vi "Main control_v2.13.vi"() -> ()   [LabVIEW 2015]
panel:
  out "millisecond timer value":u32
  in  "Snap Number Counting":dbl=49.0
  out "Movie Point cluster":cluster{"Movie Y":dbl[], "Movie X":dbl[]}={"Movie Y"=[-12.0, -12.0, -12.0, 0.323, 0.323, 0.323, 0.323, 0.323, 0.3734, 0.3734, 0.3734, 0.3734, 0.3734, 0.3734, 0.3734, 0.3734, 0.3734, 0.3734, 0.8702, 0.8702, 0.8702, 0.8702, 0.8702, 0.8702, 1.1907, 1.1907, 1.1907, 1.1907, 1.1907, 1.1782, 1.1782, 1.1782, 1.1782, 1.1782, 1.1782, 1.1782, 1.1782, 0.273, 0.273, 0.273, 2.5485, 2.5485, 2.5485, 2.5485], "Movie X"=[-1.0, -1.0, -1.0, 4.5272, 4.5272, 4.5272, 4.5272, 4.5272, 5.9944, 5.9944, 5.9944, 5.9944, 5.9944, 5.9944, 5.9944, 5.9944, 5.9944, 5.9944, 5.5544, 5.5544, 5.5544, 5.5544, 5.5544, 5.5544, 5.661, 5.661, 5.661, 5.661, 5.661, 6.0676, 6.0676, 6.0676, 6.0676, 6.0676, 6.0676, 6.0676, 6.0676, 5.2601, 5.2601, 5.2601, 2.0517, 2.0517, 2.0517, 2.0517]}
  out "Movie Point  Y Array":dbl[](array[numeric])=[-12.0, -12.0, -12.0, 0.323, 0.323, 0.323, 0.323, 0.323, 0.3734, 0.3734, 0.3734, 0.3734, 0.3734, 0.3734, 0.3734, 0.3734, 0.3734, 0.3734, 0.8702, 0.8702, 0.8702, 0.8702, 0.8702, 0.8702, 1.1907, 1.1907, 1.1907, 1.1907, 1.1907, 1.1782, 1.1782, 1.1782, 1.1782, 1.1782, 1.1782, 1.1782, 1.1782, 0.273, 0.273, 0.273, 2.5485, 2.5485, 2.5485, 2.5485]
  out "Movie Point  X Array":dbl[](array[numeric])=[-1.0, -1.0, -1.0, 4.5272, 4.5272, 4.5272, 4.5272, 4.5272, 5.9944, 5.9944, 5.9944, 5.9944, 5.9944, 5.9944, 5.9944, 5.9944, 5.9944, 5.9944, 5.5544, 5.5544, 5.5544, 5.5544, 5.5544, 5.5544, 5.661, 5.661, 5.661, 5.661, 5.661, 6.0676, 6.0676, 6.0676, 6.0676, 6.0676, 6.0676, 6.0676, 6.0676, 5.2601, 5.2601, 5.2601, 2.0517, 2.0517, 2.0517, 2.0517]
  out "Snap Point cluster":cluster{"Snap Y":dbl[], "Snap X":dbl[]}={"Snap Y"=[-12.0, 0.323, 0.8702, 1.1907, 2.5485], "Snap X"=[-1.0, 4.5272, 5.5544, 5.661, 2.0517]}
  out "Snap Point  Y Array":dbl[](array[numeric])=[-12.0, 0.323, 0.8702, 1.1907, 2.5485]
  out "Snap Point  X Array":dbl[](array[numeric])=[-1.0, 4.5272, 5.5544, 5.661, 2.0517]
  out "Stage XY Cluster":cluster{"Stage Y ":dbl[], "Stage X":dbl[]}
  in  "Previous Light control":T1={"Filter Set"=0, "Lasers DO"=[FALSE, FALSE, FALSE, FALSE, FALSE, FALSE], "Lasers AO (V)"=[0.3, 0.3, 0.3, 0.3, 0.3, 0.3], "LED"=FALSE, "Global"=FALSE} {"Lasers AO (V)" min=0.0 max=5.0 step=0.01 scale=0.0..5.0 scale format="%#1.2f"; "Filter Set" items=["R-QuasAr", "R-Cy5", "R-mCherry", "R-mOrange", "R-GFP", "R-CFP/DAPI", "R-BFP", "R-LED", "SDC-Cy5", "SDC-mCherry", "SDC-mO2", "SDC-GFP", "SDC-CFP/DAPI", "SDC-BFP", "SDC-LED"]}
  out "Image Info":T2={"Status"="Camera live", "scale bar (μm)"=65.0, "Image"=array512x512[262144 elements], "Histogram"={"max value"=6837, "mean"=2967, "min value"=1682, "Histogram"={"X Values"=[1707.775, 1759.325, 1810.875, 1862.425, 1913.975, 1965.5249999999999, 2017.0749999999998, 2068.625, 2120.175, 2171.7250000000004, 2223.2750000000005, 2274.8250000000007, 2326.375000000001, 2377.925000000001, 2429.4750000000013, 2481.0250000000015, 2532.5750000000016, 2584.125000000002, 2635.675000000002, 2687.225000000002, 2738.7750000000024, 2790.3250000000025, 2841.8750000000027, 2893.425000000003, 2944.975000000003, 2996.5250000000033, 3048.0750000000035, 3099.6250000000036, 3151.175000000004, 3202.725000000004, 3254.275000000004, 3305.8250000000044, 3357.3750000000045, 3408.9250000000047, 3460.475000000005, 3512.025000000005, 3563.5750000000053, 3615.1250000000055, 3666.6750000000056, 3718.225000000006, 3769.775000000006, 3821.325000000006, 3872.8750000000064, 3924.4250000000065, 3975.9750000000067, 4027.525000000007, 4079.075000000007, 4130.625000000007, 4182.1750000000075, 4233.725000000008, 4285.275000000008, 4336.825000000008, 4388.375000000008, 4439.925000000008, 4491.475000000009, 4543.025000000009, 4594.575000000009, 4646.125000000009, 4697.675000000009, 4749.2250000000095, 4800.77500000001, 4852.32500000001, 4903.87500000001, 4955.42500000001, 5006.97500000001, 5058.525000000011, 5110.075000000011, 5161.625000000011, 5213.175000000011, 5264.725000000011, 5316.2750000000115, 5367.825000000012, 5419.375000000012, 5470.925000000012, 5522.475000000012, 5574.025000000012, 5625.575000000013, 5677.125000000013, 5728.675000000013, 5780.225000000013, 5831.775000000013, 5883.3250000000135, 5934.875000000014, 5986.425000000014, 6037.975000000014, 6089.525000000014, 6141.075000000014, 6192.625000000015, 6244.175000000015, 6295.725000000015, 6347.275000000015, 6398.825000000015, 6450.3750000000155, 6501.925000000016, 6553.475000000016, 6605.025000000016, 6656.575000000016, 6708.125000000016, 6759.675000000017, 6811.225000000017], "Histogram: h(x)"=[41, 1173, 7166, 18548, 38399, 52796, 41857, 18688, 5319, 2347, 1597, 1341, 1106, 993, 836, 742, 658, 618, 542, 497, 461, 457, 375, 411, 351, 350, 349, 333, 306, 267, 290, 314, 267, 266, 245, 236, 239, 226, 215, 236, 207, 198, 220, 203, 183, 203, 193, 233, 207, 201, 200, 213, 225, 205, 234, 233, 217, 223, 226, 234, 205, 188, 191, 179, 188, 151, 157, 160, 126, 106, 88, 73, 65, 45, 58, 56, 47, 62, 59, 57, 75, 127, 241, 563, 1192, 2513, 4244, 6503, 8198, 8910, 8047, 6139, 3870, 2034, 948, 358, 135, 51, 13, 6]}}, "Scale Info"={"Pixel size (nm)"=650.0, "Total x width (μm)"=332.8, "Total y width (μm)"=332.8}, "Camera View indicator"=array512x512[262144 elements], "max frame rate (Hz)"=100.0}
  out "log path":path=path "C:/Register info of scope/201810 regiser info.txt"
  out "ROI cursor":T3={"Bin"=4, "ROI"={"x offset"=0, "y offset"=0, "x width"=512, "y width"=512}} caption="ROI" {"ROI"."x offset" min=1 max=512 step=1; "ROI"."y offset" min=1 max=512 step=1; "ROI"."x width" min=1 max=512 step=1; "ROI"."y width" min=1 max=512 step=1; "Bin" items=["1x1"=1, "2x2"=2, "4x4"=4]}
  out "Previous ROI":T3={"Bin"=4, "ROI"={"x offset"=0, "y offset"=0, "x width"=512, "y width"=512}} caption="ROI" {"ROI"."x offset" min=1 max=512 step=1; "ROI"."y offset" min=1 max=512 step=1; "ROI"."x width" min=1 max=512 step=1; "ROI"."y width" min=1 max=512 step=1; "Bin" items=["1x1"=1, "2x2"=2, "4x4"=4]}
  in  "Tab":T4(tab)
  in  "Load Excel to table":bool
  in  "Write table to excel":bool
  in  "Goto destination":bool
  in  "Clear Table":bool
  in  "Track on?":bool
  in  "Stage on?":bool
  out "SDC initialized":bool
  in  "Confocal on?":bool
  in  "Camera on?":bool
  out "Stage initialized":bool
  out "Camera initialized":bool[](array[boolean])
  in  "Light control":T1={"Filter Set"=7, "Lasers DO"=[FALSE, FALSE, FALSE, FALSE, FALSE, FALSE], "Lasers AO (V)"=[0.3, 0.3, 0.3, 0.3, 0.3, 0.3], "LED"=TRUE, "Global"=FALSE} {"Lasers AO (V)" min=0.2 max=5.0 step=0.01 scale=0.0..5.0 scale format="%#1.2f"; "Filter Set" items=["R-QuasAr", "R-Cy5", "R-mCherry", "R-mOrange", "R-GFP", "R-CFP/DAPI", "R-BFP", "R-LED", "SDC-Cy5", "SDC-mCherry", "SDC-mO2", "SDC-GFP", "SDC-CFP/DAPI", "SDC-BFP", "SDC-LED", "SDC-Cy3", "R-pHlamingo", "R-dualview", "R-mO2_no laser"]}
  in  "Confocal scanner":T5={"SDC shutter"=FALSE, "Filter wheel"=6, "FW speed"=3, "Disk spinning"=FALSE, "Disk speed (rpm)"=3000.0} {"Disk speed (rpm)" min=1500.0 max=10000.0; "FW speed" min=1 max=5 step=1; "Filter wheel" items=["CFP"=1, "GFP"=2, "mCherry"=3, "Alexa-647"=4, "OFP"=5, "empty"=6]}
  in  "Stage-Ctrl":T6={"Console"={"L"=FALSE, "R"=FALSE, "FWD"=FALSE, "BACK"=FALSE}, "Step Width [mm]"=0.2, "Destination [mm]"=[0.0, 0.0], "Move "=FALSE} {"Destination [mm]" format="%_6g"; "Step Width [mm]" min=0.0 format="%_6f"}
  out "Stage Status":T7={" Current Position"=[-1.0, -12.0, 0.0], "Number of Axis"=3, "ILSID"=1}
  in  "Camera Ctrl":T8={"Chosen Camera"=1, "ROI selection"=0, "Live"=FALSE, "ROI define"=FALSE, "Snap"=FALSE, "ROI update"=FALSE, "ROI previous "=FALSE, "ROI"={"Bin"=4, "ROI"={"x offset"=0, "y offset"=0, "x width"=512, "y width"=512}}, "Exposure (ms)"=100.0, "Symmetrical"=TRUE, "Autoscale"=TRUE, "Scale"={"Scale.Min"=374, "Scale.Max"=483}} {"Scale"."Scale.Max" min=1 max=5000 step=1; "Scale"."Scale.Min" min=1 max=5000 step=1; "Exposure (ms)" min=1.0 max=5000.0 step=1.0; "ROI"."ROI"."x offset" min=1 max=512 step=1; "ROI"."ROI"."y offset" min=1 max=512 step=1; "ROI"."ROI"."x width" min=1 max=512 step=1; "ROI"."ROI"."y width" min=1 max=512 step=1; "ROI"."Bin" items=["1x1"=1, "2x2"=2, "4x4"=4]; "ROI selection" items=["Full ROI", "Central quad", "Confocal", "Patch 500", "Patch 1000", "Patch 484", "Patch 484 full X", "Line scan 2.5KHz", "Confocal_2", "patch 1000 wide", "patch 671", "DV2"]; "Chosen Camera" items=["Left", "Right"]}
  in  "TI-Ctrl":T9={"Obj"=2, "Cube Bottom"=4, "Cube Top"=6, "PFS-Ctrl"={"PFS IO"=FALSE, "PSF Err"=FALSE, "PSF Pos"=0}, "Z-Ctrl"={"Z-pos"=500.85, "Home"=FALSE, "Sensitivity"=1}, "Condenser"=2, "Lightpath"=enum."R100"} {"Condenser" items=["A"=1, "DICN2"=2, "- empty 3 -"=3, "- empty 4 -"=4, "- empty 5 -"=5, "- empty 6 -"=6]; "Z-Ctrl"."Sensitivity" min=1 max=3 step=1 scale=1.0..3.0; "PFS-Ctrl"."PSF Pos" scale=0.0..16400.0; "Cube Top" items=["Quad-O"=1, "Quad-R"=2, "empty"=3, "empty"=4, "empty"=5, "DIC"=6]; "Cube Bottom" items=["GFP"=1, "RFP"=2, "mO2"=3, "empty"=4, "CFP"=5, "Cy5"=6]; "Obj" items=["20x/.75 Dry PFS"=1, "40x/1.3 Oil PFS"=2, "60x/1.4 Oil PFS"=3, "- empty 4 -"=4, "- empty 5 -"=5, "40x/0.6 Dry PFS"=6]}
  in  "Scope on?":bool
  out "Ti-E initialized":bool
  in  "stop program":bool
  in  "Record Table":string[][](table)=[["", "", "", "", ""], ["", "", "", "", ""], ["", "", "", "", ""], ["", "", "", "", ""], ["", "", "", "", ""], ["", "", "", "", ""], ["", "", "", "", ""], ["", "", "", "", ""], ["", "", "", "", ""], ["", "", "", "", ""], ["", "", "", "", ""], ["", "", "", "", ""], ["", "", "", "", ""], ["", "", "", "", ""], ["", "", "", "", ""], ["", "", "", "", ""], ["", "", "", "", ""], ["", "", "", "", ""], ["", "", "", "", ""], ["", "", "", "", ""], ["", "", "", "", ""], ["", "", "", "", ""], ["", "", "", "", ""], ["", "", "", "", ""], ["", "", "", "", ""], ["", "", "", "", ""], ["", "", "", "", ""], ["", "", "", "", ""], ["", "", "", "", ""], ["", "", "", "", ""], ["", "", "", "", ""], ["", "", "", "", ""], ["", "", "", "", ""], ["", "", "", "", ""], ["", "", "", "", ""], ["", "", "", "", ""], ["", "", "", "", ""], ["", "", "", "", ""], ["", "", "", "", ""], ["", "", "", "", ""], ["", "", "", "", ""], ["", "", "", "", ""], ["", "", "", "", ""], ["", "", "", "", ""], ["", "", "", "", ""], ["46", "01/25 18:48:27", "-1.0000", "-12.0000", "Movie"], ["47", "01/25 18:49:17", "-1.0000", "-12.0000", "Movie"], ["48", "01/25 20:04:01", "-1.0000", "-12.0000", "Movie"], ["49", "05/17 17:14:13", "-1.0000", "-12.0000", "Image"]]
  out "Stage Trajec":cluster{"Value":dbl[], "Value":dbl[]}[](graph)=[{"Value"=[], "Value"=[]}, {"Value"=[-12.0, 0.323, 0.8702, 1.1907, 2.5485], "Value"=[-1.0, 4.5272, 5.5544, 5.661, 2.0517]}, {"Value"=[-12.0, -12.0, -12.0, 0.323, 0.323, 0.323, 0.323, 0.323, 0.3734, 0.3734, 0.3734, 0.3734, 0.3734, 0.3734, 0.3734, 0.3734, 0.3734, 0.3734, 0.8702, 0.8702, 0.8702, 0.8702, 0.8702, 0.8702, 1.1907, 1.1907, 1.1907, 1.1907, 1.1907, 1.1782, 1.1782, 1.1782, 1.1782, 1.1782, 1.1782, 1.1782, 1.1782, 0.273, 0.273, 0.273, 2.5485, 2.5485, 2.5485, 2.5485], "Value"=[-1.0, -1.0, -1.0, 4.5272, 4.5272, 4.5272, 4.5272, 4.5272, 5.9944, 5.9944, 5.9944, 5.9944, 5.9944, 5.9944, 5.9944, 5.9944, 5.9944, 5.9944, 5.5544, 5.5544, 5.5544, 5.5544, 5.5544, 5.5544, 5.661, 5.661, 5.661, 5.661, 5.661, 6.0676, 6.0676, 6.0676, 6.0676, 6.0676, 6.0676, 6.0676, 6.0676, 5.2601, 5.2601, 5.2601, 2.0517, 2.0517, 2.0517, 2.0517]}]
  in  "Number":dbl
  out "Color Acquiring":bool
  out "T Acquired Progress":i32(slide)=100 scale=0.0..100.0
  in  "Load from Exel (For XY Scan)":bool
  in  "Load from table (For XY Scan)":bool
  in  "Generate Tiling":bool
  in  "XY Scan List":string[][](table)
  in  "Cal step num":bool
  in  "Cal step size":bool
  in  "Define 1":bool
  in  "Define 2":bool
  in  "Z-Stack":T10={"Z end"=1000.0, "Step Num"=10, "Step Size"=-200.0, "Z0"=3000.0, "z-stack?"=FALSE}
  in  "MD acquisition":bool
  in  "Channel settings":T11={"Take?"=[FALSE, TRUE, FALSE, FALSE], "Channel"=[1, 2, 3, 4], "Exposure time (msec)"=[100.0, 100.0, 100.0, 100.0], "Cumulation"=[1, 1, 1, 1], "Name"=["Cy5", "mCh", "GFO", "CFP"]} {"Exposure time (msec)" format="%0.0f"; "Channel" items=["R-QuasAr", "R-Cy5", "R-mCherry", "R-mOrange", "R-GFP", "R-CFP/DAPI", "R-BFP", "R-LED", "SDC-Cy5", "SDC-mCherry", "SDC-mO2", "SDC-GFP", "SDC-CFP/DAPI", "SDC-BFP", "SDC-LED", "SDC-Cy3", "R-pHlamingo"]}
  in  "Period (s)":u32=3
  in  "Timelapse Cycles":i32=100 caption="# Cycles"
  in  "Timelapse?":bool
  out "Timelapse Acquired":i32=100 caption="Acquired"
  out "Timelapse Time (s)":dbl=297.037 caption="Time (s)"
  in  "Movie frame rate (Hz)":dbl=10.0 format="%0.0f"
  out "Frames Recorded":i32=1000
  in  "Stream movie":bool
  in  "# frames":i32=1000
  in  "Total time (sec)":dbl=100.0 min=1.0 max=5000.0 step=1.0
  out "Elapsed time (sec)":dbl=100.541 min=1.0 max=5000.0 step=1.0
  in  "Base folder":path=path "C:/Users/ZouOptics/Desktop/test"
  in  "Sub-folder":string="patch"
  out "Full path":path=path "C:/Users/ZouOptics/Desktop/test/200401_patch"
  in  "XY tiling":T12={"Tiling?"=FALSE, "YY/XX"=[1, 1], "X0Y0"=[-1.0, -12.0, 0.0]}
  in  "Excel Loading Path":path=path "X:/Data and analysis/Sicong Wang/Fluorescence Images/test.xlsx"
  out "Z Stack Aquired":i32(slide)=10 scale=0.0..1.0
  out "Stage Trajec for tiling":cluster{"Value":dbl[], "Value":dbl[]}[](graph)
  in  "Ranking":u16(ring) items=["Identical", "Minimum Distance", "Snake"]
  in  "Waveform channels":T13={"Lasers"=[FALSE, TRUE, FALSE, TRUE, FALSE, FALSE], "Patch"=FALSE, "Camera Output"=TRUE}
  out "Lasers DO waveform":digitalwaveform[](graph)=[{"t0"=timestamp(0 s since 1904-01-01), "dt"=0.001, "Y"={"transitions"=[0, 10000, 13000, 19999], "data"=[[0], [1], [0], [0]]}}, {"t0"=timestamp(0 s since 1904-01-01), "dt"=0.001, "Y"={"transitions"=[0, 10000, 19999], "data"=[[1], [0], [0]]}}]
  out "Lasers AO waveform":waveform(dbl)[](graph)=[{"t0"=timestamp(0 s since 1904-01-01), "dt"=0.001, "Y"=array[20000 elements]}, {"t0"=timestamp(0 s since 1904-01-01), "dt"=0.001, "Y"=array[20000 elements]}]
  in  "Load waveform":bool
  in  "Waveform info":T14={"Waveform folder"=path "C:/Users/ZouOptics/Desktop/MATLAB codes new/MATLAB codes/ephys waveforms_new/Mito and ER/dual-color/waveform003_561_3s 3min test", "Exposure time (ms)"=200.0} {"Exposure time (ms)" format="%0.5f"}
  out "AI Waveform":cluster{"xo":i32, dbl, "data":dbl[][]}(graph)={"xo"=0, 0.001, "data"=[]}
  in  "Run waveform":bool
  out "Patch Ex. Command AO waveform":waveform(dbl)(graph)
  out "Seal test DAQ params":T15={"samples"=40000, "Duration (sec)"=2.2222222222222223, "Downsampling factor"=2000.0}
  out "Patch seal test waveform":waveform(dbl)(graph)={"t0"=timestamp(0 s since 1904-01-01), "dt"=5.555555555555556e-05, "Y"=array[40000 elements]}
  in  "Save patch param":bool
  in  "Pipet tuning parameters":T16={"Amplitude (mV)"=5.0, "Number of repeats"=20, "DAQ rate (Hz)"=18000.0, "Frequency (Hz)"=9.0}
  in  "Test patch":bool
  out "Patch output":cluster{"xo":i32, dbl, "data":dbl[][]}(graph)={"xo"=0, 5.555555555555556e-05, "data"=array2x40000[80000 elements]}
  out "Average I-t curve":cluster{"xo":i32, dbl, dbl[]}(graph)={"xo"=0, 5.555555555555556e-05, [29.880051543579523, 31.53110578210508, 83.18090907512509, 162.0368645993861, 229.6898135163709, 288.6606341781445, 343.08904187423104, 388.8031046956136, 432.56006420735736, 429.5156789314345, 389.7776239991212, 355.78201712503267, 329.13964160904936, 306.7416838810265, 288.4109564887366, 272.60916075180677, 258.4745269911103, 245.11307022374868, 234.37719239460748, 224.51919115018714, 215.35382740090955, 206.6636454502011, 199.34263011111548, 192.6498209835887, 186.06976642635385, 179.43333449516217, 174.21439286866243, 168.7377258559817, 163.79261775420784, 158.65421491547735, 154.4661750789392, 150.4794835552285, 146.3397675650155, 141.9987034936742, 139.3731246948087, 136.7636538843144, 133.12328092961516, 130.39300120942653, 127.58218215818046, 125.35124577902424, 122.21826996530297, 119.06918641850369, 117.3456469811447, 115.89594095422709, 114.10797017306047, 111.50655329307857, 109.57361178840823, 107.18965080041876, 105.35335650344665, 102.92912592909049, 102.10762590319547, 101.1008856426019, 100.06192974722902, 98.96659640362893, 97.00143950529804, 95.9946992448826, 94.87520399068636, 93.32885099805317, 91.07375276207976, 89.26967425849605, 88.464282088203, 87.36894864979442, 86.14475245555671, 84.88028669189909, 83.79300728992337, 82.64129641270459, 82.10168356131484, 81.30434527026028, 80.03987957079214, 80.11236480548284, 79.13784014631288, 78.29217829154415, 77.06798205802154, 75.22363383162443, 74.1766240107049, 74.00749150960763, 73.31485423356304, 73.04907478387904, 71.53493743348268, 71.22888838598573, 71.19667263278379, 70.03690780108447, 69.72280488470987, 69.42480969761857, 68.67579487408646, 68.2892065594221, 68.2650448000469, 67.53213783229249, 66.21129465198342, 65.04347590641633, 64.47970136823793, 63.738740585923004, 63.31188273674811, 63.06221124272047, 63.247451399716546, 62.50649048668514, 61.548073809976344, 61.5722356830505, 61.773583749751516, 61.29034841296893, 60.30776992217408, 59.252706103313066, 58.970818812926204, 59.7117796957233, 59.5345934070801, 58.45536777888253, 57.56138251425965, 56.96539234266666, 56.38550986897839, 55.6042793899474, 55.20158318736758, 55.282122384674594, 55.443200858403316, 54.97607337010223, 54.621700717145416, 54.90358802777563, 54.35592129460591, 53.42972030928748, 54.372029148842316, 53.49415159115674, 53.20421033522031, 52.2457936059895, 52.1733082482847, 52.03639155042868, 51.22294539942853, 51.79477386875771, 50.97327375999859, 51.118244339124836, 50.498092398621225, 50.820249284974935, 50.5142002256432, 49.22557270943183, 49.096709956802705, 49.41081292650386, 48.790660927446204, 48.72622958625065, 49.563837544108324, 49.71686213809168, 49.233626722017284, 48.492665888390036, 48.782607126502214, 47.62284235318299, 48.218832605660864, 48.44434242434597, 47.075175695308104, 46.94631299135462, 47.759759177278106, 46.56777864142779, 46.61610214009233, 46.18119035155284, 45.99595015189401, 45.5207686921585, 45.14223428471252, 45.383851918860685, 45.810709817016004, 45.214719602674585, 44.32073419846522, 43.990523364405924, 44.844239111123336, 45.64157743347831, 44.455050003834835, 42.9998909052363, 43.475072280525744, 43.7730674181327, 44.04690079066772, 42.99989087004219, 43.08848400218545, 42.66968004658263, 42.85492020248559, 42.981182076403115, 42.49249376565697, 42.532763411615534, 42.33946927737113, 42.017312373726895, 41.727371189308236, 42.548871213651026, 42.78243503281226, 41.815964370657404, 41.67099377457743, 40.74479272430971, 41.33272903397758, 41.73542518986539, 40.68841531947955, 40.68036138479713, 40.66425355122241, 41.67099382135634, 40.7689545273035, 40.62398400796506, 40.124640818844185, 39.83469956321526, 40.29377314835857, 39.923292709326375, 39.69778287373534, 40.09242502006745, 40.1165867506579, 39.66556710850734, 39.02385421340008, 38.449424886197086, 39.10179251143014, 39.907184658568255, 40.317934715770775, 39.82664548999167, 39.593081728282165, 39.58502783256104, 39.45616501104882, 39.480326789591686, 39.97966992283737, 39.81053760662116, 38.83601302550602, 38.505802172044845, 38.22391489382652, 39.144662908881884, 39.11790028828071, 38.417209103882385, 39.09373859598984, 38.71520425745377, 38.44942479293209, 38.64271891646013, 38.256130738306, 37.780949304210154, 37.99035129543478, 37.23328257384945, 37.692356207891606, 37.78094938449001, 37.72457190122881, 37.57154738570286, 38.00645923224989, 37.5312778137379, 37.87759644612147, 37.90981213503523, 37.84538073068071, 38.15948368901419, 38.39304737004068, 38.18364539082346, 37.716517944756625, 37.305767891483846, 36.62923834581099, 36.830586380562174, 36.28291974002178, 36.62923835578246, 36.99971871503225, 37.24133642280873, 37.67624822587764, 35.888277488077094, 36.52453727615889, 37.82121877366858, 37.080257998223054, 36.677561870857566, 35.63055195367037, 36.47621377440903, 36.556752962450304, 36.817079377736675, 35.87216966309211, 35.45336570834543, 35.75136084508183, 35.77552256150283, 36.06546377068963, 36.21848834436996, 35.831900084497946, 36.64534623485339, 36.49232172114825, 36.049356061223044, 35.86411580752019, 36.31773634513554, 36.38762076053971, 36.162110948839185, 35.1714785375557, 35.80228530827381, 36.221089318174705, 36.05740998819331, 36.234596259515136, 35.131208907727846, 35.93660112849782, 36.98361098547167, 36.41983640610623, 35.63055202080656, 35.70303727905714, 36.05740981623031, 35.92854705422721, 35.35671863758792, 35.686929417746775, 36.02519411870366, 36.04130196862305, 35.80513734973099, 35.853460911422225, 35.11510086032629, 34.656027278390894, 34.478840946772294, 34.57548806003412, 35.1527696265201, 36.00103227632688, 35.30034103329851, 34.53521850111496, 34.865429279655665, 35.6627675893214, 36.685615730073295, 35.703037251838076, 34.054584022453355, 35.68953027356607, 35.83995400784085, 35.2439637863511, 35.04261567853634, 34.56198119625272, 34.79814587027351, 34.970130472238445, 35.01040010245213, 34.67473618343048, 34.73916762344858, 35.24656475502339, 35.13380981144574, 34.124468602443265, 34.41701062047655, 34.61835868531181, 35.22240285144073, 35.0023460751858, 35.211748027071806, 34.23722340304511, 33.826473384960565, 34.58354206554848, 33.227882236903135, 33.10707340456224, 33.823872504398196, 33.81036547173107, 33.38090675630988, 33.268151809626936, 33.260097906803445, 33.42117637060354, 34.17019112956772, 34.79839701045026, 34.98363723051565, 33.89090473781439, 32.51368406091628, 33.48820861717215, 34.0680910149931, 32.4305439113784, 32.88961752023779, 33.47755388152356, 33.32713026373934, 33.35129198579972, 32.85740184312288, 34.50845598814005, 33.576801900497294, 34.28814790525812, 33.29491457286375, 33.77814996396535, 34.084199078645284, 34.272040140362186, 33.23308420063638, 33.60356458985568, 33.98469978568426, 33.79685868804102, 33.98209888749632, 33.353892963877016, 33.28686075071024, 33.10707355187398, 32.89767152720865, 33.539133089710276, 33.49886349447493, 33.55264005260219, 33.78905597985785, 33.93117437541065, 34.18084601030195, 32.916380133871534, 32.2559585132527, 32.58616932156536, 33.21177438100168, 33.576801728530626, 33.52847818346761, 33.77814984665877, 33.63863227243345, 33.778149832967486, 34.97818427338362, 34.680189157321486, 33.75944114678964, 33.93117436078832, 33.82387255658079, 33.34063724504784, 33.061350832666015, 32.33649783263258, 32.86000283828841, 32.46536067034913, 32.70957917530949, 32.87611066749775, 32.60227733217256, 33.431831332440225, 33.20632151462504, 32.67736351117674, 32.63709392257487, 33.015628287713305, 33.86934405322023, 32.99952040978686, 33.50691746633257, 33.03458822506665, 33.2923137505889, 33.25464502047356, 32.857401940524845, 33.13383614177684, 32.7230860846945, 33.51782354473178, 33.16865260615072, 33.25464488004037, 33.81036555020686, 34.156684233437915, 32.97821065828864, 32.86000265489926, 32.70697814823967, 32.972757554955756, 32.51108314372694, 32.7929704134161, 33.12032905957902, 32.27466722926702, 32.19412805134144, 31.896132920558067, 33.70826546725869, 33.89090476099264, 33.69761065497293, 33.190213613064564, 33.20632142585998, 32.98601334906449, 32.741794880060795, 32.28817436835036, 31.7646694066269, 32.50823109621544, 32.46796151596167, 31.340412406565125, 31.03436337556969, 31.56852313913503, 32.1403515811195, 32.63969476829801, 32.5485007324532, 32.30688307985144, 32.03304972077633, 32.53499374600606, 32.36065966647435, 32.59942512105814, 32.196980288638684, 31.635806586574443, 31.235711320411408, 32.306882974958725, 32.15125757030716, 31.944456465814945, 31.82104673328156, 31.77272321662366, 32.26946549432704, 32.23724981873913, 31.737906623218368, 31.853262418874255, 32.24790456433751, 32.34195074938029, 32.280120284066754, 31.517598539524357, 30.65582887774616, 30.81975955493944, 31.619698723654817, 31.104247722579014, 30.9351153357554, 32.213088086020925, 31.456019436396677, 31.73790676935194, 32.75270098238981, 32.607730407576675, 31.41574989477592, 31.531105711919206, 31.18478704877367, 30.919007585808018, 31.587483151770833, 31.12840961645485, 31.179334033517204, 30.35523306530969, 31.16607837413623, 31.689583307138683, 32.108387280662065, 31.44796563489925, 31.665421495347566, 32.74464701592463, 32.30168130493072, 32.143203734291866, 32.07071842025991, 31.50434292991561, 32.01434091344282, 32.304282138445515, 31.555267359288916, 31.61164479053598, 31.772723234375118, 31.73245361272506, 32.03850264630772, 31.866769372738997, 31.133862486566013, 31.378080986518274, 31.43445846323188, 31.297541794396263, 31.007600642087446, 31.426404609191703, 31.305595773656705, 32.47341445327548, 31.68958317094127, 31.708291949137532, 31.571375276751702, 31.41029680286774, 31.735054573538918, 31.40224294857394, 32.25855958429945, 32.12709595526592, 32.014341055350485, 32.548500821840065, 31.563321429034854, 32.06266464659797, 31.557868392452068, 31.735054666392447, 32.06786634854822, 32.21829000105026, 31.43445864129108, 30.90550055484247, 31.565922199383742, 32.74439577108956, 32.80622627683914, 31.603590937293813, 31.227657404087406, 31.33235844208331, 31.72439980138405, 32.20763509026013, 30.97538496036247, 31.265326158285603, 30.910953532773906, 31.44796545801619, 31.70569100495986, 31.25727220550966, 30.68544366007619, 31.69763699291113, 32.5568058683679, 30.967331024342286, 31.257272228962393, 31.461221169015328, 31.51759864918303, 31.99823311270946, 31.684130142679276, 30.516311463134777, 29.914868169545862, 30.9779858757755, 31.99823312580485, 30.508257520275055, 31.348466316509402, 31.54721343780208, 31.89353212832518, 31.635806689247424, 31.888079136450628, 31.710892859029546, 32.46796154145252, 32.20218214144233, 31.531105730372392, 31.799485974142833, 31.896133044845413, 31.549814385193596, 31.633205796520286, 31.638658809288323, 33.034588244313646, 32.811679271974256, 32.63994604569917, 32.62383813951148, 31.947308642051155, 31.882877272238257, 31.705691012757082, 31.59553694057632, 31.0639780411176, 32.245303741456134, 31.327156646376245, 31.98497738706063, 31.754014493314706, 32.75815391380303, 31.756615378639385, 31.512396844714164, 31.3674262422325, 32.77140960429028, 31.533957751273974, 30.77688911611326, 31.456019463499782, 31.657367500176907, 31.778176318456836, 31.893532131794363, 31.327156735270798, 30.540473205208805, 30.06529184371326, 30.951223310518714, 30.894845837431127, 31.096193885174088, 30.637120368779996, 31.7243998764309, 31.257272371463607, 31.788831245688037, 31.28948811045239, 32.135149885863015, 32.172818584434474, 31.286887102411967, 31.810392069406326, 31.713745016952483, 31.57137528962488, 30.908352738668093, 31.327156703970836, 31.402242833385337, 31.563321255214674, 31.724399686599444, 32.24790466817393, 32.164764616467565, 30.983438868015334, 30.725713302903657, 31.845208507857382, 32.90572538454016, 32.680215511032365, 31.69763699732868, 31.635806530539316, 32.39287522201038, 32.24245161694785, 32.1834733143828, 32.46536063396243, 33.11772828602879, 32.45730665126147, 32.078772309469485, 31.40224285401661, 31.57942916481285, 31.20349572746602, 31.450566465836673, 31.32975760514152, 31.200894856826146, 32.296228336044614, 31.281434118783995, 30.878737999785105, 30.580742902576137, 31.68673114847933, 33.01562831400659, 31.131010466554596, 30.631667235535073, 31.496289125427666, 31.614245797440212, 31.211549671241873, 31.370027177893874, 30.991492850089656, 30.833015316745822, 31.24376532947516, 31.692184034043294, 30.572688825384922, 31.5552673754126, 31.217002640458894, 30.96733103585858, 31.434458503688436, 31.659968271830152, 32.11904192419194, 31.120355544607026, 30.830414336323074, 30.564634884949417, 30.95122310879727, 31.966017358462167, 31.47732895837401, 30.148431847342014, 30.446426980577804, 30.94577015502743, 31.023708412930922, 31.80493890640768, 30.972532773535328, 31.713493666093385, 32.25855949492659, 31.95251043134216, 31.85326252525323, 31.756615505137205, 31.549814382487217, 31.020856402695518, 31.979273100828895, 32.39002319769506, 31.90418701928753, 32.36586145638116, 31.84235650087687, 32.06526542756272, 30.628815052346862, 29.839782002889855, 31.077233852323314, 32.13229763381895, 32.02499571929181, 29.941630711558663, 29.925522915681533, 29.91486810586367, 30.28820071066647, 30.798198666447885, 29.815620191529806, 30.258585876990605, 31.12035556143148, 30.545926225824854, 30.352632087120078, 31.21440175147005, 31.36482536311301, 30.801050802731506, 31.429256736566643, 31.520450751781844, 30.862630039038468, 31.324304499306724, 31.278833159463602, 30.956676254443614, 30.3604347147787, 30.476041848199696, 30.894845809018012, 30.701551671752554, 30.999546815003757, 31.24116453355479, 32.465360708866044, 32.20763519921539, 31.76727034656866, 31.4451134538732, 31.72700076064497, 30.824961454822606, 30.76053008060773, 31.3001428842445, 31.286635957481643, 31.018255638184936, 31.710892845150802, 31.54721353543418, 31.82910086033523, 31.4692751855601, 31.72960156848901, 31.61424578852162, 31.55786830228545, 31.434458571204658, 30.516311420978596, 30.476041797680725, 30.629066321367187, 30.733767290196383, 30.451880022493715, 29.65194086011632, 30.368739961190006, 30.39550254159804, 29.23313682270737, 30.368739862372074, 31.026560691792298, 31.023708509804553, 31.888079024195022, 31.415498550014895, 31.51499780331629, 30.784691725345446, 29.957989912879217, 30.473440956633922, 31.045269456235964, 30.333672123238326, 29.85588982023964, 30.073345767800177, 30.207410243685274, 30.921608483815014, 29.98995440320599, 30.51891240020253, 31.455768218895308, 31.81559387622767, 31.815593882283984, 30.932263310215863, 31.17128009201948, 32.234397788879974, 31.010201633812333, 31.356520264265857, 31.649313626879547, 32.03044881971146, 31.375480236579005, 31.061377280971858, 31.286635736595215, 30.725713337528504, 31.11775467351705, 31.273380076138007, 31.426404587227502, 31.16867905851295, 30.862630000857155, 30.81430646152824, 31.434458454174607, 30.919007421203926, 30.83041426930373, 30.760529811808027, 30.639721029031293, 30.497351315332885, 31.042417142920748, 31.576576862282476, 31.802086771755153, 31.163226034858297, 31.434458539901552, 31.831701628300063, 30.704152537353597, 30.26663987115451, 30.59685068241315, 30.935115403309197, 30.994093738597435, 31.13101047335675, 29.885253409888595, 30.69064560512269, 31.6571162794837, 31.718946822468943, 30.84367014287102, 31.334959407307114, 32.309484016428925, 31.997981895589806, 31.24921839735877, 31.316250660405387, 31.504091714639518, 31.31885149341779, 30.27729465851637, 31.316250610730435, 31.297541854155217, 31.74570932861524, 30.86523088628539, 31.007600607971025, 31.179333876255754, 30.800799517191457, 30.741821192127794, 30.54592616862937, 31.104247680473215, 31.788831082376014, 31.783378025132098, 30.851975215476774, 30.365887672508354, 30.476041756270966, 30.82756216299985, 31.56046904668177, 32.05981230246551, 31.15517211759733, 31.249218328323703, 30.693497699573225, 30.097507435948625, 31.394188871726715, 30.526966219048095, 29.71897311446653, 31.06397815885712, 30.902899699950478, 30.025022174032827, 29.912267285168575, 30.34717913403877, 29.592711336450922, 29.506719012104046, 30.52696631479477, 30.328219104807474, 30.594249854926087, 30.50565668876932, 30.910953669575182, 31.292340216785878, 31.90158606541657, 30.83846834299569, 31.47472819085728, 31.06943114529891, 31.555267375178683, 31.15257125475, 31.152571236122316, 30.73922032685906, 30.4438260962654, 30.097507394514306, 30.465386966695327, 30.65868110266879, 30.45733306260895, 30.715058585676303, 30.908352699865382, 31.0317623644851, 30.900298765572398, 30.540473145533497, 31.64386047438833, 30.226370196123653, 30.328470367039458, 30.178046702743913, 31.684130129933784, 31.38613500513597, 30.119068410694847, 30.583343710082143, 30.49735145483496, 31.198042662156247, 31.22505669951251, 31.30274374127294, 31.326905528954132, 32.62358699616382, 32.11618989103248, 31.50409184549359, 31.560469251446197, 31.83975567319857, 31.082686970538155, 30.51891238925412, 30.78729266941014, 31.098794773824803, 31.823647750627856, 30.357833871748657, 29.88525333248012, 31.122956480936736, 31.332358484811667, 30.18064757398678, 29.643886974725834, 29.87199765914472, 30.580742811847994, 30.242478044568006, 30.91095356758006, 30.38484772028895, 30.664134121345576, 29.99020551564751, 29.97149677764961, 30.760781181089612, 29.81016705878638, 29.92552289823385, 30.94031707674453, 30.784691652032432, 30.897446617439208, 30.577890634454963, 29.952536889890304, 29.68675743323106, 30.39290172749185, 30.400955672851023, 29.78340454552243, 31.023708580818, 30.398103518369282, 29.383309306915507, 29.694811402401267, 29.19806912103426, 29.689358424338295, 30.263787758332427, 30.71220652952314, 30.505656731183127, 29.99825962923186, 30.725713420318137, 30.23702502470289, 30.011515276599383, 29.313676253034696, 30.145831032122537, 30.548527090833915, 30.650627267976194, 29.437085864190102, 29.297568285526683, 30.121669222761223, 30.467987853632795, 31.748561437058765, 30.355232915444972, 29.756641812719355, 30.38484771031607, 30.935115297572047, 30.57268877968259, 29.598164183607203, 29.54984064495232, 30.234424079699664, 30.411610382671917, 30.132323956261548, 29.055950579773217, 29.968644702536775, 30.61035761548154, 30.457333052694707, 30.578141935818294, 29.933576855493047, 29.598164341679603, 30.24247813231346, 30.237025048291827, 29.603366100870506, 29.587258253062178, 30.752476186866865, 30.376542653985073, 30.328219138044766, 30.70675352766904, 30.875885853142567, 31.251819323134317, 31.05307209489085, 30.100108369400296, 30.242478130987276, 31.579429207528584, 30.465387066590555, 30.36588778766559, 30.688044641234868, 30.218316291768947, 30.99149281941957, 29.332384797535045, 29.300169096758832, 30.250531908373873, 29.936428947409006, 29.82367404783354, 31.00499978308015, 31.206347778490027, 30.64517405374463, 30.988891874451113, 30.46798779128403, 30.046582983070873, 30.462534742357736, 30.7122063872844, 29.45579451175222, 29.00737572075709, 30.9940936394729, 31.195441722935506, 30.49214966993508, 29.69481138318175, 30.188701502252982, 30.269240719057212, 29.662595666793226, 30.02502222200787, 29.823674167948187, 30.132324080321702, 30.245079031228556, 30.196755523816226, 29.51477300648566, 29.939029987192416, 30.81690750522429, 30.58334373538448, 30.20480941376228, 30.494750608848882, 29.952536916967993, 29.501517270797315, 29.273155228096407, 29.020882729501672, 29.904213316044252, 29.743134889524367, 30.116216128197355, 29.68415651199726]}
  out "Patch quality":T17={"Ra (MΩ)"=24.853031315565314, "Rm (MΩ)"=165.59219608794982, "Cm (pF)"=76.83727869217161, "RC constant (msec)"=1.9096392935393605, "Steady state current (pA)"=30.194659640508572}
  in  "Path of saving register":path=path "C:/Register info of scope"
  in  "Calibrate stage":bool
  in  "Hardware Settings":T18={"DAQ ports"={"Lasers DO lines"=["Dev2/port0/line0", "Dev2/port0/line1", "Dev2/port0/line2", "Dev2/port0/line3", "Dev2/port0/line4", "Dev2/port0/line5"], "Lasers AO lines"=["Dev2/ao0", "Dev2/ao1", "Dev2/ao2", "Dev2/ao3", "Dev2/ao4", "Dev2/ao5"], "Patch AO line"="Dev1/ao1", "Patch AI lines 1"={"Patch scaled output"="Dev1/ai13", "Patch 10 V_m "="Dev1/ai8"}, "Camera timing DI"="Dev1/port0/line23", "Dev1 timing DO "="Dev1/port0/line18", "Dev1 trigger source"="/Dev1/PFI0", "Dev2 trigger source"="/Dev2/PFI0", "LED line"="Dev1/port0/line8", "Global Shutter line"="Dev1/port0/line10", "Patch AI lines 2"={"Cell capacitance"="Dev1/ai9", "Mode"="Dev1/ai10", "Frequency"="Dev1/ai11", "Gain"="Dev1/ai12"}}, "Camera Setting"={"Camera Output triger mode setiting"={"Mode"=3, "Polarity"=2, "Period"=0.0005, "Delay"=0.0}, "Camera timing port for trigering"=enum."3"}, "Stage setting"={"Baudrate"=57600, "COM Port"="COM10", "Xmax"=118.5, "Xmin"=15.0, "Ymax"=76.5, "Ymin"=12.2}, "Confocal VISA Setting"="COM1"} {"Camera Setting"."Camera Output triger mode setiting"."Polarity" items=["Negative"=1, "Positive"=2]; "Camera Setting"."Camera Output triger mode setiting"."Mode" items=["Low"=1, "Global Exposure"=2, "Programmable"=3, "Trigger Ready"=4, "High"=5]}
  out "Camera":errorcluster
  out "Stage":errorcluster
  out "Confocal":errorcluster
  out "Camera Info":T19={"Camera Details Array"=[{"Model"="C11440-22C", "Camera ID"="S/N: 003223", "Firmware"="3.20.A"}], "Handle"=0, "Camera in use "={"Model"="C11440-22C", "Camera ID"="S/N: 003223", "Bits"=16}}
  out "Confocal Info":T20
  in  "Ti Control Lib":refnum<k7>
  out "TiE Ref":T21 caption="Ref (can be hidden)"
  out "Previous Bin":u16(ring)=1 caption="Cursor Bin" items=["1x1"=1, "2x2"=2, "4x4"=4]
  # "Nikon Scope v2.13"
  # "Red"
  # "637"
  # "561"
  # "488"
  # "405"
  # "532"
  # "Camera"
  # "Left Camera"
  # "Right Camera"
  # "Stage"
  # "DON'T Close the window \nuntil this button turns RED!"
  # "Stage Status"
  # "Confocal Scanner"
  # "Nikon control"
  # "Red"
  # "637"
  # "561"
  # "488"
  # "405"
  # "532"
  # "X"
  # "Y"
  # "X"
  # "Y"
  # "File I/O"
  # "Multidimensional acquisition"
  # "Stream"
  # "1. Timelapse"
  # "2. Channel"
  # "grey out at start up"
  # "3. XY Scan"
  # "4. Z-stack"
  # "Need to add tiling function"
  # "X"
  # "Y"
  # "Load waveform"
  # "637"
  # "561"
  # "532"
  # "488"
  # "405"
  # "Red"
  # "Pipet tuning"
  # "Need to restart the program if these settings are changed."
  # "Trigger source: /Dev1/PFI0= right camera (default);\n                           /Dev1/PFI8= left camera"
  # "637"
  # "561"
  # "532"
  # "488"
  # "405"
  # "Red"
  # "Camera information"
  # "Confocal Status"
  # "Power calibration (2017-02-09) Confocal mode\nLaser\t     Voltage\t   mW\n405nm     1             1.22\n488nm\t    1\t            2.90    \n532nm\t    1\t            4.76    \n561nm\t    1\t            4.47       \n637nm\t   \t1             9.95"
  # "Low gain = 100mV/nA\nWith external set to div10,\nthis means DAQ 1mV = 1 pA"
  # "When updating filter set information, please edit:\nsubDAQ_SetFilterSet.vi"
  # "Global shutter mode : 4"
  # "Minimum AO for all lasers: 0.2 V"
  # "Frame        DAQ rate       Exposure\nrate (Hz)       (Hz)            time (ms)\n986.1          9681.46         1.03290\n1058          21159.48        0.9452"
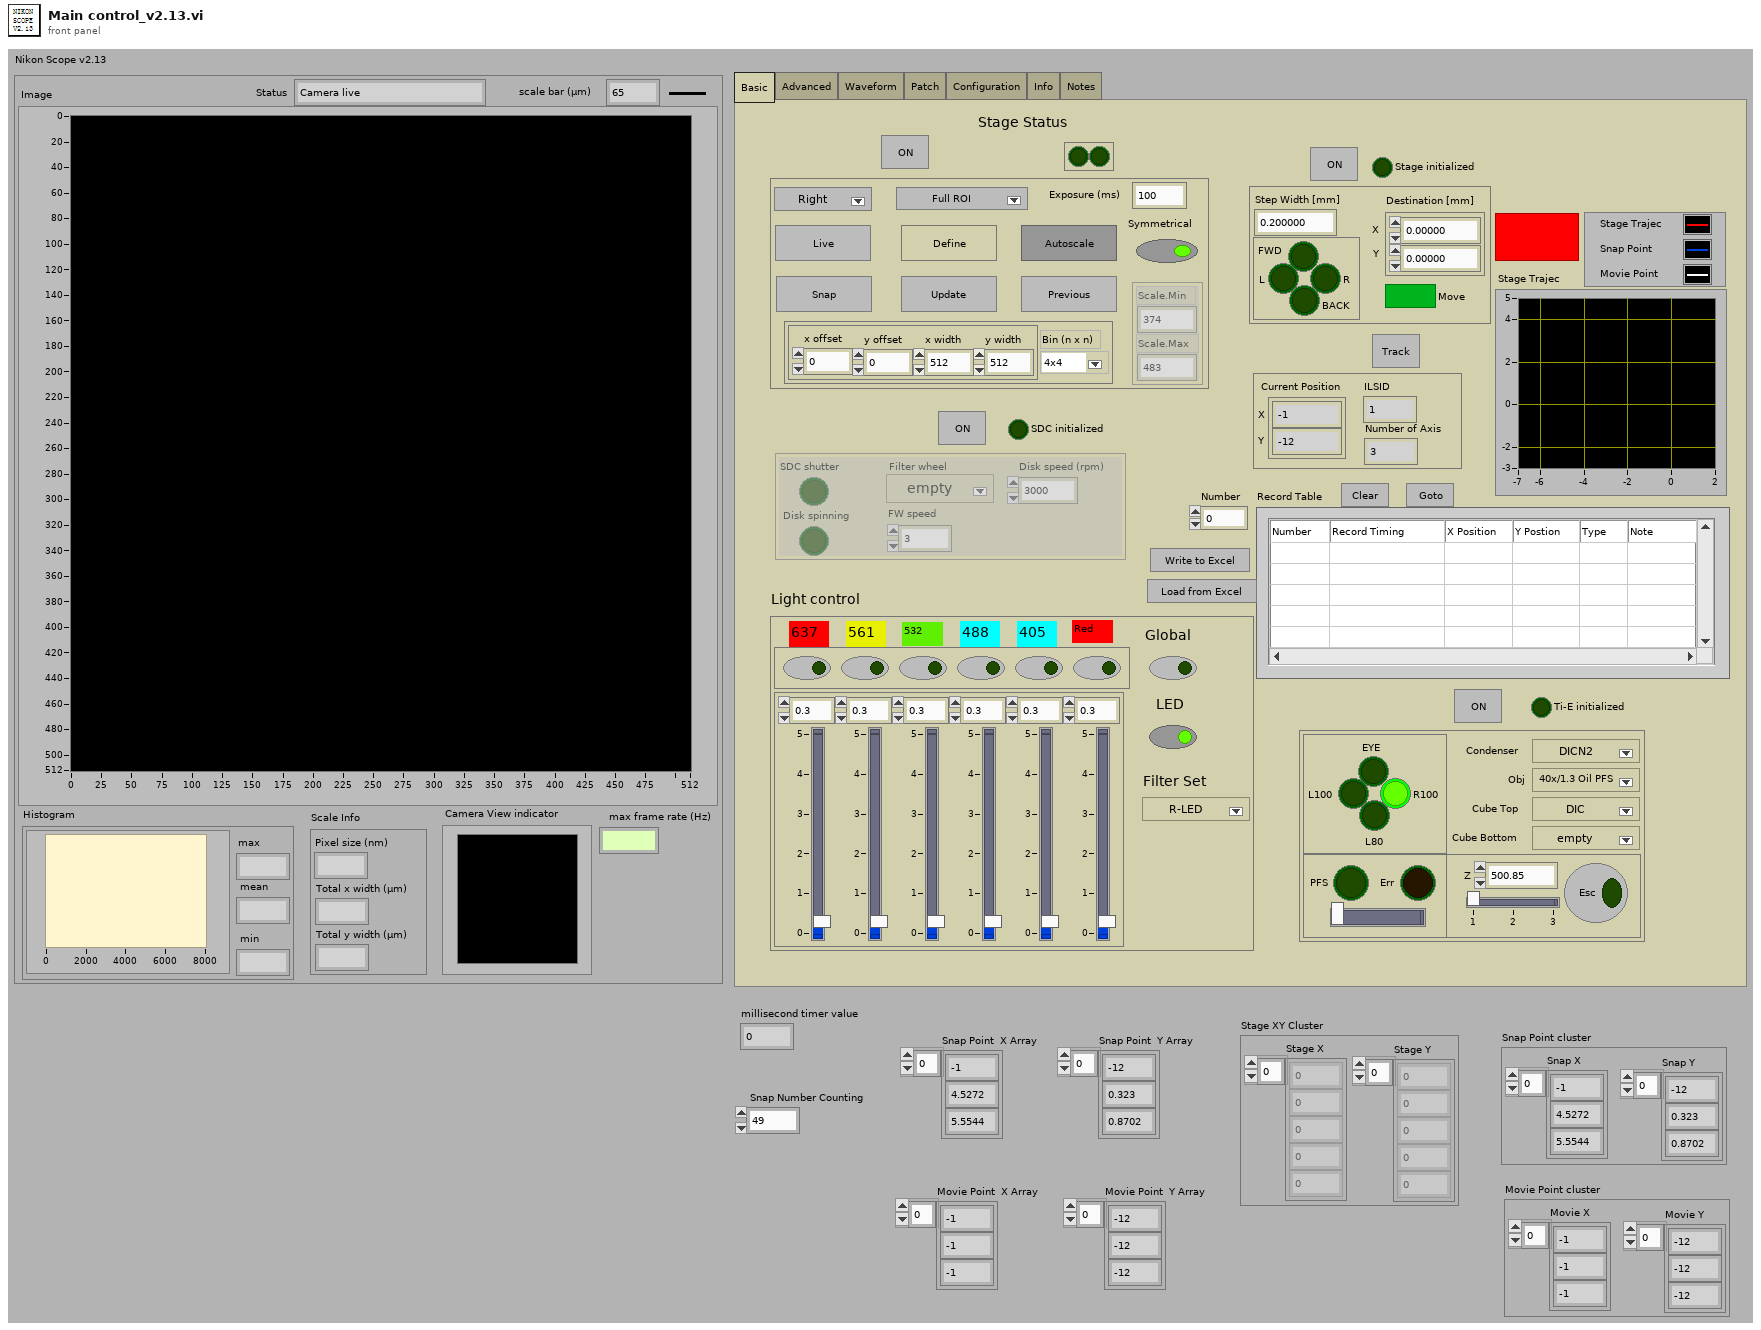
[diagram p1: front panel]
types:
  T1 = cluster{"Filter Set":i32, "Lasers DO":bool[], "Lasers AO (V)":dbl[], "LED":bool, "Global":bool}
  T2 = cluster{"Status":string, "scale bar (μm)":dbl, "Image":u16[][], "Histogram":cluster{"max value":u16, "mean":i16, "min value":u16, "Histogram":cluster{"X Values":dbl[], "Histogram: h(x)":i32[]}}, "Scale Info":cluster{"Pixel size (nm)":dbl, "Total x width (μm)":dbl, "Total y width (μm)":dbl}, "Camera View indicator":u16[][], "max frame rate (Hz)":dbl}
  T3 = cluster{"Bin":u16, "ROI":cluster{"x offset":i32, "y offset":i32, "x width":i32, "y width":i32}}
  T4 = enum32{"Basic", "Advanced", "Waveform", "Patch", "Configuration", "Info", "Notes"}
  T5 = cluster{"SDC shutter":bool, "Filter wheel":u16, "FW speed":i32, "Disk spinning":bool, "Disk speed (rpm)":dbl}
  T6 = cluster{"Console":cluster{"L":bool, "R":bool, "FWD":bool, "BACK":bool}, "Step Width [mm]":dbl, "Destination [mm]":dbl[], "Move ":bool}
  T7 = cluster{" Current Position":dbl[], "Number of Axis":i32, "ILSID":i32}
  T8 = cluster{"Chosen Camera":u32, "ROI selection":u16, "Live":bool, "ROI define":bool, "Snap":bool, "ROI update":bool, "ROI previous ":bool, "ROI":cluster{"Bin":u16, "ROI":cluster{"x offset":i32, "y offset":i32, "x width":i32, "y width":i32}}, "Exposure (ms)":dbl, "Symmetrical":bool, "Autoscale":bool, "Scale":cluster{"Scale.Min":i32, "Scale.Max":i32}}
  T9 = cluster{"Obj":u16, "Cube Bottom":u16, "Cube Top":u16, "PFS-Ctrl":cluster{"PFS IO":bool, "PSF Err":bool, "PSF Pos":u32}, "Z-Ctrl":cluster{"Z-pos":dbl, "Home":bool, "Sensitivity":u8}, "Condenser":u16, "Lightpath":enum32{"EYE", "L100", "R100", "L80"}}
  T10 = cluster{"Z end":dbl, "Step Num":i32, "Step Size":dbl, "Z0":dbl, "z-stack?":bool}
  T11 = cluster{"Take?":bool[], "Channel":i32[], "Exposure time (msec)":dbl[], "Cumulation":i32[], "Name":string[]}
  T12 = cluster{"Tiling?":bool, "YY/XX":i32[], "X0Y0":dbl[]}
  T13 = cluster{"Lasers":bool[], "Patch":bool, "Camera Output":bool}
  T14 = cluster{"Waveform folder":path, "Exposure time (ms)":dbl}
  T15 = cluster{"samples":i32, "Duration (sec)":dbl, "Downsampling factor":dbl}
  T16 = cluster{"Amplitude (mV)":dbl, "Number of repeats":i32, "DAQ rate (Hz)":dbl, "Frequency (Hz)":dbl}
  T17 = cluster{"Ra (MΩ)":dbl, "Rm (MΩ)":dbl, "Cm (pF)":dbl, "RC constant (msec)":dbl, "Steady state current (pA)":dbl}
  T18 = cluster{"DAQ ports":cluster{"Lasers DO lines":tag[], "Lasers AO lines":tag[], "Patch AO line":tag, "Patch AI lines 1":cluster{"Patch scaled output":tag, "Patch 10 V_m ":tag}, "Camera timing DI":tag, "Dev1 timing DO ":tag, "Dev1 trigger source":tag, "Dev2 trigger source":tag, "LED line":tag, "Global Shutter line":tag, "Patch AI lines 2":cluster{"Cell capacitance":tag, "Mode":tag, "Frequency":tag, "Gain":tag}}, "Camera Setting":cluster{"Camera Output triger mode setiting":cluster{"Mode":u32, "Polarity":u32, "Period":dbl, "Delay":dbl}, "Camera timing port for trigering":enum16{"1", "2", "3"}}, "Stage setting":cluster{"Baudrate":i32, "COM Port":string, "Xmax":dbl, "Xmin":dbl, "Ymax":dbl, "Ymin":dbl}, "Confocal VISA Setting":refnum<visa-resource-name>}
  T19 = cluster{"Camera Details Array":cluster{"Model":string, "Camera ID":string, "Firmware":string}[], "Handle":u32, "Camera in use ":cluster{"Model":string, "Camera ID":string, "Bits":i32}}
  T20 = cluster{"Actual Disk speed (rpm)":string, "Actual FW speed (rpm)":i32}
  T21 = cluster{"TI":refnum<k7>, "Nosepiece":refnum<k7>, "LightPathDrive":refnum<k7>, "ZDrive":refnum<k7>, "PFS":refnum<k7>, "CondenserCassette":refnum<k7>, "FilterBlockCassette1":refnum<k7>, "FilterBlockCassette2":refnum<k7>}
  T22 = cluster{"width":u32, "height":u32, "datatype":u32}
  T23 = enum8{"Enabled", "Disabled", "Disabled and Grayed Out"}
  T24 = cluster{"SDC shutter":bool, "FWPosition":i32, "FW speed":i32, "Disk spinning?":bool, "Disk speed (rpm)":dbl}
  T25 = cluster{"Lasers DO lines":tag[], "Lasers AO lines":tag[], "Patch AO line":tag, "Patch AI lines 1":cluster{"Patch scaled output":tag, "Patch 10 V_m ":tag}, "Camera timing DI":tag, "Dev1 timing DO ":tag, "Dev1 trigger source":tag, "Dev2 trigger source":tag, "LED line":tag, "Global Shutter line":tag, "Patch AI lines 2":cluster{"Cell capacitance":tag, "Mode":tag, "Frequency":tag, "Gain":tag}}
  T26 = cluster{"Baudrate":i32, "COM Port":string, "Xmax":dbl, "Xmin":dbl, "Ymax":dbl, "Ymin":dbl}
  T27 = cluster{"LEFT":bool, "RIGHT":bool, "FWD":bool, "BACK":bool}
  T28 = cluster{"Total x width (μm)":refnum<vi>, "Total y width (μm)":refnum<vi>, "Pixel size (nm)":refnum<vi>, "scale bar (μm)":refnum<vi>}
  T29 = cluster{"Ra (Mohm)":dbl, "Rm (Mohm)":dbl, "Cm (pF)":dbl, "RC constant (msec)":dbl, "Steady state current (pA)":dbl}
  T30 = cluster{"max value":u16, "mean":i16, "min value":u16, "Histogram":cluster{"X Values":dbl[], "Histogram: h(x)":i32[]}}
  T31 = cluster{"Camera Output triger mode setiting":cluster{"Mode":u32, "Polarity":u32, "Period":dbl, "Delay":dbl}, "Camera timing port for trigering":enum16{"1", "2", "3"}}
  T32 = cluster{"Model":string, "Camera ID":string, "Bits":i32}
  T33 = cluster{"Lasers DO lines":tag[], "Lasers AO lines":tag[], "Patch AO line":tag, "Patch AI lines":tag[], "Dev1 timing DO":tag, "Camera timing DI":tag, "Dev1 trigger source":tag, "Dev2 trigger source":tag}
  T34 = cluster{"Sampling rate (Hz)":dbl, "dt (sec)":dbl, "total time (sec)":dbl, "# samples":i32, "Exposure time (ms)":dbl, "# frames":i32}
  T35 = cluster{"TI-Ctrl":refnum<vi>, "TiE Ref":cluster{"TI":refnum<k7>, "Nosepiece":refnum<k7>, "LightPathDrive":refnum<k7>, "ZDrive":refnum<k7>, "PFS":refnum<k7>, "CondenserCassette":refnum<k7>, "FilterBlockCassette1":refnum<k7>, "FilterBlockCassette2":refnum<k7>}}
  T36 = cluster{"Filter Set":i32, "Light control":refnum<vi>, "Confocal scanner":refnum<vi>, "Value":cluster{"Lasers DO lines":tag[], "Lasers AO lines":tag[], "Patch AO line":tag, "Patch AI lines 1":cluster{"Patch scaled output":tag, "Patch 10 V_m ":tag}, "Camera timing DI":tag, "Dev1 timing DO ":tag, "Dev1 trigger source":tag, "Dev2 trigger source":tag, "LED line":tag, "Global Shutter line":tag, "Patch AI lines 2":cluster{"Cell capacitance":tag, "Mode":tag, "Frequency":tag, "Gain":tag}}, "Value":refnum<visa-resource-name>}
  T37 = cluster{"XY tiling":cluster{"Tiling?":bool, "YY/XX":i32[], "X0Y0":dbl[]}, "Stage Status":refnum<vi>}
  T38 = cluster{i32, "appended path":path, "Z-Stack":cluster{"Z end":dbl, "Step Num":i32, "Step Size":dbl, "Z0":dbl, "z-stack?":bool}, "Arch_Dragon cumulation":i32, "Image Info":refnum<vi>, "Camera Ctrl":cluster{"Chosen Camera":u32, "ROI selection":u16, "Live":bool, "ROI define":bool, "Snap":bool, "ROI update":bool, "ROI previous ":bool, "ROI":cluster{"Bin":u16, "ROI":cluster{"x offset":i32, "y offset":i32, "x width":i32, "y width":i32}}, "Exposure (ms)":dbl, "Symmetrical":bool, "Autoscale":bool, "Scale":cluster{"Scale.Min":i32, "Scale.Max":i32}}}
  T39 = cluster{"NewVal":i32, "Light control":refnum<vi>, "Confocal scanner":refnum<vi>, "Value":cluster{"Lasers DO lines":tag[], "Lasers AO lines":tag[], "Patch AO line":tag, "Patch AI lines 1":cluster{"Patch scaled output":tag, "Patch 10 V_m ":tag}, "Camera timing DI":tag, "Dev1 timing DO ":tag, "Dev1 trigger source":tag, "Dev2 trigger source":tag, "LED line":tag, "Global Shutter line":tag, "Patch AI lines 2":cluster{"Cell capacitance":tag, "Mode":tag, "Frequency":tag, "Gain":tag}}, "Value":refnum<visa-resource-name>}
  T40 = cluster{"Obj":u16, "Cube 1":u16, "Cube 2":u16, "PFS-Ctrl":cluster{"PFS IO":bool, "PSF Err":bool, "PSF Pos":u32}, "Z-Ctrl":cluster{"Z-pos":dbl, "Home":bool, "Sensitivity":u8}, "Condenser":u16, "Lightpath":enum32{"EYE", "L100", "R100", "L80"}}
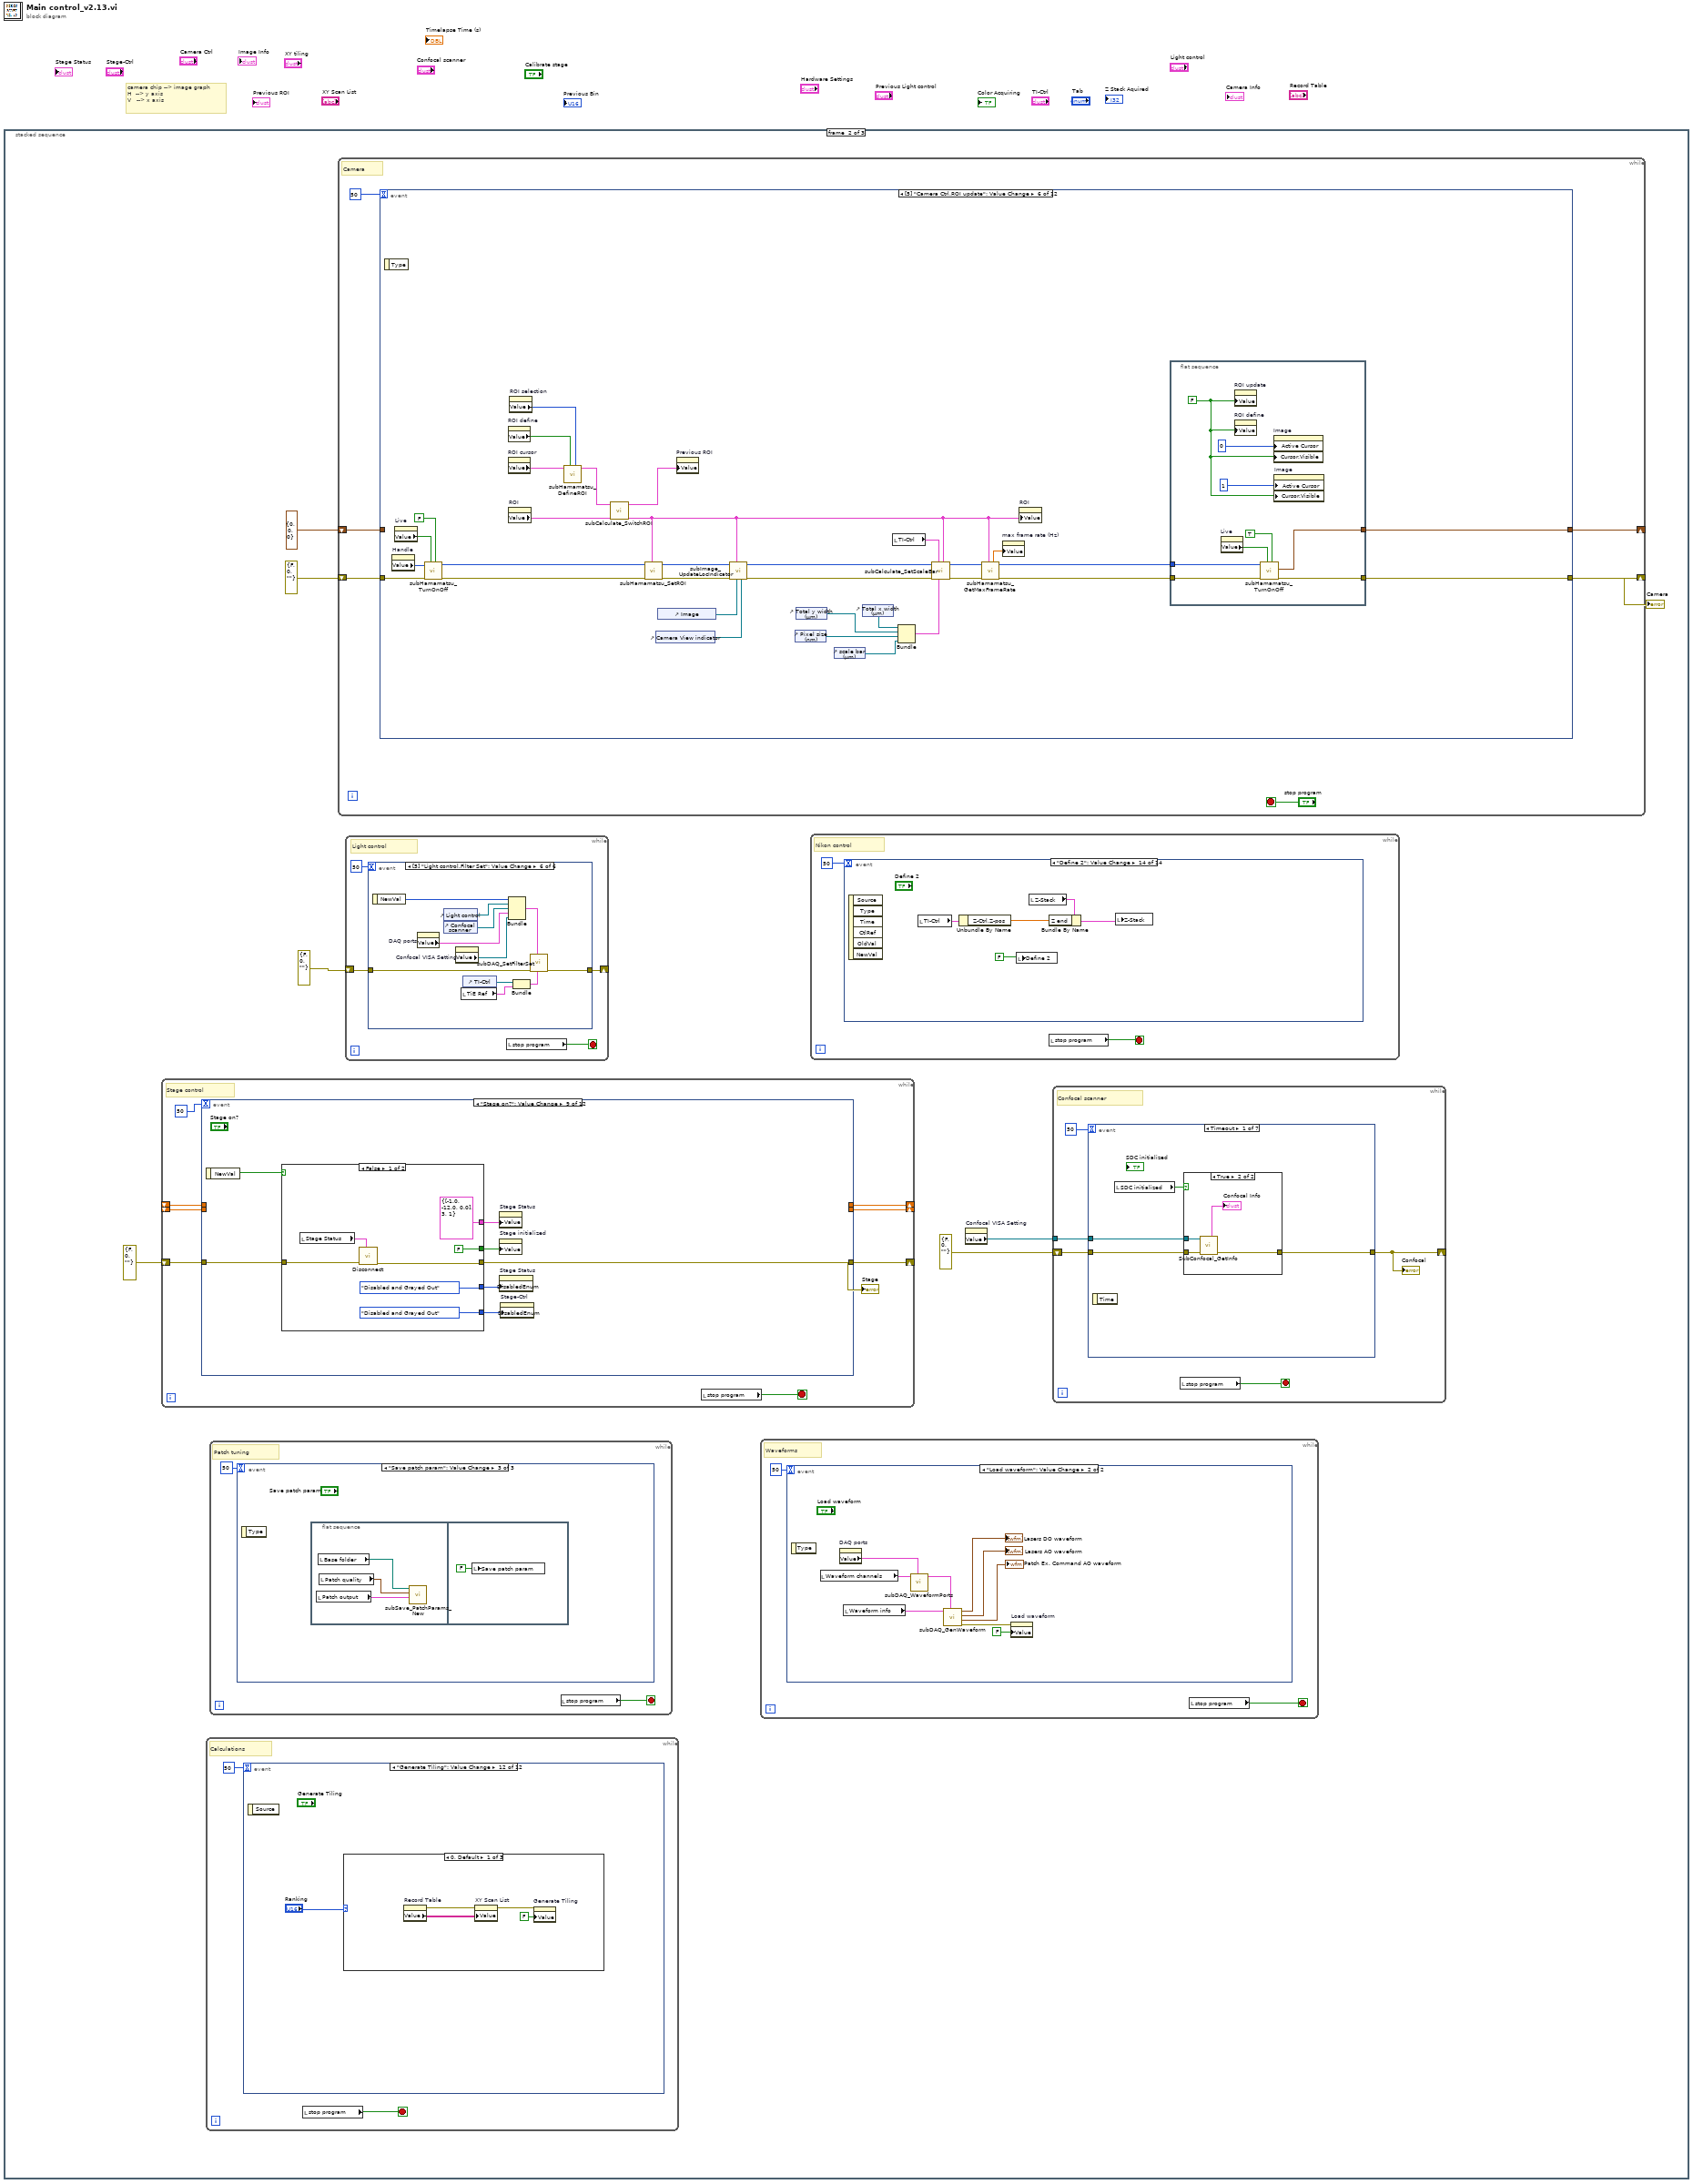
[diagram p0: block diagram]
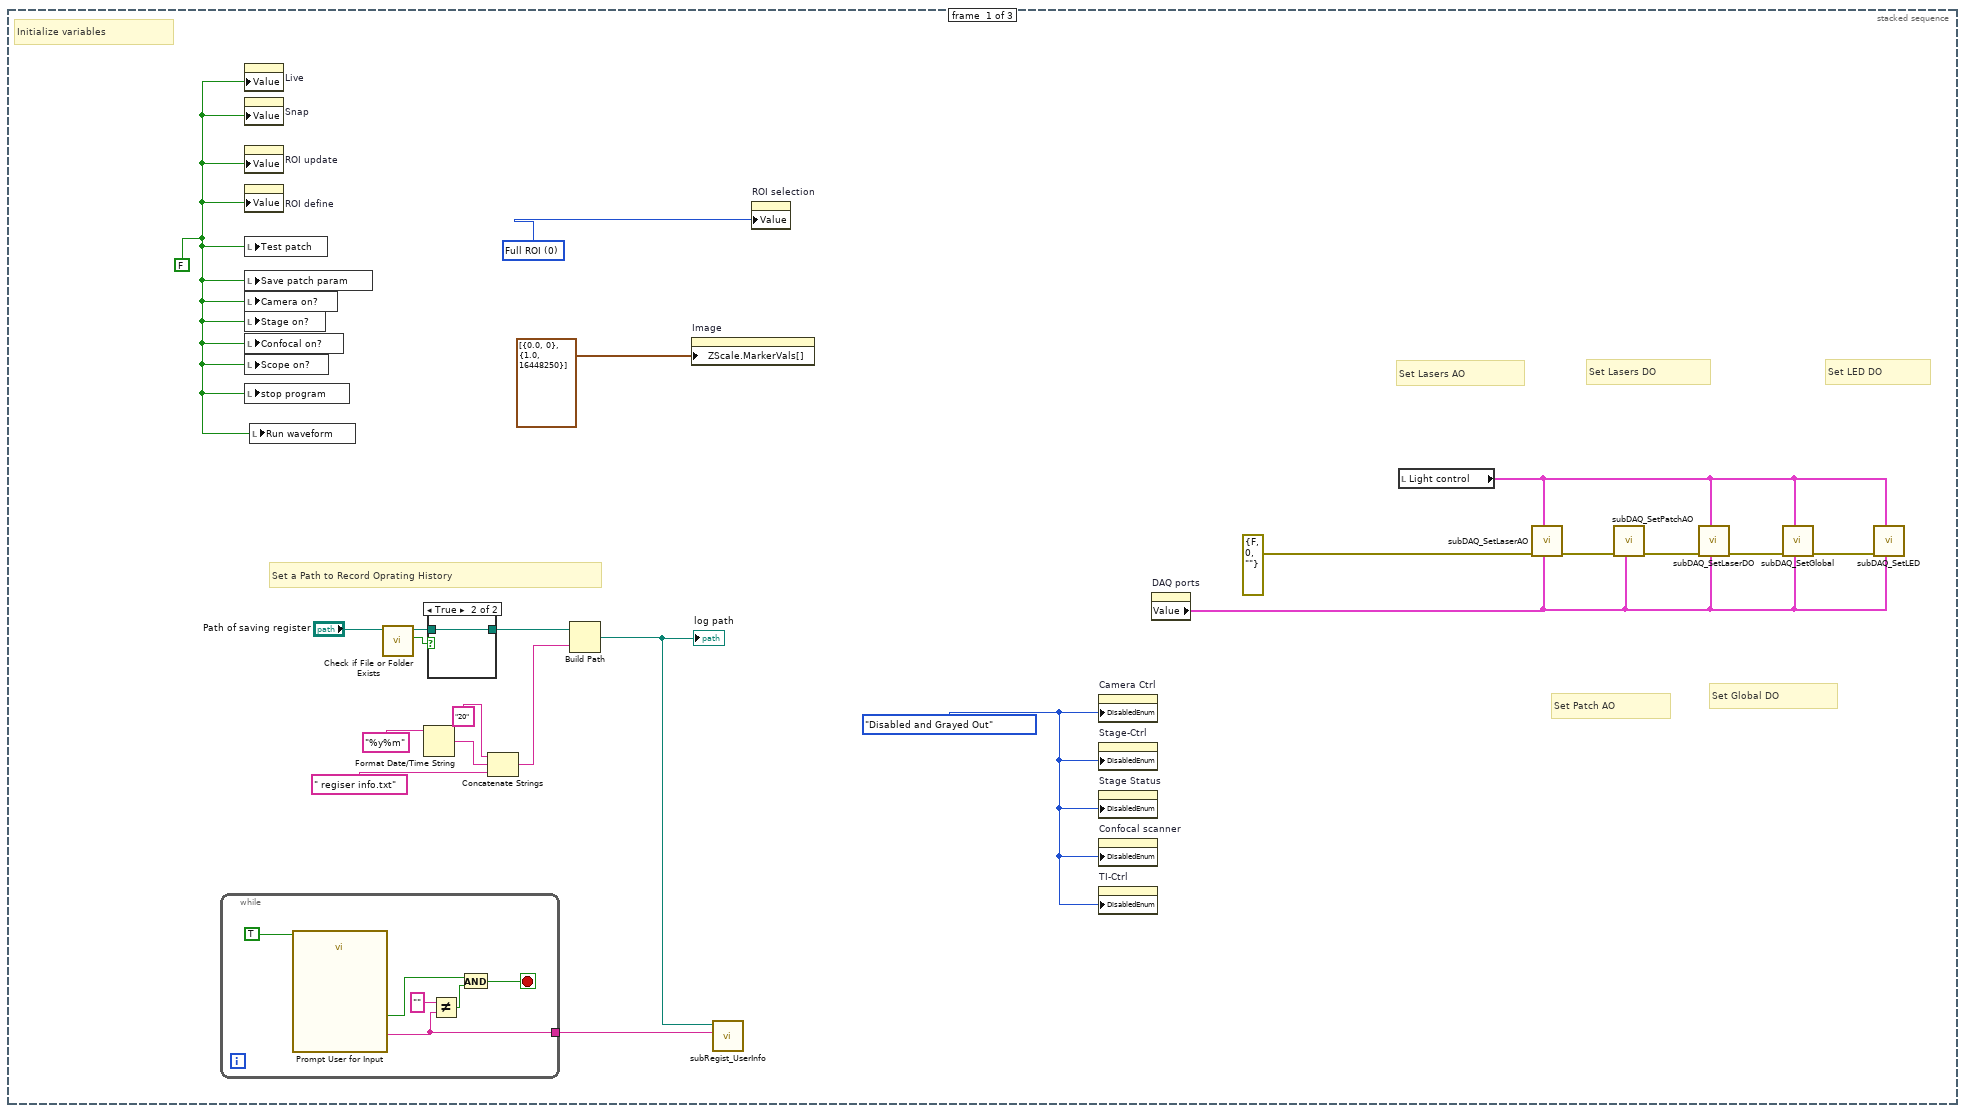
[diagram p2: hidden frame]
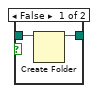
[diagram p3: hidden frame]
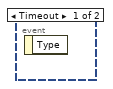
[diagram p4: hidden frame]
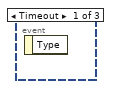
[diagram p5: hidden frame]
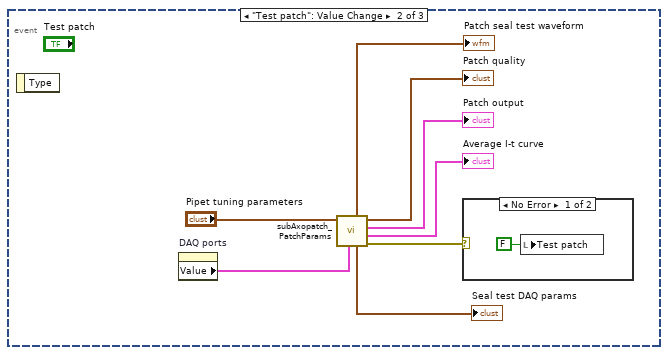
[diagram p6: hidden frame]
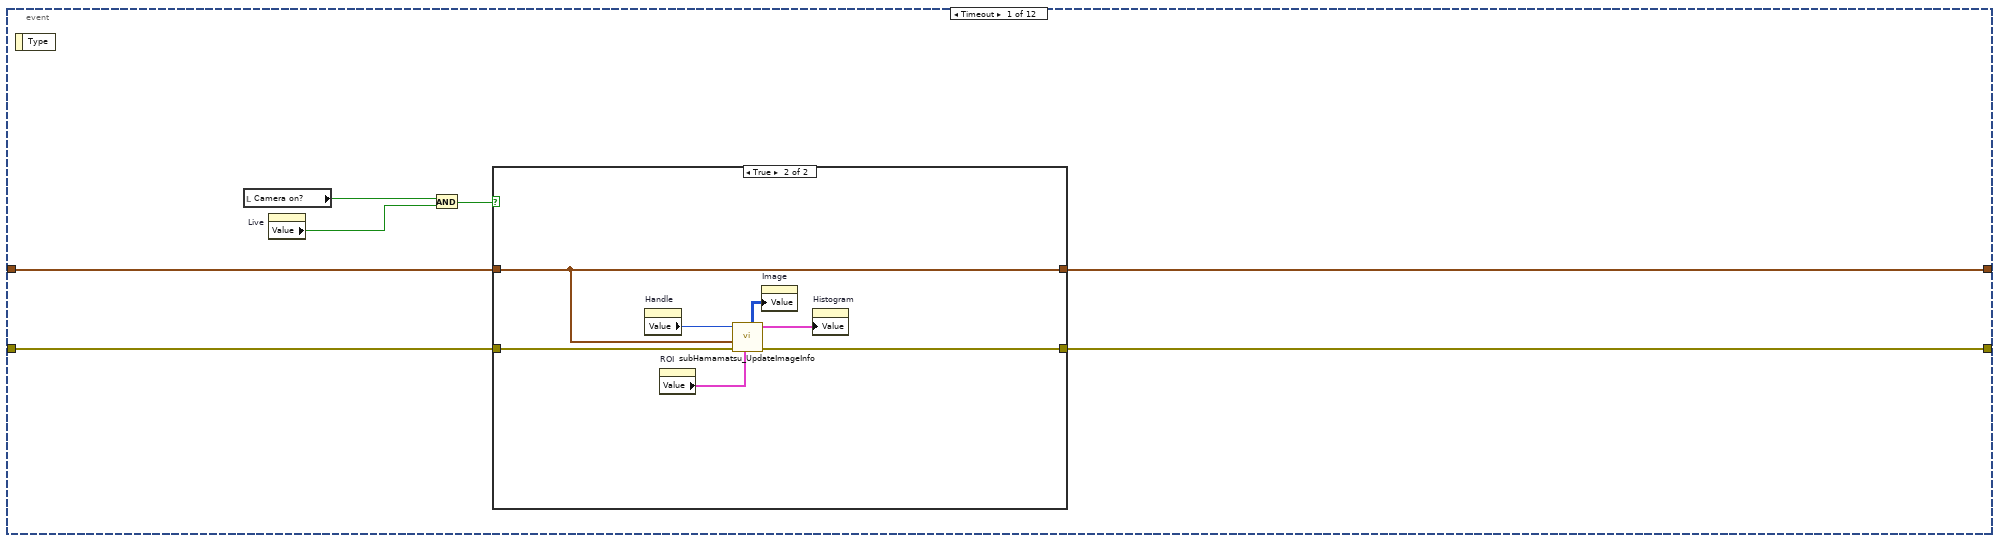
[diagram p8: hidden frame]
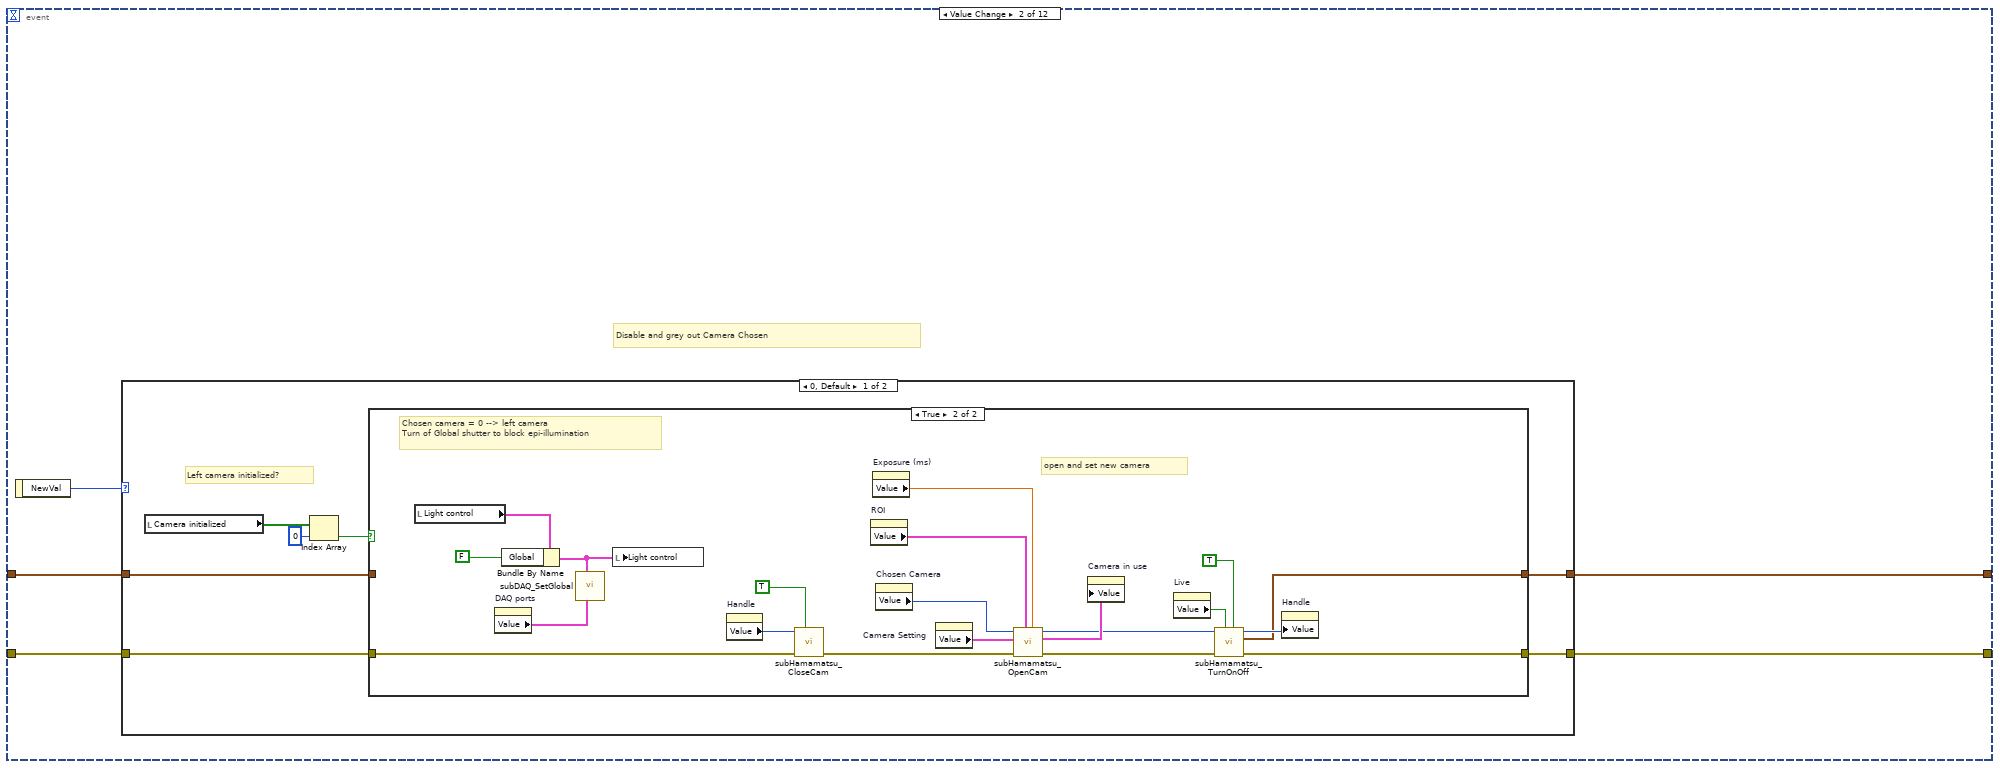
[diagram p10: hidden frame]
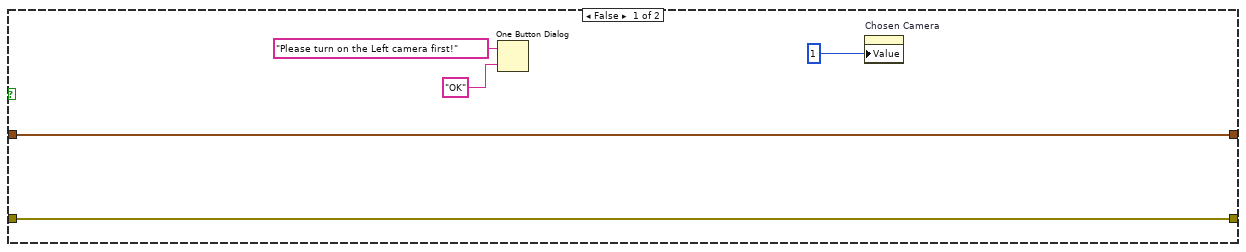
[diagram p11: hidden frame]
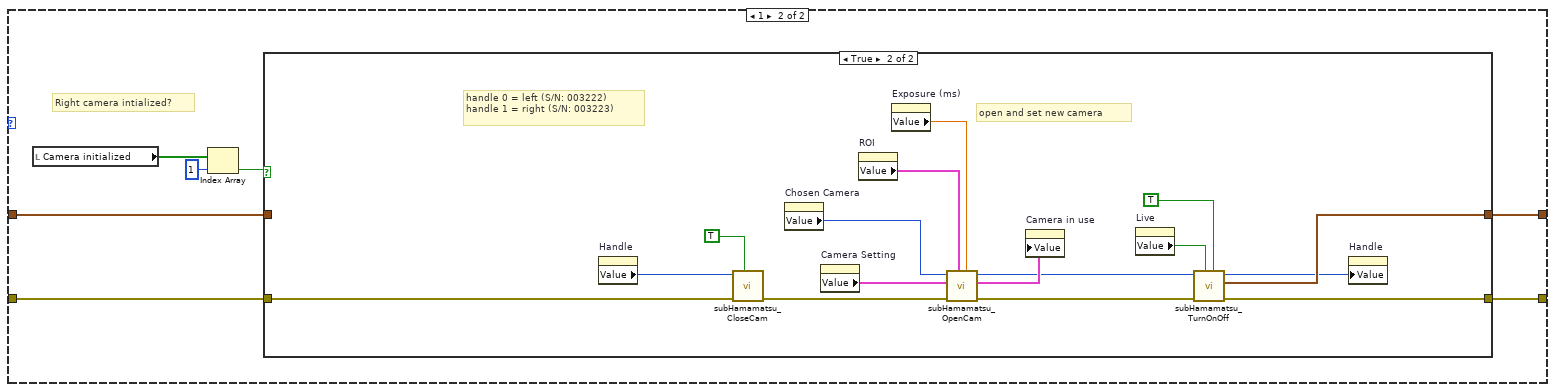
[diagram p12: hidden frame]
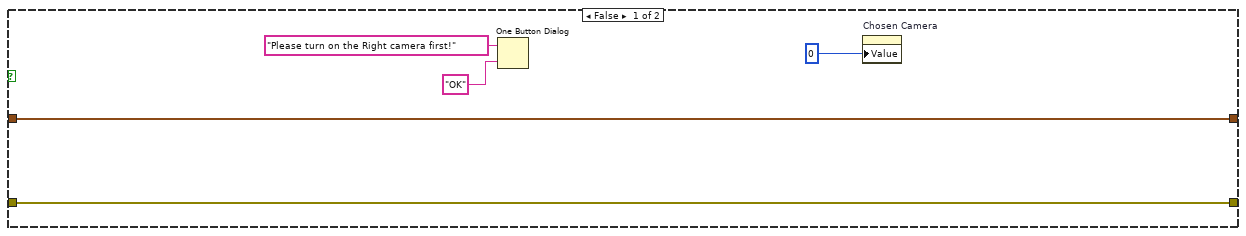
[diagram p13: hidden frame]
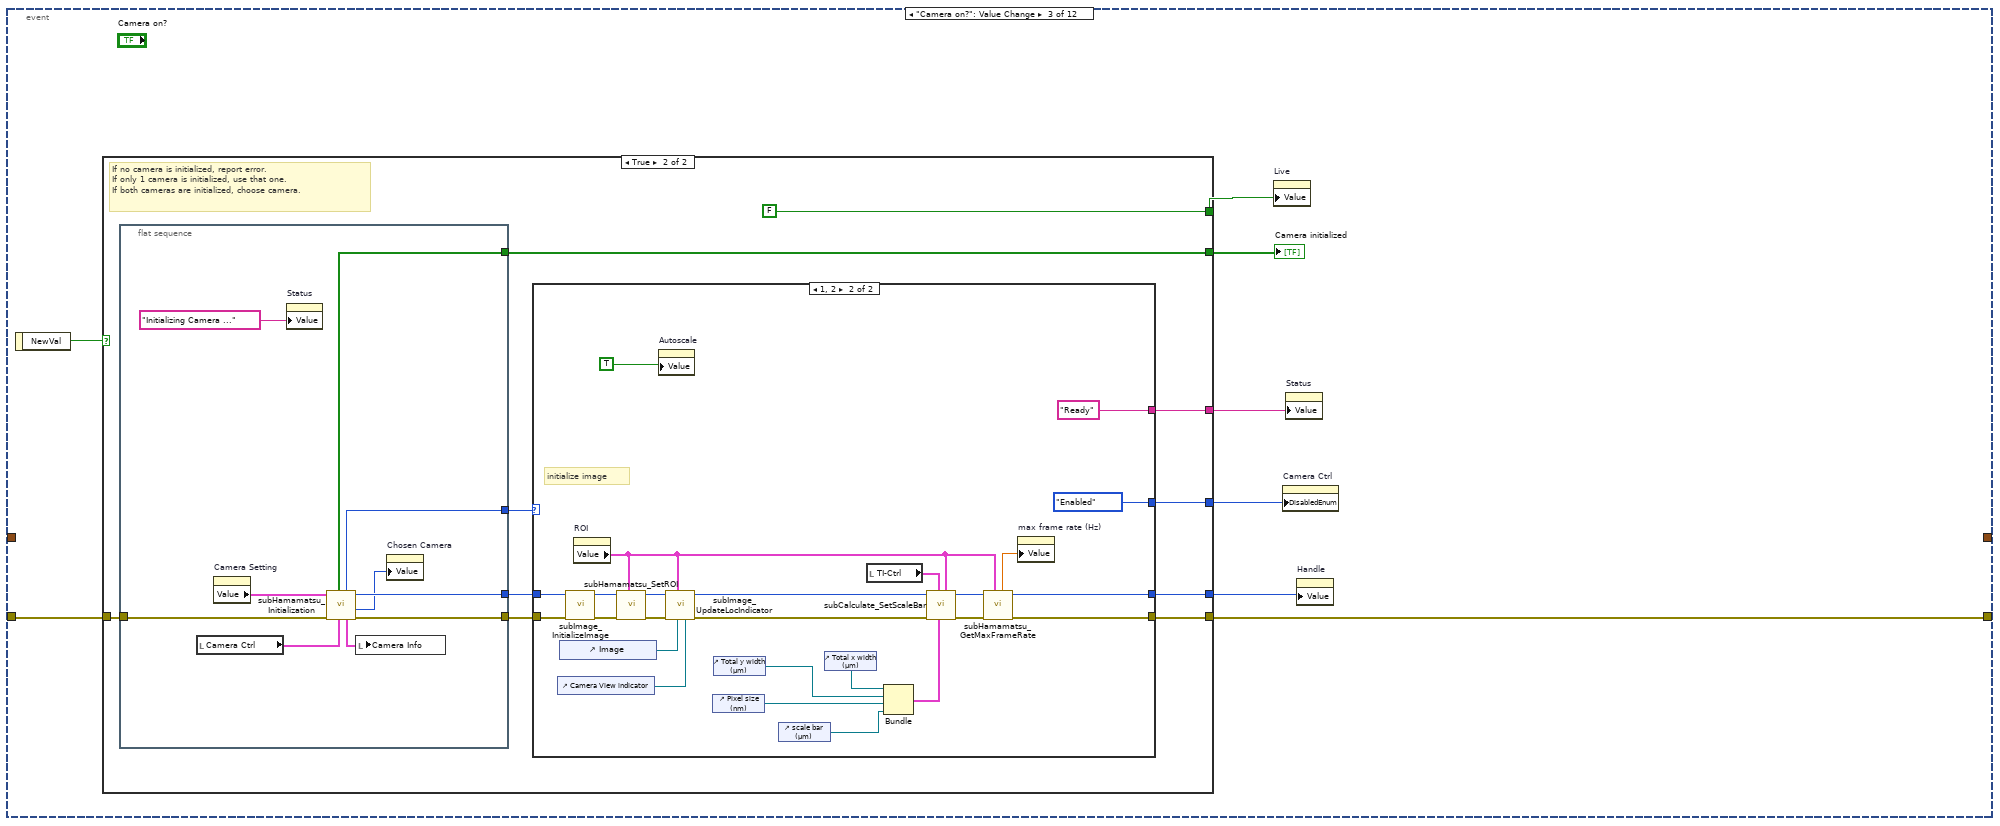
[diagram p14: hidden frame]
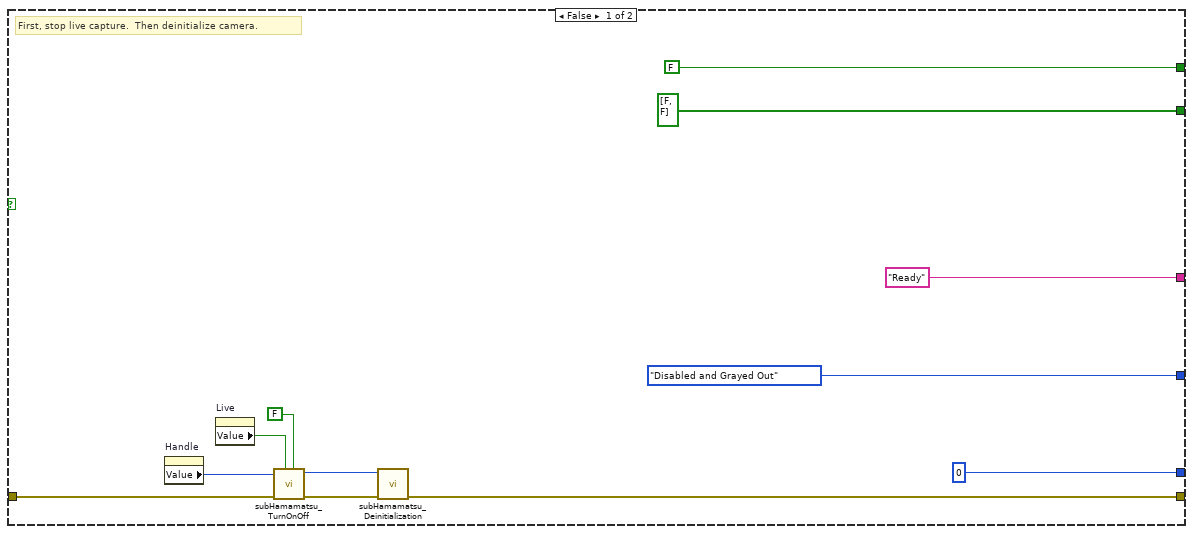
[diagram p15: hidden frame]
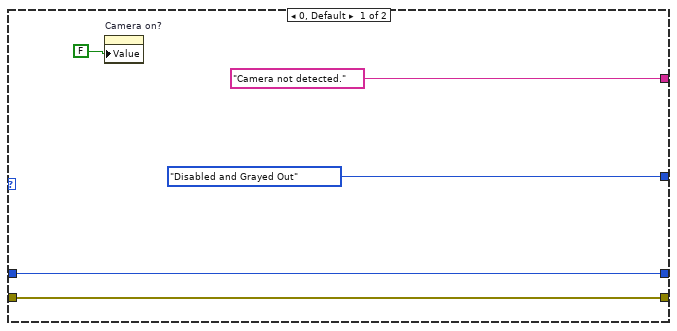
[diagram p16: hidden frame]
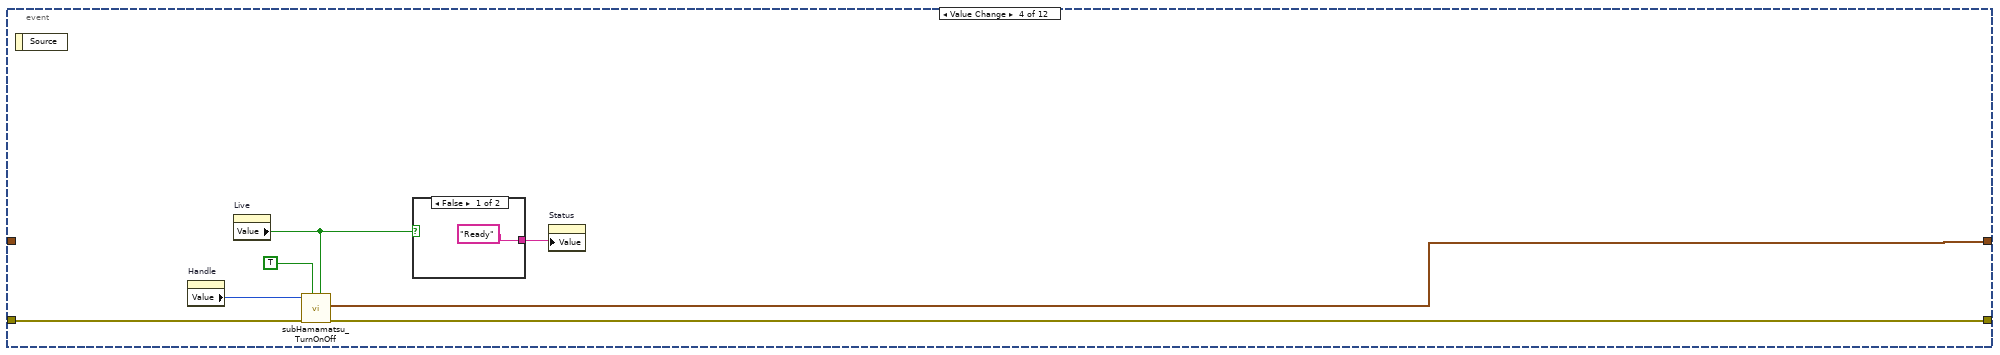
[diagram p17: hidden frame]
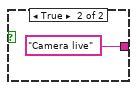
[diagram p18: hidden frame]
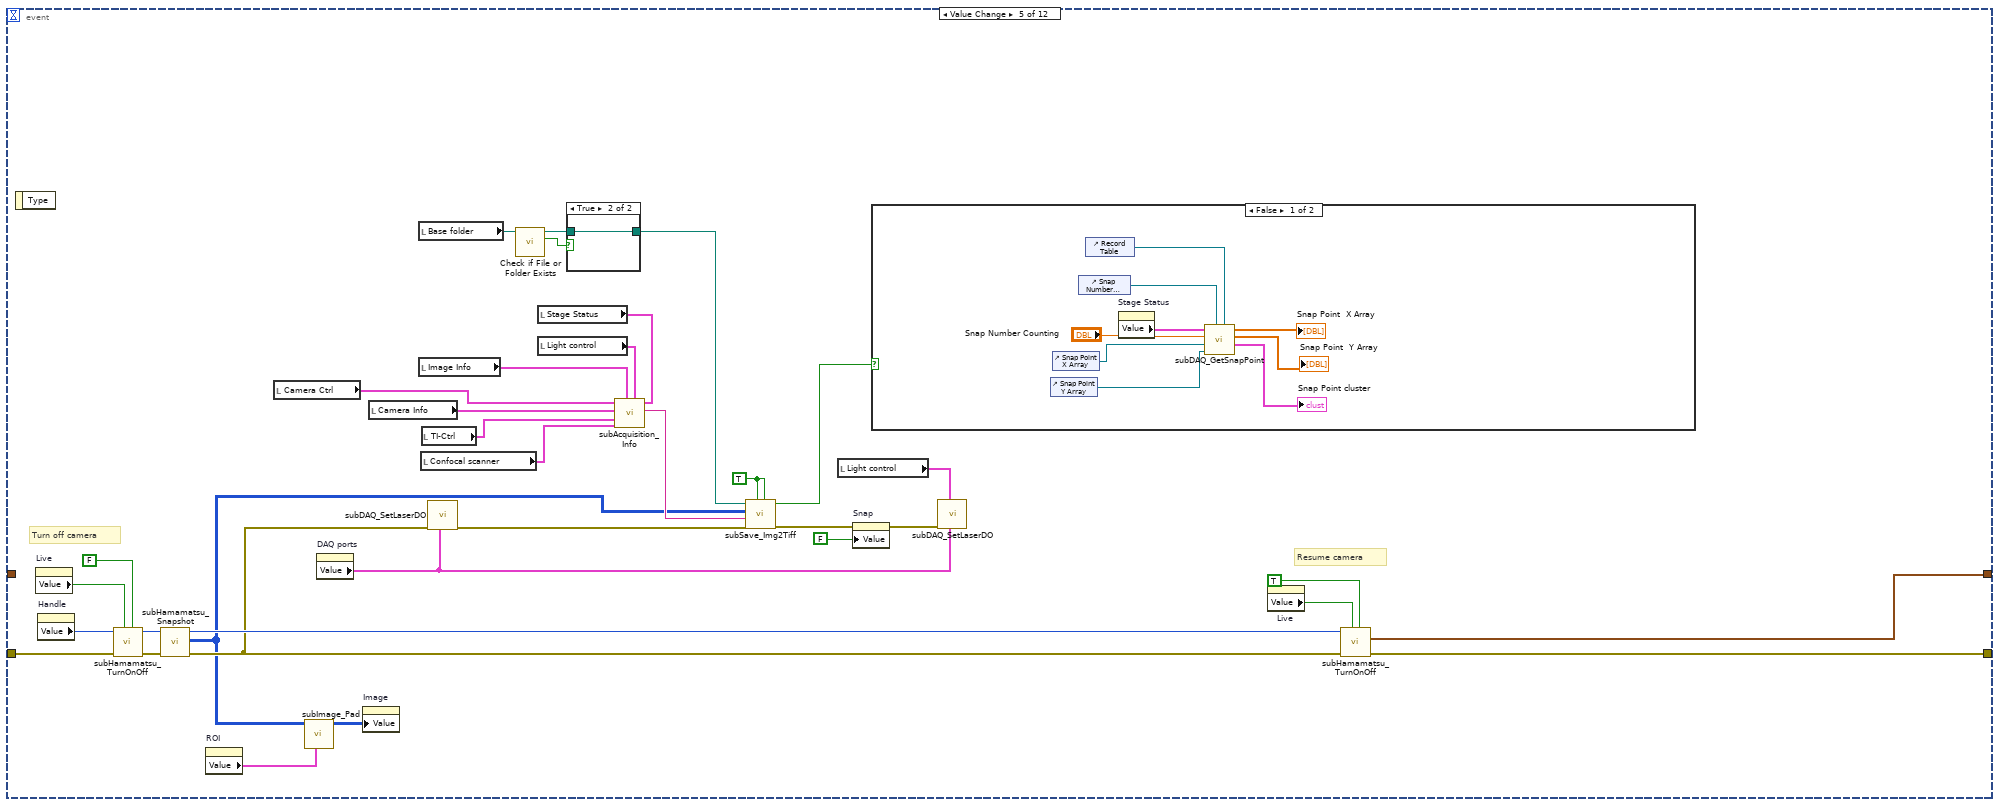
[diagram p19: hidden frame]
diagram:
  # "camera chip --> image graph\nH  --> y axis\nV   --> x axis"
  n1 = stacked-sequence {
    frame #0 {
      w5 = T23."Disabled and Grayed Out" ("Disabled")
      w3 = u16 0 items=["Full ROI", "Central quad", "Custom ROI"] ("ROI selection")
      w4 = FALSE ("stop program")
      # "Set LED DO"
      # "Set Global DO"
      # "Set Patch AO"
      # "Set Lasers DO"
      # "Set Lasers AO"
      # "Set a Path to Record Oprating History"
      # "Initialize variables"
      n2 = while {
        tunnel: [w23] -> w20
        stop <- w24 stop-if-true
        n3 = call "Prompt User for Input"("Enable"=TRUE) -> ("使用前请登记，使用后请按流程关闭程序，不要点保存，谢谢！"=w23:string, "OK"=w28:bool)  [unwired: 16 in, 1 out]
        n4 = Not Equal?(x="", y=w23) -> (x != y?=w27:bool)
        n5 = And(x=w28, y=w27) -> (x .and. y?=w24:bool)
      }
      n6 = property on="Live" class="Bool (strict)"("Value"=w4) -> ()  [unwired: 2 in, 2 out]
      n7 = property on="Snap" class="Bool (strict)"("Value"=w4) -> ()  [unwired: 2 in, 2 out]
      n8 = property on="ROI update" class="Bool (strict)"("Value"=w4) -> ()  [unwired: 2 in, 2 out]
      n9 = property on="ROI define" class="Bool (strict)"("Value"=w4) -> ()  [unwired: 2 in, 2 out]
      n10 = local write "Test patch"(w4) -> ()
      n11 = local write "Save patch param"(w4) -> ()
      n12 = local write "Camera on?"(w4) -> ()
      n13 = local write "Stage on?"(w4) -> ()
      n14 = local write "Confocal on?"(w4) -> ()
      n15 = local write "Scope on?"(w4) -> ()
      n16 = local write "stop program"(w4) -> ()
      n17 = local write "Run waveform"(w4) -> ()
      n18 = call <vilib>:"Check if File or Folder Exists.vi"("path"="Path of saving register") -> ("file or folder exists?"=w21:bool, "dup path"=w22:path)  [unwired: 8 in, 1 out]
      n19 = Format Date/Time String(time format string (%c)="%y%m") -> (date/time string=w18:string)  [unwired: 2 in]
      n20 = case shown="True" w21 {
        tunnel: w22 -> [w30 w31]
        tunnel: [w29 w31] -> w14
        frame False {
          n21 = Create Folder(path (use dialog)=w30) -> (created path=w29:path)  [unwired: 2 in, 2 out]
        }
        frame True {
        }
      }
      n22 = Concatenate Strings("20" ("string"), w18, " regiser info.txt" ("string")) -> (w17:string)
      n23 = Build Path(base path=w14, name or relative path=w17) -> (appended path=w6:path)
      "log path" <- w6
      n24 = property on="Image" class="IntGraph (strict)"("ZScale.MarkerVals[]"=cluster{dbl, u32}[] [{0.0, 0}, {1.0, 16448250}] ("Z Scale.Marker Values[]")) -> ()  [unwired: 2 in, 2 out]
      n25 = call "subRegist_UserInfo.vi"("user name"=w20, "log path"=w6) -> ()  [unwired: 10 in]
      n26 = property on="ROI selection" class="Ring (strict)"("Value"=w3) -> ()  [unwired: 2 in, 2 out]
      n27 = property on="Camera Ctrl" class="Clust (strict)"("DisabledEnum"=w5) -> ()  [unwired: 2 in, 2 out]
      n28 = property on="Stage-Ctrl" class="Clust (strict)"("DisabledEnum"=w5) -> ()  [unwired: 2 in, 2 out]
      n29 = property on="Stage Status" class="Clust (strict)"("DisabledEnum"=w5) -> ()  [unwired: 2 in, 2 out]
      n30 = property on="Confocal scanner" class="Clust (strict)"("DisabledEnum"=w5) -> ()  [unwired: 2 in, 2 out]
      n31 = property on="TI-Ctrl" class="Clust (strict)"("DisabledEnum"=w5) -> ()  [unwired: 2 in, 2 out]
      n32 = property on="DAQ ports" class="Clust (strict)"() -> ("Value"=w1:T25)  [unwired: 2 in, 2 out]
      n33 = local read "Light control"() -> (w7:T1)
      n34 = call "subDAQ_SetLaserAO.vi"("DAQ ports"=w1, "Light control (All off)"=w7, "Error in (no error)"=errorcluster {"status"=FALSE, "code"=0, "source"=""} ("error out")) -> ("Error out"=w11:errorcluster)  [unwired: 8 in]
      n35 = call "subDAQ_SetPatchAO.vi"("DAQ ports"=w1, "Error in (no error)"=w11) -> ("Error out"=w10:errorcluster)  [unwired: 9 in]
      n36 = call "subDAQ_SetLaserDO.vi"("DAQ ports"=w1, "Light control (All off)"=w7, "Error in (no error)"=w10) -> ("Error out"=w9:errorcluster)  [unwired: 8 in]
      n37 = call "subDAQ_SetGlobal.vi"("DAQ ports"=w1, "Light control (All off)"=w7, "Error in (no error)"=w9) -> ("Error out"=w8:errorcluster)  [unwired: 8 in]
      n38 = call "subDAQ_SetLED.vi"("DAQ ports"=w1, "Light control (All Off)"=w7, "Error in (no error)"=w8) -> ()  [unwired: 8 in, 1 out]
    }
    frame #1 {
      n39 = while {
        shift-right: [w787] -> _
        shift-left: errorcluster {"status"=FALSE, "code"=0, "source"=""} ("Error out") -> [w789]
        shift-right: [w786] -> _
        shift-left: _ -> [w785]
        shift-right: [w784] -> _
        shift-left: _ -> [w783]
        stop <- w788 stop-if-true
        # "Stage control"
        n40 = event shown="[8] \"Stage on?\": Value Change" {
          selector: _ -> [_ _ _ _ _ _ _ _ _ _ _ _]
          dyn-events: _ -> [_ _ _ _ _ _ _ _ _ _ _ _]
          timeout: 50 -> [_ _ _ _ _ _ _ _ _ _ _ _]
          tunnel: w789 -> [w797 _ w825 w836 w842 w851 w861 w869 w876 w901 w921 w928]
          tunnel: [w796 _ w823 w834 w847 w848 w857 w865 w878 w897 w917 w926] -> w787
          tunnel: [w794 _ w818 w838 w844 w853 w862 w870 _ w893 w912 w922] -> w786
          tunnel: w785 -> [w793 _ w818 w838 w844 w853 w862 w870 _ w893 w912 w922]
          tunnel: [w792 _ w819 w839 w845 w854 w863 w871 _ w894 w913 w923] -> w784
          tunnel: w783 -> [w791 _ w819 w839 w845 w854 w863 w871 _ w894 w913 w923]
          event Timeout {
            n41 = event-data() -> ()  [unwired: 1 in, 1 out]
            n42 = local read "Stage initialized"() -> (w795:bool)
            n43 = case shown="True" w795 {
              tunnel: w797 -> [w800 w813]
              tunnel: [w800 w814] -> w796
              tunnel: [w798 w807] -> w794
              tunnel: w793 -> [w798 w810]
              tunnel: [w799 w808] -> w792
              tunnel: w791 -> [w799 w809]
              frame False {
              }
              frame True {
                n44 = local read "Stage Status"() -> (w811:T7)
                n45 = call "subStage_GetPosition.vi"("Stage Info In"=w811, "Error In"=w813) -> ("Error out"=w814:errorcluster, "Stage Info Out"=w812:T7)  [unwired: 8 in]
                n46 = local write "Stage Status"(w812) -> ()
                n47 = call "subStage_TrackTrajectory.vi"("Track on?"="Track on?", "Stage Current Status"=w812, "Stage Previous Status"=w811, "Stage X Array In"=w810, "Stage Y Array In"=w809) -> ("Stage X Array Out"=w807:dbl[], "Stage Y Array Out"=w808:dbl[], "Stage XY Cluster"=→"Stage XY Cluster":cluster{dbl[], dbl[]})  [unwired: 4 in]
                n48 = local read "Snap Point cluster"() -> (w803:cluster{"Snap Y":dbl[], "Snap X":dbl[]})
                n49 = local read "Stage XY Cluster"() -> (w804:cluster{"Stage Y ":dbl[], "Stage X":dbl[]})
                n50 = local read "Movie Point cluster"() -> (w802:cluster{"Movie Y":dbl[], "Movie X":dbl[]})
                n51 = Build Array(w804, w803, w802) -> (→"Stage Trajec":cluster{"Movie Y":dbl[], "Movie X":dbl[]}[])
              }
            }
          }
          event "Track on?": Value Change {
            w816 = dbl[] [] ("Movie Point  X Array")
            w817 = cluster{dbl[], dbl[]} {[], []}
            n52 = event-data() -> ()  [unwired: 1 in, 1 out]
            n53 = property on="Snap Point cluster" class="Clust (strict)"("Value"=w817) -> ()  [unwired: 2 in, 2 out]
            n54 = property on="Stage XY Cluster" class="Clust (strict)"("Value"=w817) -> ()  [unwired: 2 in, 2 out]
            n55 = property on="Movie Point cluster" class="Clust (strict)"("Value"=w817) -> ()  [unwired: 2 in, 2 out]
            n56 = property on="Movie Point  X Array" class="Arr (strict)"("Value"=w816) -> ()  [unwired: 2 in, 2 out]
            n57 = property on="Movie Point  Y Array" class="Arr (strict)"("Value"=w816) -> ()  [unwired: 2 in, 2 out]
            n58 = property on="Snap Number Counting" class="DigNum (strict)"("Value"=0.0 ("Snap Number Counting")) -> ()  [unwired: 2 in, 2 out]
            n59 = property on="Snap Point  X Array" class="Arr (strict)"("Value"=w816) -> ()  [unwired: 2 in, 2 out]
            n60 = property on="Snap Point  Y Array" class="Arr (strict)"("Value"=w816) -> ()  [unwired: 2 in, 2 out]
          }
          event "Clear Table": Value Change {
            n61 = event-data() -> ()  [unwired: 1 in, 1 out]
            n62 = Two Button Dialog(message="Are you sure to clear this table?\nPlease write the tabel to Excel first.") -> (T button?=w820:bool)  [unwired: 2 in]
            n63 = case shown="True" w820 {
              tunnel: w825 -> [w826 w830]
              tunnel: [w826 w828] -> w824
              frame False {
              }
              frame True {
                w827 = string[][] [] ("Record Table")
                n64 = property on="Record Table" class="Tbl (strict)"(error in=w830, "Value"=w827) -> (error out=w829:errorcluster)  [unwired: 1 in, 1 out]
                n65 = property on="XY Scan List" class="Tbl (strict)"(error in=w829, "Value"=w827) -> (error out=w828:errorcluster)  [unwired: 1 in, 1 out]
              }
            }
            n66 = property on="Clear Table" class="Bool (strict)"(error in=w824, "Value"=FALSE ("Clear Table")) -> (error out=w823:errorcluster)  [unwired: 1 in, 1 out]
          }
          event "Goto destination": Value Change {
            n67 = event-data() -> ()  [unwired: 1 in, 1 out]
            n68 = local read "Record Table"() -> (w831:string[][])
            n69 = property on="ILSID" class="DigNum (strict)"() -> ("Value"=w833:i32)  [unwired: 2 in, 2 out]
            n70 = call "subStage_GotoAccordingtoTable.vi"("Record Table"=w831, "error in (no error)"=w836, "ILSID"=w833, "Number"="Number") -> ("error out"=w835:errorcluster)  [unwired: 7 in]
            n71 = property on="Goto destination" class="Bool (strict)"(error in=w835, "Value"=FALSE ("Goto destination")) -> (error out=w834:errorcluster)  [unwired: 1 in, 1 out]
          }
          event "Write table to excel": Value Change {
            n72 = event-data() -> ()  [unwired: 1 in, 1 out]
            n73 = local read "Excel Loading Path"() -> (w840:path)
            n74 = local read "Record Table"() -> (w843:string[][])
            n75 = call "SubStage_WriteTableToExcel.vi"("Record Table"=w843, "error in (no error)"=w842, "Path"=w840) -> ("error out"=w841:errorcluster)  [unwired: 8 in]
            n76 = property on="Write table to excel" class="Bool (strict)"(error in=w841, "Value"=FALSE ("Write table to excel")) -> (error out=w847:errorcluster)  [unwired: 1 in, 1 out]
          }
          event "Load Excel to table": Value Change {
            n77 = event-data() -> ()  [unwired: 1 in, 1 out]
            n78 = call "subStage_ReadExcelToTable.vi"("error in (no error)"=w851, "File Path"="Excel Loading Path") -> ("error out"=w849:errorcluster, "Record Table"=w852:string[][])  [unwired: 8 in]
            n79 = local write "Record Table"(w852) -> ()
            n80 = property on="Load Excel to table" class="Bool (strict)"(error in=w849, "Value"=FALSE ("Load Excel to table")) -> (error out=w848:errorcluster)  [unwired: 1 in, 1 out]
          }
          event "Load from table (For XY Scan)": Value Change {
            n81 = event-data() -> ()  [unwired: 1 in, 1 out]
            n82 = property on="Record Table" class="Tbl (strict)"(error in=w861) -> (error out=w860:errorcluster, "Value"=w859:string[][])  [unwired: 1 in, 1 out]
            n83 = property on="XY Scan List" class="Tbl (strict)"(error in=w860, "Value"=w859) -> (error out=w858:errorcluster)  [unwired: 1 in, 1 out]
            n84 = property on="Load from table (For XY Scan)" class="Bool (strict)"(error in=w858, "Value"=FALSE ("Load from table (For XY Scan)")) -> (error out=w857:errorcluster)  [unwired: 1 in, 1 out]
          }
          event "Load from Exel (For XY Scan)": Value Change {
            n85 = event-data() -> ()  [unwired: 1 in, 1 out]
            n86 = local read "Excel Loading Path"() -> (w867:path)
            n87 = call "subStage_ReadExcelToTable.vi"("error in (no error)"=w869, "File Path"=w867) -> ("error out"=w866:errorcluster, "Record Table"=w868:string[][])  [unwired: 8 in]
            n88 = local write "XY Scan List"(w868) -> ()
            n89 = property on="Load from Exel (For XY Scan)" class="Bool (strict)"(error in=w866, "Value"=FALSE ("Load Excel to table")) -> (error out=w865:errorcluster)  [unwired: 1 in, 1 out]
          }
          event "Stage on?": Value Change {
            n90 = event-data() -> ("NewVal"=w877:bool)  [unwired: 1 in]
            n91 = case shown="False" w877 {
              tunnel: [w882 w890] -> w878
              tunnel: w876 -> [w881 w891]
              tunnel: [T23."Disabled and Grayed Out" ("Disabled") T23."Enabled" ("Disabled")] -> w875
              tunnel: [FALSE w889] -> w874
              tunnel: [T23."Disabled and Grayed Out" ("Disabled") T23."Enabled" ("Disabled")] -> w873
              tunnel: [T7 {" Current Position"=[-1.0, -12.0, 0.0], "Number of Axis"=3, "ILSID"=1} ("Stage Info") w887] -> w872
              frame False {
                n92 = local read "Stage Status"() -> (w880:T7)
                n93 = call "Disconnect.vi"("Stage Info"=w880, "Error In"=w881) -> ("Error out"=w882:errorcluster)  [unwired: 9 in]
              }
              frame True {
                n94 = property on="Stage setting" class="Clust (strict)"() -> ("Value"=w886:T26)  [unwired: 2 in, 2 out]
                n95 = call "subStage_Initialize.vi"("Stage setting"=w886, "Error In"=w891) -> ("Error out"=w890:errorcluster, "Stage initialized"=w889:bool, "Stage Info"=w887:T7)  [unwired: 7 in]
              }
            }
            n96 = property on="Stage Status" class="Clust (strict)"("Value"=w872) -> ()  [unwired: 2 in, 2 out]
            n97 = property on="Stage initialized" class="Bool (strict)"("Value"=w874) -> ()  [unwired: 2 in, 2 out]
            n98 = property on="Stage Status" class="Clust (strict)"("DisabledEnum"=w873) -> ()  [unwired: 2 in, 2 out]
            n99 = property on="Stage-Ctrl" class="Clust (strict)"("DisabledEnum"=w875) -> ()  [unwired: 2 in, 2 out]
          }
          event "Stage-Ctrl.Move": Value Change {
            n100 = event-data() -> ()  [unwired: 1 in, 1 out]
            n101 = local read "Stage-Ctrl"() -> (w899:T6)
            n102 = property on="Stage setting" class="Clust (strict)"() -> ("Value"=w895:T26)  [unwired: 2 in, 2 out]
            n103 = call "SubStage_MoveLimitation.vi"("Stage-Ctrl"=w899, "Stage setting"=w895) -> ("Allow?"=w903:bool)  [unwired: 9 in]
            n104 = case shown="False" w903 {
              selector: w903 -> [w909 _]
              tunnel: [w909 w910] -> w902
              frame True {
              }
              frame False, Default {
                n105 = Two Button Dialog(message="WARNING: Are you sure?\n It may collide the objective.") -> (T button?=w910:bool)  [unwired: 2 in]
              }
            }
            n106 = local read "Stage Status"() -> (w900:T7)
            n107 = case shown="True" w902 {
              tunnel: w901 -> [w904 w908]
              tunnel: [w904 w907] -> w898
              tunnel: w899 -> [_ w905]
              tunnel: w900 -> [_ w906]
              frame False {
              }
              frame True {
                n108 = call "subStage_MoveAbs.vi"("Stage Info"=w906, "error in (no error)"=w908, "Stage-Ctrl"=w905) -> ("error out"=w907:errorcluster)  [unwired: 8 in]
              }
            }
            n109 = property on="Move" class="Bool (strict)"(error in=w898, "Value"=FALSE ("Move absolute")) -> (error out=w897:errorcluster)  [unwired: 1 in, 1 out]
          }
          event "Calibrate stage": Value Change {
            n110 = event-data() -> ()  [unwired: 1 in, 1 out]
            n111 = local read "TiE Ref"() -> (w915:T21)
            n112 = local read "TI-Ctrl"() -> (w914:T9)
            n113 = call "subTiE_SetZEscape.vi"("Wait for a second? (F)"=TRUE, "Ref"=w915, "TI-Ctrl"=w914, "error in"=w921) -> ("error out"=w920:errorcluster)  [unwired: 7 in]
            n114 = local read "Stage Status"() -> (w919:T7)
            n115 = call "subStage_Calibrate.vi"("Stage Info"=w919, "error in (no error)"=w920) -> ("error out"=w917:errorcluster, "Calibrate"=w918:bool)  [unwired: 7 in]
            n116 = property on="Calibrate stage" class="Bool (strict)"("Value"=w918) -> ()  [unwired: 2 in, 2 out]
          }
          event "Stage-Ctrl.Console": Value Change {
            n117 = event-data() -> ()  [unwired: 1 in, 1 out]
            n118 = local read "Stage Status"() -> (w927:T7)
            n119 = local read "Stage-Ctrl"() -> (w924:T6)
            n120 = call "subStage_MoveRelative.vi"("Stage-Ctrl"=w924, "error in"=w928, "Stage Info"=w927) -> ("error out"=w926:errorcluster, "Console Out"=w925:T27)  [unwired: 7 in]
            n121 = property on="Console" class="Clust (strict)"("Value"=w925) -> ()  [unwired: 2 in, 2 out]
          }
        }
        "Stage" <- w787
        n122 = local read "stop program"() -> (w788:bool)
      }
      n123 = while {
        stop <- w629 stop-if-true
        # "Calculations"
        n124 = event shown="[11] \"Generate Tiling\": Value Change" {
          selector: _ -> [_ _ _ _ _ _ _ _ _ _ _ _]
          dyn-events: _ -> [_ _ _ _ _ _ _ _ _ _ _ _]
          timeout: 50 -> [_ _ _ _ _ _ _ _ _ _ _ _]
          event Timeout {
            n125 = event-data() -> ()  [unwired: 1 in, 1 out]
            n126 = local read "Camera on?"() -> (w631:bool)
            n127 = case shown="True" w631 {
              frame False {
              }
              frame True {
                n128 = property on="ROI define" class="Bool (strict)"() -> ("Value"=w633:bool)  [unwired: 2 in, 2 out]
                n129 = property on="Autoscale" class="Bool (strict)"() -> ("Value"=w632:bool)  [unwired: 2 in, 2 out]
                n130 = case shown="True" w633 {
                  frame False {
                  }
                  frame True {
                    # "set ROI cursor"
                    # "calculate frame rate\nbased on cursor"
                    # "update cursor info"
                    n131 = control-ref of="Image"() -> (w635:refnum<vi>)
                    n132 = property on="ROI" class="Clust (strict)"() -> ("Value"=w638:T3)  [unwired: 2 in, 2 out]
                    n133 = property on="Symmetrical" class="Bool (strict)"() -> ("Value"=w636:bool)  [unwired: 2 in, 2 out]
                    n134 = call "subImage_ApplyCursorLimit.vi"("Symmetrical ROI"=w636, "IntGraph Refnum"=w635, "Current ROI"=w638) -> ("ROI cursor"=w634:T3)  [unwired: 8 in]
                    "ROI cursor" <- w634
                    n135 = call "subHamamatsu_GetMaxFrameRate.vi"("ROI in"=w634) -> ("max frame rate (Hz)"=w637:dbl)  [unwired: 8 in, 2 out]
                    n136 = property on="max frame rate (Hz)" class="DigNum (strict)"("Value"=w637) -> ()  [unwired: 2 in, 2 out]
                  }
                }
                n137 = case shown="False" w632 {
                  frame False {
                    # "update cursor info"
                    n138 = control-ref of="Image"() -> (w641:refnum<vi>)
                    n139 = control-ref of="Histogram"() -> (w640:refnum<vi>)
                    n140 = call "subHistogram_ApplyScaleLimit.vi"("IntGraph Refnum"=w641, "XYGraph Refnum"=w640) -> ("Scale"=w639:cluster{"Scale.Min":i32, "Scale.Max":i32})  [unwired: 8 in, 1 out]
                    n141 = property on="Scale" class="Clust (strict)"("Value"=w639) -> ()  [unwired: 2 in, 2 out]
                  }
                  frame True {
                  }
                }
              }
            }
          }
          event "Camera Ctrl.ROI define": Value Change {
            n142 = event-data() -> ("NewVal"=w642:bool)  [unwired: 1 in]
            n143 = case shown="True" w642 {
              frame False {
                w644 = FALSE ("Visible")
                # "hide cursors from image graph"
                n144 = property on="Image" class="IntGraph (strict)"("Active Cursor"=u32 0, "Cursor.Visible"=w644) -> ()  [unwired: 2 in, 2 out]
                n145 = property on="Image" class="IntGraph (strict)"("Active Cursor"=u32 1, "Cursor.Visible"=w644) -> ()  [unwired: 2 in, 2 out]
              }
              frame True {
                w646 = TRUE ("Visible")
                n146 = property on="Image" class="IntGraph (strict)"() -> ("XScale.Minimum"=w651:dbl, "YScale.Maximum"=w650:dbl, "XScale.Maximum"=w649:dbl, "YScale.Minimum"=w648:dbl)  [unwired: 2 in, 2 out]
                n147 = property on="Image" class="IntGraph (strict)"("Active Cursor"=u32 0, "Cursor.Visible"=w646, "Cursor.Cursor X"=w651, "Cursor.Cursor Y"=w650) -> ()  [unwired: 2 in, 2 out]
                n148 = property on="Image" class="IntGraph (strict)"("Active Cursor"=u32 1, "Cursor.Visible"=w646, "Cursor.Cursor X"=w649, "Cursor.Cursor Y"=w648) -> ()  [unwired: 2 in, 2 out]
              }
            }
          }
          event "Timelapse?": Value Change {
            n149 = event-data() -> ()  [unwired: 1 in, 1 out]
            n150 = Select(t=T23."Enabled" ("Disabled"), s="Timelapse?", f=T23."Disabled and Grayed Out" ("Disabled")) -> (s? t:f=w653:T23)
            n151 = property on="Timelapse Wait (s)" class="DigNum (strict)"("DisabledEnum"=w653) -> ()  [unwired: 2 in, 2 out]
            n152 = property on="Timelapse Cycles" class="DigNum (strict)"("DisabledEnum"=w653) -> ()  [unwired: 2 in, 2 out]
          }
          event "Camera Ctrl.Autoscale": Value Change {
            n153 = event-data() -> ("NewVal"=w659:bool)  [unwired: 1 in]
            n154 = case shown="False" w659 {
              tunnel: [T23."Enabled" ("Disabled") T23."Disabled and Grayed Out" ("Disabled")] -> w657
              tunnel: [u8 0 ("X Scale.Scale Fit") u8 2 ("X Scale.Scale Fit")] -> w658
              frame False {
                # "autoscale OFF"
                # "initialize scale cursors to\nthe current histogram"
                n155 = property on="Histogram" class="XYGraph (strict)"() -> ("XScale.Minimum"=w664:dbl, "XScale.Maximum"=w660:dbl)  [unwired: 2 in, 2 out]
                n156 = property on="Histogram" class="XYGraph (strict)"("Active Cursor"=u32 0, "Cursor.Visible"=TRUE, "Cursor.Cursor X"=w664, "Cursor.Cursor Y"=-1000.0 ("y")) -> ()  [unwired: 2 in, 2 out]
                n157 = property on="Histogram" class="XYGraph (strict)"("Active Cursor"=u32 1, "Cursor.Visible"=TRUE, "Cursor.Cursor X"=w660, "Cursor.Cursor Y"=-1000.0 ("y")) -> ()  [unwired: 2 in, 2 out]
              }
              frame True {
                w670 = FALSE ("Visible")
                # "autoscale ON"
                # "hide cursors from image graph"
                n158 = property on="Histogram" class="XYGraph (strict)"("Active Cursor"=u32 0, "Cursor.Visible"=w670) -> ()  [unwired: 2 in, 2 out]
                n159 = property on="Histogram" class="XYGraph (strict)"("Active Cursor"=u32 1, "Cursor.Visible"=w670) -> ()  [unwired: 2 in, 2 out]
              }
            }
            n160 = property on="Histogram" class="XYGraph (strict)"("XScale.ScaleFit"=w658) -> ()  [unwired: 2 in, 2 out]
            n161 = property on="Image" class="IntGraph (strict)"("ZScale.ScaleFit"=w658) -> ()  [unwired: 2 in, 2 out]
            n162 = property on="Scale" class="Clust (strict)"("DisabledEnum"=w657) -> ()  [unwired: 2 in, 2 out]
          }
          event "Camera Ctrl.Scale": Value Change {
            n163 = event-data() -> ("NewVal"=w681:cluster{"Scale.Min":i32, "Scale.Max":i32})  [unwired: 1 in]
            n164 = Unbundle By Name(w681) -> ("Scale.Min"=w679:i32, "Scale.Max"=w675:i32)
            n165 = property on="Histogram" class="XYGraph (strict)"("Active Cursor"=u32 0, "Cursor.Visible"=TRUE, "Cursor.Cursor X"=w679) -> ()  [unwired: 2 in, 2 out]
            n166 = property on="Histogram" class="XYGraph (strict)"("Active Cursor"=u32 1, "Cursor.Visible"=TRUE, "Cursor.Cursor X"=w675) -> ()  [unwired: 2 in, 2 out]
            n167 = property on="Image" class="IntGraph (strict)"("ZScale.Minimum"=w679, "ZScale.Maximum"=w675) -> ()  [unwired: 2 in, 2 out]
          }
          event "Cal step num": Value Change {
            n168 = event-data() -> ()  [unwired: 1 in, 1 out]
            n169 = local read "Z-Stack"() -> (w689:T10)
            n170 = Unbundle By Name(w689) -> ("Z end"=w688:dbl, "Z0"=w687:dbl, "Step Size"=w686:dbl)
            n171 = Subtract(x=w688, y=w687) -> (x-y=w690:dbl)
            n172 = Divide(x=w690, y=w686) -> (x/y=w685:dbl)
            n173 = local read "Z-Stack"() -> (w684:T10)
            n174 = Bundle By Name(cluster=w684, "Step Num"=w685) -> (w683:T10)
            n175 = local write "Z-Stack"(w683) -> ()
            n176 = local write "Cal step size"(FALSE) -> ()
          }
          event "Cal step size": Value Change {
            n177 = event-data() -> ()  [unwired: 1 in, 1 out]
            n178 = local read "Z-Stack"() -> (w697:T10)
            n179 = Unbundle By Name(w697) -> ("Z end"=w696:dbl, "Z0"=w695:dbl, "Step Num"=w694:i32)
            n180 = Subtract(x=w696, y=w695) -> (x-y=w699:dbl)
            n181 = Divide(x=w699, y=w694) -> (x/y=w693:dbl)
            n182 = local read "Z-Stack"() -> (w692:T10)
            n183 = Bundle By Name(cluster=w692, "Step Size"=w693) -> (w691:T10)
            n184 = local write "Z-Stack"(w691) -> ()
            n185 = local write "Cal step size"(FALSE) -> ()
          }
          event "# frames": Value Change {
            n186 = event-data() -> ()  [unwired: 1 in, 1 out]
            n187 = local read "Movie frame rate (Hz)"() -> (w700:dbl)
            n188 = Divide(x="# frames", y=w700) -> (x/y=w702:dbl)
            n189 = local write "Total time (sec)"(w702) -> ()
          }
          event "Total time (sec)": Value Change {
            n190 = event-data() -> ()  [unwired: 1 in, 1 out]
            n191 = local read "Movie frame rate (Hz)"() -> (w703:dbl)
            n192 = Multiply(x="Total time (sec)", y=w703) -> (x*y=w705:dbl)
            n193 = Round To Nearest(number=w705) -> (nearest integer value=w704:dbl)
            n194 = Divide(x=w704, y=w703) -> (x/y=w707:dbl)
            n195 = local write "# frames"(w704) -> ()
            n196 = local write "Total time (sec)"(w707) -> ()
          }
          event "Movie frame rate (Hz)": Value Change {
            n197 = event-data() -> ()  [unwired: 1 in, 1 out]
            n198 = local read "# frames"() -> (w710:i32)
            n199 = Divide(x=w710, y="Movie frame rate (Hz)") -> (x/y=w708:dbl)
            n200 = local write "Total time (sec)"(w708) -> ()
          }
          event "Scope on?", "Camera on?", "TI-Ctrl.Obj": Value Change {
            n201 = event-data() -> ()  [unwired: 1 in, 1 out]
            n202 = control-ref of="Pixel size (nm)"() -> (w715:refnum<vi>)
            n203 = control-ref of="Total y width (μm)"() -> (w714:refnum<vi>)
            n204 = control-ref of="scale bar (μm)"() -> (w712:refnum<vi>)
            n205 = control-ref of="Total x width (μm)"() -> (w713:refnum<vi>)
            n206 = local read "TI-Ctrl"() -> (w717:T9)
            n207 = property on="ROI" class="Clust (strict)"() -> ("Value"=w716:T3)  [unwired: 2 in, 2 out]
            n208 = Bundle("Total x width (μm)"=w713, "Total y width (μm)"=w714, "Pixel size (nm)"=w715, "scale bar (μm)"=w712) -> (w711:T28)  [unwired: 1 in]
            n209 = call "subCalculate_SetScaleBar.vi"("ROI in"=w716, "Scale calculation cluster"=w711, "TI-Ctrl"=w717) -> ()  [unwired: 7 in, 2 out]
          }
          event "Generate Tiling": Value Change {
            n210 = event-data() -> ()  [unwired: 1 in, 1 out]
            n211 = case shown="0, Default" "Ranking" {
              frame 0, Default {
                n212 = property on="Record Table" class="Tbl (strict)"() -> (error out=w719:errorcluster, "Value"=w722:string[][])  [unwired: 2 in, 1 out]
                n213 = property on="XY Scan List" class="Tbl (strict)"(error in=w719, "Value"=w722) -> (error out=w720:errorcluster)  [unwired: 1 in, 1 out]
                n214 = property on="Generate Tiling" class="Bool (strict)"(error in=w720, "Value"=FALSE ("Generate Tiling")) -> ()  [unwired: 1 in, 2 out]
              }
              frame 1 {
                n215 = local read "XY Scan List"() -> (w726:string[][])
                n216 = call "subStage_GetMinimumMovingDistance.vi"("XY Scan List"=w726) -> ("error out"=w724:errorcluster, "XY Scan List (reorder)"=w725:string[][])  [unwired: 9 in]
                n217 = local write "XY Scan List"(w725) -> ()
                n218 = property on="Generate Tiling" class="Bool (strict)"(error in=w724, "Value"=FALSE ("Generate Tiling")) -> ()  [unwired: 1 in, 2 out]
              }
              frame 2 {
                n219 = local write "XY Scan List"(string[][] [] ("XY Scan List")) -> ()
                n220 = property on="Generate Tiling" class="Bool (strict)"("Value"=FALSE ("Generate Tiling")) -> ()  [unwired: 2 in, 2 out]
              }
            }
          }
        }
        n221 = local read "stop program"() -> (w629:bool)
      }
      n222 = while {
        stop <- w50 stop-if-true
        # "Patch tuning"
        n223 = event shown="[2] \"Save patch param\": Value Change" {
          selector: _ -> [_ _ _]
          dyn-events: _ -> [_ _ _]
          timeout: 50 -> [_ _ _]
          event Timeout {
            n224 = event-data() -> ()  [unwired: 1 in, 1 out]
          }
          event "Test patch": Value Change {
            n225 = event-data() -> ()  [unwired: 1 in, 1 out]
            n226 = property on="DAQ ports" class="Clust (strict)"() -> ("Value"=w52:T25)  [unwired: 2 in, 2 out]
            n227 = call "subAxopatch_PatchParams.vi"("DAQ ports"=w52, "Pipet tuning parameters"="Pipet tuning parameters") -> ("Error out"=w58:errorcluster, "Average I-t curve"=→"Average I-t curve":cluster{"xo":i32, dbl, dbl[]}, "Patch output"=→"Patch output":cluster{"xo":i32, dbl, "data":dbl[][]}, "Patch quality"=→"Patch quality":T29, "Seal test DAQ params"=→"Seal test DAQ params":T15, "Patch seal test waveform"=→"Patch seal test waveform":waveform(dbl))  [unwired: 4 in]
            n228 = case shown="No Error" w58 {
              frame No Error {
                n229 = local write "Test patch"(FALSE ("Test patch")) -> ()
              }
              frame Error {
              }
            }
          }
          event "Save patch param": Value Change {
            n230 = event-data() -> ()  [unwired: 1 in, 1 out]
            n231 = flat-sequence {
              frame #0 {
                n232 = local read "Patch output"() -> (w61:cluster{"xo":i32, dbl, "data":dbl[][]})
                n233 = local read "Base folder"() -> (w63:path)
                n234 = local read "Patch quality"() -> (w62:T17)
                n235 = call "subSave_PatchParams_New.vi"("Scaled output"=w61, "Patch quality"=w62, "Base path"=w63) -> ()  [unwired: 9 in]
              }
              frame #1 {
                n236 = local write "Save patch param"(FALSE ("Save patch param")) -> ()
              }
            }
          }
        }
        n237 = local read "stop program"() -> (w50:bool)
      }
      n238 = while {
        shift-right: [w65] -> _
        shift-left: T22 {"width"=0, "height"=0, "datatype"=0} ("Buffer") -> [w69]
        shift-right: [w68] -> w36
        shift-left: errorcluster {"status"=FALSE, "code"=0, "source"=""} ("camera \ninitialization\nerror") -> [w67]
        stop <- "stop program" stop-if-true
        # "Camera"
        n239 = event shown="[5] \"Camera Ctrl.ROI update\": Value Change" {
          selector: _ -> [_ _ _ _ _ _ _ _ _ _ _ _]
          dyn-events: _ -> [_ _ _ _ _ _ _ _ _ _ _ _]
          timeout: 50 -> [_ _ _ _ _ _ _ _ _ _ _ _]
          tunnel: w69 -> [w77 w88 _ _ _ _ _ _ w386 _ _ _]
          tunnel: w67 -> [w76 w91 w158 w228 w259 w308 w351 w381 w387 w402 w468 w526]
          tunnel: [w75 w90 w159 w227 w258 w307 w350 w380 w389 w401 w463 w525] -> w68
          tunnel: [w71 w89 _ w223 w240 w302 w344 w376 w386 w399 w461 w524] -> w65
          event Timeout {
            n240 = event-data() -> ()  [unwired: 1 in, 1 out]
            n241 = local read "Camera on?"() -> (w74:bool)
            n242 = property on="Live" class="Bool (strict)"() -> ("Value"=w72:bool)  [unwired: 2 in, 2 out]
            n243 = And(x=w74, y=w72) -> (x .and. y?=w73:bool)
            n244 = case shown="True" w73 {
              tunnel: w76 -> [w79 w84]
              tunnel: [w79 w86] -> w75
              tunnel: w77 -> [w78 w85]
              tunnel: [w78 w85] -> w71
              frame False {
              }
              frame True {
                n245 = property on="Handle" class="DigNum (strict)"() -> ("Value"=w83:u32)  [unwired: 2 in, 2 out]
                n246 = property on="ROI" class="Clust (strict)"() -> ("Value"=w82:T3)  [unwired: 2 in, 2 out]
                n247 = call "subHamamatsu_UpdateImageInfo.vi"("ROI"=w82, "Error In"=w84, "Image Buffer"=w85, "Handle in"=w83) -> ("Error out"=w86:errorcluster, "Histogram"=w80:T30, "Image out"=w81:u16[][])  [unwired: 5 in]
                n248 = property on="Image" class="IntGraph (strict)"("Value"=w81) -> ()  [unwired: 2 in, 2 out]
                n249 = property on="Histogram" class="Clust (strict)"("Value"=w80) -> ()  [unwired: 2 in, 2 out]
              }
            }
          }
          event "Camera Ctrl.Chosen Camera": Value Change {
            # "Disable and grey out Camera Chosen"
            n250 = event-data() -> ("NewVal"=w87:u32)  [unwired: 1 in]
            n251 = case shown="0, Default" w87 {
              tunnel: w91 -> [w98 w128]
              tunnel: [w97 w129] -> w90
              tunnel: [w95 w127] -> w89
              tunnel: w88 -> [w96 w130]
              frame 0, Default {
                # "Left camera initialized?"
                n252 = local read "Camera initialized"() -> (w93:bool[])
                n253 = Index Array(array=w93, index=0) -> (element=w92:bool)
                n254 = case shown="True" w92 {
                  tunnel: w98 -> [w103 w116]
                  tunnel: [w103 w107] -> w97
                  tunnel: w96 -> [w99 _]
                  tunnel: [w99 w106] -> w95
                  frame False {
                    n255 = One Button Dialog(message="Please turn on the Left camera first!", button name ("OK")="OK") -> ()  [unwired: 1 out]
                    n256 = property on="Chosen Camera" class="Ring (strict)"("Value"=u32 1) -> ()  [unwired: 2 in, 2 out]
                  }
                  frame True {
                    # "open and set new camera"
                    # "Chosen camera = 0 --> left camera\nTurn of Global shutter to block epi-illumination"
                    n257 = local read "Light control"() -> (w122:T1)
                    n258 = property on="DAQ ports" class="Clust (strict)"() -> ("Value"=w105:T25)  [unwired: 2 in, 2 out]
                    n259 = Bundle By Name(cluster=w122, "Global"=FALSE ("new element/subarray")) -> (w121:T1)
                    n260 = call "subDAQ_SetGlobal.vi"("DAQ ports"=w105, "Light control (All off)"=w121) -> ()  [unwired: 9 in, 1 out]
                    n261 = local write "Light control"(w121) -> ()
                    n262 = property on="Handle" class="DigNum (strict)"() -> ("Value"=w114:u32)  [unwired: 2 in, 2 out]
                    n263 = call "subHamamatsu_CloseCam.vi"("Live"=TRUE, "error in (no error)"=w116, "Handle in"=w114) -> ("error out"=w117:errorcluster)  [unwired: 8 in]
                    n264 = property on="ROI" class="Clust (strict)"() -> ("Value"=w118:T3)  [unwired: 2 in, 2 out]
                    n265 = property on="Exposure (ms)" class="DigNum (strict)"() -> ("Value"=w119:dbl)  [unwired: 2 in, 2 out]
                    n266 = property on="Chosen Camera" class="Ring (strict)"() -> ("Value"=w115:u32)  [unwired: 2 in, 2 out]
                    n267 = property on="Camera Setting" class="Clust (strict)"() -> ("Value"=w104:T31)  [unwired: 2 in, 2 out]
                    n268 = call "subHamamatsu_OpenCam.vi"("Exposure (ms)"=w119, "ROI"=w118, "error in (no error)"=w117, "Camera Setting"=w104, "Handle in"=w115) -> ("error out"=w112:errorcluster, "Camera in use"=w120:T32, "Handle out"=w111:u32)  [unwired: 4 in]
                    n269 = property on="Camera in use" class="Clust (strict)"("Value"=w120) -> ()  [unwired: 2 in, 2 out]
                    n270 = property on="Live" class="Bool (strict)"() -> ("Value"=w109:bool)  [unwired: 2 in, 2 out]
                    n271 = call "subHamamatsu_TurnOnOff.vi"("logic 2"=TRUE ("logic 1"), "logic 1"=w109, "error in (no error)"=w112, "Handle in"=w111) -> ("error out"=w107:errorcluster, "Buffer"=w106:T22, "Handle out"=w110:u32)  [unwired: 5 in]
                    n272 = property on="Handle" class="DigNum (strict)"("Value"=w110) -> ()  [unwired: 2 in, 2 out]
                  }
                }
              }
              frame 1 {
                # "Right camera intialized?"
                # "handle 0 = left (S/N: 003222)\nhandle 1 = right (S/N: 003223)"
                n273 = local read "Camera initialized"() -> (w125:bool[])
                n274 = Index Array(array=w125, index=1) -> (element=w124:bool)
                n275 = case shown="True" w124 {
                  tunnel: w128 -> [w135 w147]
                  tunnel: [w135 w143] -> w129
                  tunnel: w130 -> [w131 _]
                  tunnel: [w131 w139] -> w127
                  frame False {
                    n276 = One Button Dialog(message="Please turn on the Right camera first!", button name ("OK")="OK") -> ()  [unwired: 1 out]
                    n277 = property on="Chosen Camera" class="Ring (strict)"("Value"=u32 0) -> ()  [unwired: 2 in, 2 out]
                  }
                  frame True {
                    # "open and set new camera"
                    n278 = property on="Handle" class="DigNum (strict)"() -> ("Value"=w145:u32)  [unwired: 2 in, 2 out]
                    n279 = call "subHamamatsu_CloseCam.vi"("Live"=TRUE, "error in (no error)"=w147, "Handle in"=w145) -> ("error out"=w148:errorcluster)  [unwired: 8 in]
                    n280 = property on="Chosen Camera" class="Ring (strict)"() -> ("Value"=w146:u32)  [unwired: 2 in, 2 out]
                    n281 = property on="Camera Setting" class="Clust (strict)"() -> ("Value"=w136:T31)  [unwired: 2 in, 2 out]
                    n282 = property on="ROI" class="Clust (strict)"() -> ("Value"=w149:T3)  [unwired: 2 in, 2 out]
                    n283 = property on="Exposure (ms)" class="DigNum (strict)"() -> ("Value"=w150:dbl)  [unwired: 2 in, 2 out]
                    n284 = call "subHamamatsu_OpenCam.vi"("Exposure (ms)"=w150, "ROI"=w149, "error in (no error)"=w148, "Camera Setting"=w136, "Handle in"=w146) -> ("error out"=w142:errorcluster, "Camera in use"=w151:T32, "Handle out"=w138:u32)  [unwired: 4 in]
                    n285 = property on="Camera in use" class="Clust (strict)"("Value"=w151) -> ()  [unwired: 2 in, 2 out]
                    n286 = property on="Live" class="Bool (strict)"() -> ("Value"=w141:bool)  [unwired: 2 in, 2 out]
                    n287 = call "subHamamatsu_TurnOnOff.vi"("logic 2"=TRUE ("logic 1"), "logic 1"=w141, "error in (no error)"=w142, "Handle in"=w138) -> ("error out"=w143:errorcluster, "Buffer"=w139:T22, "Handle out"=w137:u32)  [unwired: 5 in]
                    n288 = property on="Handle" class="DigNum (strict)"("Value"=w137) -> ()  [unwired: 2 in, 2 out]
                  }
                }
              }
            }
          }
          event "Camera on?": Value Change {
            n289 = event-data() -> ("NewVal"=w157:bool)  [unwired: 1 in]
            n290 = case shown="True" w157 {
              tunnel: [w171 w181] -> w159
              tunnel: w158 -> [w170 w177]
              tunnel: [FALSE FALSE] -> w154
              tunnel: [bool[] [FALSE, FALSE] ("Camera initialized") w175] -> w156
              tunnel: [T23."Disabled and Grayed Out" ("Disabled") w176] -> w155
              tunnel: ["Ready" ("Status") w173] -> w153
              tunnel: [u32 0 ("Handle out") w172] -> w152
              frame False {
                # "First, stop live capture.  Then deinitialize camera."
                n291 = property on="Handle" class="DigNum (strict)"() -> ("Value"=w163:u32)  [unwired: 2 in, 2 out]
                n292 = property on="Live" class="Bool (strict)"() -> ("Value"=w164:bool)  [unwired: 2 in, 2 out]
                n293 = call "subHamamatsu_TurnOnOff.vi"("logic 2"=FALSE, "logic 1"=w164, "error in (no error)"=w170, "Handle in"=w163) -> ("error out"=w169:errorcluster, "Handle out"=w162:u32)  [unwired: 5 in, 1 out]
                n294 = call "subHamamatsu_Deinitialization.vi"("error in (no error)"=w169, "Handle"=w162) -> ("error out"=w171:errorcluster)  [unwired: 9 in]
              }
              frame True {
                # "If no camera is initialized, report error.\nIf only 1 camera is initialized, use that one.\nIf both cameras are initialized, choose camera."
                n295 = flat-sequence {
                  tunnel: [w186] -> w179
                  tunnel: [w191] -> w178
                  tunnel: w177 -> [w190]
                  tunnel: [w188] -> w175
                  tunnel: [w189] -> w174
                  frame #0 {
                    n296 = local read "Camera Ctrl"() -> (w185:T8)
                    n297 = property on="Camera Setting" class="Clust (strict)"() -> ("Value"=w182:T31)  [unwired: 2 in, 2 out]
                    n298 = property on="Status" class="Str"("Value"="Initializing Camera ..." ("Status")) -> ()  [unwired: 2 in, 2 out]
                    n299 = call "subHamamatsu_Initialization.vi"("Camera Ctrl"=w185, "error in (no error)"=w190, "Camera Setting"=w182) -> ("error out"=w191:errorcluster, "Chosen Camera"=w183:u32, "Handle out"=w186:u32, "Camera Info"=w184:T19, "Number Of Cameras"=w189:u32, "Camera initialized"=w188:bool[])  [unwired: 3 in]
                    n300 = local write "Camera Info"(w184) -> ()
                    n301 = property on="Chosen Camera" class="Ring (strict)"("Value"=w183) -> ()  [unwired: 2 in, 2 out]
                  }
                }
                n302 = case shown="1, 2" w174 {
                  tunnel: w178 -> [w196 w219]
                  tunnel: w179 -> [w193 w217]
                  tunnel: [w196 w199] -> w181
                  tunnel: [T23."Disabled and Grayed Out" ("Disabled") T23."Enabled" ("Disabled")] -> w176
                  tunnel: [w193 w197] -> w172
                  tunnel: ["Camera not detected." ("Status") "Ready" ("Status")] -> w173
                  frame 0, Default {
                    n303 = property on="Camera on?" class="Bool (strict)"("Value"=FALSE ("Camera on?")) -> ()  [unwired: 2 in, 2 out]
                  }
                  frame 1, 2 {
                    # "initialize image"
                    n304 = control-ref of="Camera View indicator"() -> (w210:refnum<vi>)
                    n305 = control-ref of="Image"() -> (w211:refnum<vi>)
                    n306 = call "subImage_InitializeImage.vi"("error in (no error)"=w219, "Handle in"=w217) -> ("error out"=w218:errorcluster, "Handle out"=w216:u32)  [unwired: 7 in, 1 out]
                    n307 = property on="ROI" class="Clust (strict)"() -> ("Value"=w213:T3)  [unwired: 2 in, 2 out]
                    n308 = call "subHamamatsu_SetROI.vi"("ROI"=w213, "error in (no error)"=w218, "Handle in"=w216) -> ("error out"=w203:errorcluster, "Handle out"=w204:u32)  [unwired: 6 in, 1 out]
                    n309 = property on="Autoscale" class="Bool (strict)"("Value"=TRUE ("Autoscale")) -> ()  [unwired: 2 in, 2 out]
                    n310 = call "subImage_UpdateLocIndicator.vi"("Camera View Indicator Ref"=w210, "Image Refnum"=w211, "ROI"=w213, "error in"=w203, "Handle in"=w204) -> ("error out"=w202:errorcluster, "Handle out"=w201:u32)  [unwired: 5 in]
                    n311 = control-ref of="Pixel size (nm)"() -> (w208:refnum<vi>)
                    n312 = control-ref of="Total y width (μm)"() -> (w207:refnum<vi>)
                    n313 = control-ref of="scale bar (μm)"() -> (w209:refnum<vi>)
                    n314 = control-ref of="Total x width (μm)"() -> (w206:refnum<vi>)
                    n315 = local read "TI-Ctrl"() -> (w214:T9)
                    n316 = Bundle("Total x width (μm)"=w206, "Total y width (μm)"=w207, "Pixel size (nm)"=w208, "scale bar (μm)"=w209) -> (w205:T28)  [unwired: 1 in]
                    n317 = call "subCalculate_SetScaleBar.vi"("ROI in"=w213, "Scale calculation cluster"=w205, "TI-Ctrl"=w214, "error in"=w202, "Handle in"=w201) -> ("error out"=w200:errorcluster, "Handle out"=w198:u32)  [unwired: 5 in]
                    n318 = call "subHamamatsu_GetMaxFrameRate.vi"("ROI in"=w213, "error in"=w200, "Handle in"=w198) -> ("error out"=w199:errorcluster, "Handle out"=w197:u32, "max frame rate (Hz)"=w215:dbl)  [unwired: 6 in]
                    n319 = property on="max frame rate (Hz)" class="DigNum (strict)"("Value"=w215) -> ()  [unwired: 2 in, 2 out]
                  }
                }
              }
            }
            "Camera initialized" <- w156
            n320 = property on="Live" class="Bool (strict)"("Value"=w154) -> ()  [unwired: 2 in, 2 out]
            n321 = property on="Camera Ctrl" class="Clust (strict)"("DisabledEnum"=w155) -> ()  [unwired: 2 in, 2 out]
            n322 = property on="Status" class="Str"("Value"=w153) -> ()  [unwired: 2 in, 2 out]
            n323 = property on="Handle" class="DigNum (strict)"("Value"=w152) -> ()  [unwired: 2 in, 2 out]
          }
          event "Camera Ctrl.Live": Value Change {
            n324 = event-data() -> ()  [unwired: 1 in, 1 out]
            n325 = property on="Handle" class="DigNum (strict)"() -> ("Value"=w222:u32)  [unwired: 2 in, 2 out]
            n326 = property on="Live" class="Bool (strict)"() -> ("Value"=w225:bool)  [unwired: 2 in, 2 out]
            n327 = call "subHamamatsu_TurnOnOff.vi"("logic 2"=w225, "logic 1"=TRUE ("Status pre"), "error in (no error)"=w228, "Handle in"=w222) -> ("error out"=w227:errorcluster, "Buffer"=w223:T22)  [unwired: 5 in, 1 out]
            n328 = case shown="False" w225 {
              tunnel: ["Ready" ("Status") "Camera live" ("Status")] -> w224
              frame False {
              }
              frame True {
              }
            }
            n329 = property on="Status" class="Str"("Value"=w224) -> ()  [unwired: 2 in, 2 out]
          }
          event "Camera Ctrl.Snap": Value Change {
            w257 = TRUE ("Snap&Save")
            # "Resume camera"
            # "Turn off camera"
            n330 = event-data() -> ()  [unwired: 1 in, 1 out]
            n331 = property on="Live" class="Bool (strict)"() -> ("Value"=w252:bool)  [unwired: 2 in, 2 out]
            n332 = property on="Handle" class="DigNum (strict)"() -> ("Value"=w239:u32)  [unwired: 2 in, 2 out]
            n333 = call "subHamamatsu_TurnOnOff.vi"("logic 2"=FALSE, "logic 1"=w252, "error in (no error)"=w259, "Handle in"=w239) -> ("error out"=w261:errorcluster, "Handle out"=w238:u32)  [unwired: 5 in, 1 out]
            n334 = call "subHamamatsu_Snapshot.vi"("Error in"=w261, "Value"=w238) -> ("Error out"=w251:errorcluster, "Image"=w237:u16[][], "Handle out"=w255:u32)  [unwired: 7 in]
            n335 = property on="ROI" class="Clust (strict)"() -> ("Value"=w236:T3)  [unwired: 2 in, 2 out]
            n336 = local read "Camera Ctrl"() -> (w231:T8)
            n337 = call "subImage_Pad.vi"("ROI"=w236, "Image in"=w237) -> ("Image out"=w235:u16[][])  [unwired: 7 in, 2 out]
            n338 = property on="DAQ ports" class="Clust (strict)"() -> ("Value"=w234:T25)  [unwired: 2 in, 2 out]
            n339 = property on="Image" class="IntGraph (strict)"("Value"=w235) -> ()  [unwired: 2 in, 2 out]
            n340 = local read "Camera Info"() -> (w232:T19)
            n341 = local read "Base folder"() -> (w264:path)
            n342 = local read "Image Info"() -> (w245:T2)
            n343 = local read "Confocal scanner"() -> (w247:T5)
            n344 = local read "TI-Ctrl"() -> (w244:T9)
            n345 = call "subDAQ_SetLaserDO.vi"("DAQ ports"=w234, "Error in (no error)"=w251) -> ("Error out"=w254:errorcluster)  [unwired: 9 in]
            n346 = call <vilib>:"Check if File or Folder Exists.vi"("path"=w264) -> ("file or folder exists?"=w263:bool, "dup path"=w262:path)  [unwired: 8 in, 1 out]
            n347 = local read "Stage Status"() -> (w246:T7)
            n348 = local read "Light control"() -> (w248:T1)
            n349 = case shown="True" w263 {
              tunnel: w262 -> [w276 w277]
              tunnel: [w275 w277] -> w256
              frame False {
                n350 = Create Folder(path (use dialog)=w276) -> (created path=w275:path)  [unwired: 2 in, 2 out]
              }
              frame True {
              }
            }
            n351 = call "subAcquisition_Info.vi"("Stage Status"=w246, "Light control"=w248, "Image Info"=w245, "Confocal scanner"=w247, "TI-Ctrl"=w244, "Camera Info"=w232, "Camera Ctrl"=w231) -> ("Text"=w249:string)  [unwired: 4 in]
            n352 = call "subSave_Img2Tiff.vi"("Open file dialog? (F)"=w257, "Save Text file? (F)"=w257, "Error in (no error)"=w254, "text"=w249, "Image"=w237, "File path/name"=w256) -> ("Error out"=w243:errorcluster, "Cancel or not?"=w233:bool)  [unwired: 4 in]
            n353 = local read "Light control"() -> (w253:T1)
            n354 = property on="Snap" class="Bool (strict)"(error in=w243, "Value"=FALSE ("Snap&Save")) -> (error out=w242:errorcluster)  [unwired: 1 in, 1 out]
            n355 = case shown="False" w233 {
              frame False {
                n356 = control-ref of="Snap Point  Y Array"() -> (w267:refnum<vi>)
                n357 = control-ref of="Snap Point  X Array"() -> (w268:refnum<vi>)
                n358 = control-ref of="Snap Number Counting"() -> (w269:refnum<vi>)
                n359 = control-ref of="Record Table"() -> (w266:refnum<vi>)
                n360 = property on="Stage Status" class="Clust (strict)"() -> ("Value"=w274:T7)  [unwired: 2 in, 2 out]
                n361 = call "subDAQ_GetSnapPoint.vi"("Record Table Refnum"=w266, "Snap Number Refnum"=w269, "Snap Point Y Arr Refnum"=w267, "Snap Point X Arr Refnum"=w268, "Snap Number Counting"="Snap Number Counting", "Stage Status"=w274) -> ("Snap Point cluster"=→"Snap Point cluster":cluster{"Snap Y":dbl[], "Snap X":dbl[]}, "Snap Point  Y Array"=→"Snap Point  Y Array":dbl[], "Snap Point  X Array"=→"Snap Point  X Array":dbl[])  [unwired: 3 in]
              }
              frame True {
              }
            }
            n362 = call "subDAQ_SetLaserDO.vi"("DAQ ports"=w234, "Light control (All off)"=w253, "Error in (no error)"=w242) -> ()  [unwired: 8 in, 1 out]
            n363 = property on="Live" class="Bool (strict)"() -> ("Value"=w250:bool)  [unwired: 2 in, 2 out]
            n364 = call "subHamamatsu_TurnOnOff.vi"("logic 2"=TRUE, "logic 1"=w250, "error in (no error)"=w251, "Handle in"=w255) -> ("error out"=w258:errorcluster, "Buffer"=w240:T22)  [unwired: 5 in, 1 out]
          }
          event "Camera Ctrl.ROI update": Value Change {
            n365 = event-data() -> ()  [unwired: 1 in, 1 out]
            n366 = property on="Handle" class="DigNum (strict)"() -> ("Value"=w300:u32)  [unwired: 2 in, 2 out]
            n367 = property on="Live" class="Bool (strict)"() -> ("Value"=w304:bool)  [unwired: 2 in, 2 out]
            n368 = call "subHamamatsu_TurnOnOff.vi"("logic 2"=FALSE ("Status post"), "logic 1"=w304, "error in (no error)"=w308, "Handle in"=w300) -> ("error out"=w305:errorcluster, "Handle out"=w306:u32)  [unwired: 5 in, 1 out]
            n369 = property on="ROI define" class="Bool (strict)"() -> ("Value"=w299:bool)  [unwired: 2 in, 2 out]
            n370 = property on="ROI cursor" class="Clust (strict)"() -> ("Value"=w301:T3)  [unwired: 2 in, 2 out]
            n371 = property on="ROI" class="Clust (strict)"() -> ("Value"=w296:T3)  [unwired: 2 in, 2 out]
            n372 = property on="ROI selection" class="Ring (strict)"() -> ("Value"=w298:u16)  [unwired: 2 in, 2 out]
            n373 = call "subHamamatsu_DefineROI.vi"("ROI selection"=w298, "ROI define"=w299, "ROI cursor"=w301) -> ("ROI out"=w297:T3)  [unwired: 8 in]
            n374 = call "subCalculate_SwitchROI.vi"("ROI 2 in"=w296, "ROI 1 in"=w297) -> ("ROI 2 out"=w294:T3, "ROI 1 out"=w295:T3)  [unwired: 8 in]
            n375 = call "subHamamatsu_SetROI.vi"("ROI"=w294, "error in (no error)"=w305, "Handle in"=w306) -> ("error out"=w284:errorcluster, "Handle out"=w285:u32)  [unwired: 6 in, 1 out]
            n376 = control-ref of="Camera View indicator"() -> (w291:refnum<vi>)
            n377 = control-ref of="Image"() -> (w292:refnum<vi>)
            n378 = property on="Previous ROI" class="Clust (strict)"("Value"=w295) -> ()  [unwired: 2 in, 2 out]
            n379 = call "subImage_UpdateLocIndicator.vi"("Camera View Indicator Ref"=w291, "Image Refnum"=w292, "ROI"=w294, "error in"=w284, "Handle in"=w285) -> ("error out"=w282:errorcluster, "Handle out"=w283:u32)  [unwired: 5 in]
            n380 = control-ref of="Pixel size (nm)"() -> (w289:refnum<vi>)
            n381 = control-ref of="Total y width (μm)"() -> (w288:refnum<vi>)
            n382 = control-ref of="scale bar (μm)"() -> (w290:refnum<vi>)
            n383 = control-ref of="Total x width (μm)"() -> (w287:refnum<vi>)
            n384 = local read "TI-Ctrl"() -> (w293:T9)
            n385 = Bundle("Total x width (μm)"=w287, "Total y width (μm)"=w288, "Pixel size (nm)"=w289, "scale bar (μm)"=w290) -> (w286:T28)  [unwired: 1 in]
            n386 = call "subCalculate_SetScaleBar.vi"("ROI in"=w294, "Scale calculation cluster"=w286, "TI-Ctrl"=w293, "error in"=w282, "Handle in"=w283) -> ("error out"=w280:errorcluster, "Handle out"=w281:u32)  [unwired: 5 in]
            n387 = call "subHamamatsu_GetMaxFrameRate.vi"("ROI in"=w294, "error in"=w280, "Handle in"=w281) -> ("error out"=w278:errorcluster, "Handle out"=w279:u32, "max frame rate (Hz)"=w303:dbl)  [unwired: 6 in]
            n388 = property on="max frame rate (Hz)" class="DigNum (strict)"("Value"=w303) -> ()  [unwired: 2 in, 2 out]
            n389 = property on="ROI" class="Clust (strict)"("Value"=w294) -> ()  [unwired: 2 in, 2 out]
            n390 = flat-sequence {
              tunnel: w279 -> [w318]
              tunnel: w278 -> [w317]
              tunnel: [w316] -> w302
              tunnel: [w314] -> w307
              frame #0 {
                w311 = FALSE ("Visible")
                n391 = property on="Live" class="Bool (strict)"() -> ("Value"=w310:bool)  [unwired: 2 in, 2 out]
                n392 = property on="ROI update" class="Bool (strict)"("Value"=w311) -> ()  [unwired: 2 in, 2 out]
                n393 = property on="ROI define" class="Bool (strict)"("Value"=w311) -> ()  [unwired: 2 in, 2 out]
                n394 = call "subHamamatsu_TurnOnOff.vi"("logic 2"=TRUE, "logic 1"=w310, "error in (no error)"=w317, "Handle in"=w318) -> ("error out"=w314:errorcluster, "Buffer"=w316:T22)  [unwired: 5 in, 1 out]
                n395 = property on="Image" class="IntGraph (strict)"("Active Cursor"=u32 0, "Cursor.Visible"=w311) -> ()  [unwired: 2 in, 2 out]
                n396 = property on="Image" class="IntGraph (strict)"("Active Cursor"=u32 1, "Cursor.Visible"=w311) -> ()  [unwired: 2 in, 2 out]
              }
            }
          }
          event "Camera Ctrl.ROI previous": Value Change {
            w347 = FALSE ("Update ROI")
            n397 = event-data() -> ()  [unwired: 1 in, 1 out]
            n398 = property on="Handle" class="DigNum (strict)"() -> ("Value"=w342:u32)  [unwired: 2 in, 2 out]
            n399 = property on="ROI previous" class="Bool (strict)"("Value"=w347) -> ()  [unwired: 2 in, 2 out]
            n400 = property on="ROI define" class="Bool (strict)"("Value"=w347) -> ()  [unwired: 2 in, 2 out]
            n401 = property on="Image" class="IntGraph (strict)"("Active Cursor"=u32 0, "Cursor.Visible"=w347) -> ()  [unwired: 2 in, 2 out]
            n402 = property on="Image" class="IntGraph (strict)"("Active Cursor"=u32 1, "Cursor.Visible"=w347) -> ()  [unwired: 2 in, 2 out]
            n403 = property on="Live" class="Bool (strict)"() -> ("Value"=w345:bool)  [unwired: 2 in, 2 out]
            n404 = call "subHamamatsu_TurnOnOff.vi"("logic 2"=FALSE, "logic 1"=w345, "error in (no error)"=w351, "Handle in"=w342) -> ("error out"=w336:errorcluster, "Handle out"=w335:u32)  [unwired: 5 in, 1 out]
            n405 = local read "Previous ROI"() -> (w340:T3)
            n406 = property on="ROI" class="Clust (strict)"() -> ("Value"=w341:T3)  [unwired: 2 in, 2 out]
            n407 = call "subCalculate_SwitchROI.vi"("ROI 2 in"=w341, "ROI 1 in"=w340) -> ("ROI 2 out"=w334:T3, "ROI 1 out"=w339:T3)  [unwired: 8 in]
            n408 = call "subHamamatsu_SetROI.vi"("ROI"=w334, "error in (no error)"=w336, "Handle in"=w335) -> ("error out"=w326:errorcluster, "Handle out"=w322:u32)  [unwired: 6 in, 1 out]
            n409 = control-ref of="Camera View indicator"() -> (w333:refnum<vi>)
            n410 = control-ref of="Image"() -> (w332:refnum<vi>)
            n411 = property on="Previous ROI" class="Clust (strict)"("Value"=w339) -> ()  [unwired: 2 in, 2 out]
            n412 = call "subImage_UpdateLocIndicator.vi"("Camera View Indicator Ref"=w333, "Image Refnum"=w332, "ROI"=w334, "error in"=w326, "Handle in"=w322) -> ("error out"=w325:errorcluster, "Handle out"=w321:u32)  [unwired: 5 in]
            n413 = control-ref of="Pixel size (nm)"() -> (w327:refnum<vi>)
            n414 = control-ref of="Total x width (μm)"() -> (w329:refnum<vi>)
            n415 = control-ref of="Total y width (μm)"() -> (w330:refnum<vi>)
            n416 = control-ref of="scale bar (μm)"() -> (w331:refnum<vi>)
            n417 = local read "TI-Ctrl"() -> (w337:T9)
            n418 = Bundle("Total x width (μm)"=w329, "Total y width (μm)"=w330, "Pixel size (nm)"=w327, "scale bar (μm)"=w331) -> (w328:T28)  [unwired: 1 in]
            n419 = call "subCalculate_SetScaleBar.vi"("ROI in"=w334, "Scale calculation cluster"=w328, "TI-Ctrl"=w337, "error in"=w325, "Handle in"=w321) -> ("error out"=w324:errorcluster, "Handle out"=w320:u32)  [unwired: 5 in]
            n420 = call "subHamamatsu_GetMaxFrameRate.vi"("ROI in"=w334, "error in"=w324, "Handle in"=w320) -> ("error out"=w323:errorcluster, "Handle out"=w319:u32, "max frame rate (Hz)"=w338:dbl)  [unwired: 6 in]
            n421 = property on="max frame rate (Hz)" class="DigNum (strict)"("Value"=w338) -> ()  [unwired: 2 in, 2 out]
            n422 = property on="ROI" class="Clust (strict)"("Value"=w334) -> ()  [unwired: 2 in, 2 out]
            n423 = property on="Live" class="Bool (strict)"() -> ("Value"=w346:bool)  [unwired: 2 in, 2 out]
            n424 = call "subHamamatsu_TurnOnOff.vi"("logic 2"=TRUE, "logic 1"=w346, "error in (no error)"=w323, "Handle in"=w319) -> ("error out"=w350:errorcluster, "Buffer"=w344:T22)  [unwired: 5 in, 1 out]
          }
          event "Camera Ctrl.ROI.Bin": Value Change {
            # "Recalculate ROI"
            n425 = event-data() -> ("OldVal"=w384:u16, "NewVal"=w379:u16)  [unwired: 1 in]
            n426 = property on="Handle" class="DigNum (strict)"() -> ("Value"=w375:u32)  [unwired: 2 in, 2 out]
            n427 = control-ref of="Image"() -> (w373:refnum<vi>)
            n428 = property on="ROI" class="Clust (strict)"() -> ("Value"=w374:T3)  [unwired: 2 in, 2 out]
            n429 = property on="Live" class="Bool (strict)"() -> ("Value"=w378:bool)  [unwired: 2 in, 2 out]
            n430 = call "subHamamatsu_TurnOnOff.vi"("logic 2"=FALSE ("Status post"), "logic 1"=w378, "error in (no error)"=w381, "Handle in"=w375) -> ("error out"=w361:errorcluster, "Handle out"=w363:u32)  [unwired: 5 in, 1 out]
            n431 = call "subImage_UpdateBin.vi"("Bin (n x n)"=w379, "Previous bin"=w384, "Image Refnum"=w373, "ROI in"=w374) -> ("ROI out"=w362:T3)  [unwired: 7 in]
            n432 = call "subHamamatsu_SetBin.vi"("ROI"=w362, "error in (no error)"=w361, "Handle in"=w363) -> ("error out"=w360:errorcluster, "Handle out"=w355:u32)  [unwired: 7 in]
            n433 = control-ref of="Camera View indicator"() -> (w369:refnum<vi>)
            n434 = control-ref of="Image"() -> (w370:refnum<vi>)
            n435 = call "subImage_UpdateLocIndicator.vi"("Camera View Indicator Ref"=w369, "Image Refnum"=w370, "ROI"=w362, "error in"=w360, "Handle in"=w355) -> ("error out"=w359:errorcluster, "Handle out"=w354:u32)  [unwired: 5 in]
            n436 = control-ref of="Total x width (μm)"() -> (w366:refnum<vi>)
            n437 = control-ref of="Total y width (μm)"() -> (w367:refnum<vi>)
            n438 = control-ref of="scale bar (μm)"() -> (w365:refnum<vi>)
            n439 = control-ref of="Pixel size (nm)"() -> (w368:refnum<vi>)
            n440 = local read "TI-Ctrl"() -> (w371:T9)
            n441 = Bundle("Total x width (μm)"=w366, "Total y width (μm)"=w367, "Pixel size (nm)"=w368, "scale bar (μm)"=w365) -> (w364:T28)  [unwired: 1 in]
            n442 = call "subCalculate_SetScaleBar.vi"("ROI in"=w362, "Scale calculation cluster"=w364, "TI-Ctrl"=w371, "error in"=w359, "Handle in"=w354) -> ("error out"=w358:errorcluster, "Handle out"=w353:u32)  [unwired: 5 in]
            n443 = call "subHamamatsu_GetMaxFrameRate.vi"("ROI in"=w362, "error in"=w358, "Handle in"=w353) -> ("error out"=w357:errorcluster, "Handle out"=w356:u32, "max frame rate (Hz)"=w372:dbl)  [unwired: 6 in]
            n444 = property on="max frame rate (Hz)" class="DigNum (strict)"("Value"=w372) -> ()  [unwired: 2 in, 2 out]
            n445 = property on="ROI" class="Clust (strict)"("Value"=w362) -> ()  [unwired: 2 in, 2 out]
            n446 = property on="Live" class="Bool (strict)"() -> ("Value"=w377:bool)  [unwired: 2 in, 2 out]
            n447 = call "subHamamatsu_TurnOnOff.vi"("logic 2"=TRUE ("Status post"), "logic 1"=w377, "error in (no error)"=w357, "Handle in"=w356) -> ("error out"=w380:errorcluster, "Buffer"=w376:T22)  [unwired: 5 in, 1 out]
          }
          event "Camera Ctrl.Exposure (ms)": Value Change {
            n448 = event-data() -> ()  [unwired: 1 in, 1 out]
            n449 = property on="Handle" class="DigNum (strict)"() -> ("Value"=w385:u32)  [unwired: 2 in, 2 out]
            n450 = property on="Exposure (ms)" class="DigNum (strict)"() -> ("Value"=w388:dbl)  [unwired: 2 in, 2 out]
            n451 = call "subHamamatsu_SetExposure.vi"("Exposure (ms)"=w388, "error in (no error)"=w387, "Handle in"=w385) -> ("error out"=w389:errorcluster)  [unwired: 7 in, 1 out]
          }
          event "Run waveform": Value Change {
            n452 = event-data() -> ()  [unwired: 1 in, 1 out]
            n453 = flat-sequence {
              tunnel: [w419] -> w403
              tunnel: w402 -> [w424]
              tunnel: [w437] -> w400
              tunnel: [w450] -> w399
              tunnel: w403 -> [w445]
              tunnel: [w446] -> w401
              tunnel: w400 -> [w444]
              frame #0 {
                # "save TXT file"
                # "If camera is running, turn it off."
                # "Create full folder name with current time"
                n454 = property on="Lasers AO (V)" class="Arr (strict)"(error in=w424) -> (error out=w423:errorcluster, "Value"=w422:dbl[])  [unwired: 1 in, 1 out]
                n455 = property on="Previous Lasers AO (V)" class="Arr (strict)"("Value"=w422) -> ()  [unwired: 2 in, 2 out]
                n456 = property on="Handle" class="DigNum (strict)"() -> ("Value"=w429:u32)  [unwired: 2 in, 2 out]
                n457 = property on="Live" class="Bool (strict)"() -> ("Value"=w432:bool)  [unwired: 2 in, 2 out]
                n458 = call "subHamamatsu_TurnOnOff.vi"("logic 2"=FALSE, "logic 1"=w432, "error in (no error)"=w423, "Handle in"=w429) -> ("error out"=w436:errorcluster, "Handle out"=w431:u32)  [unwired: 5 in, 1 out]
                n459 = property on="Status" class="Str"("Value"="Acquiring .dcimg file" ("Status")) -> ()  [unwired: 2 in, 2 out]
                n460 = property on="DAQ ports" class="Clust (strict)"() -> ("Value"=w427:T25)  [unwired: 2 in, 2 out]
                n461 = call "subDAQ_WaveformPorts.vi"("DAQ ports"=w427, "Waveform channels"="Waveform channels") -> ("Waveform port selection"=w439:T33)  [unwired: 9 in]
                n462 = call "subSave_CreateSubfolder.vi"("Time (F)"=TRUE, "Subfolder name"="Sub-folder", "Base path"="Base folder") -> ("Subfolder"=w405:path)  [unwired: 8 in]
                "Full path" <- w405
                n463 = call "subAcquisition_Waveform.vi"("Waveform info"="Waveform info", "full path"=w405, "error in (no error)"=w436, "Waveform port selection"=w439, "Handle in"=w431) -> ("Error out"=w434:errorcluster, "Acquisition params"=w416:T34, "Handle out"=w437:u32, "AI Waveform"=→"AI Waveform":cluster{"xo":i32, dbl, "data":dbl[][]})  [unwired: 3 in]
                n464 = local read "Stage Status"() -> (w413:T7)
                n465 = local read "Camera Info"() -> (w411:T19)
                n466 = local read "Light control"() -> (w414:T1)
                n467 = local read "Confocal scanner"() -> (w409:T5)
                n468 = local read "Image Info"() -> (w415:T2)
                n469 = local read "Camera Ctrl"() -> (w412:T8)
                n470 = local read "TI-Ctrl"() -> (w410:T9)
                n471 = call "subAcquisition_MovieInfo.vi"("Stage Status"=w413, "Acquisition params"=w416, "Light control"=w414, "Image Info"=w415, "Confocal scanner"=w409, "TI-Ctrl"=w410, "Camera Info"=w411, "Camera Ctrl"=w412) -> ("Text"=w404:string)  [unwired: 3 in]
                n472 = property on="Previous Light control" class="Clust (strict)"() -> ("Value"=w421:T1)  [unwired: 2 in, 2 out]
                n473 = property on="DAQ ports" class="Clust (strict)"() -> ("Value"=w425:T25)  [unwired: 2 in, 2 out]
                n474 = call "subDAQ_SetLaserDO.vi"("DAQ ports"=w425, "Error in (no error)"=w434) -> ("Error out"=w426:errorcluster)  [unwired: 9 in]
                n475 = Build Path(base path=w405, name or relative path="movie_info.txt") -> (appended path=w406:path)
                n476 = call "subDAQ_SetLaserAO.vi"("DAQ ports"=w425, "Light control (All off)"=w421, "Error in (no error)"=w426) -> ("Error out"=w420:errorcluster)  [unwired: 8 in]
                n477 = property on="Lasers DO" class="Arr (strict)"(error in=w420, "Value"=bool[] [FALSE, FALSE, FALSE, FALSE, FALSE, FALSE]) -> (error out=w419:errorcluster)  [unwired: 1 in, 1 out]
                n478 = Write to Text File(file (use dialog)=w406, text=w404) -> ()  [unwired: 2 in, 3 out]
              }
              frame #1 {
                # "Reset camera settings"
                n479 = property on="Exposure (ms)" class="DigNum (strict)"() -> ("Value"=w441:dbl)  [unwired: 2 in, 2 out]
                n480 = local write "Run waveform"(FALSE) -> ()
                n481 = call "subHamamatsu_SetExposure.vi"("Exposure (ms)"=w441, "error in (no error)"=w445, "Handle in"=w444) -> ("error out"=w447:errorcluster, "Handle out"=w449:u32)  [unwired: 7 in]
                n482 = property on="Status" class="Str"("Value"="ready" ("Status")) -> ()  [unwired: 2 in, 2 out]
                n483 = property on="Live" class="Bool (strict)"() -> ("Value"=w442:bool)  [unwired: 2 in, 2 out]
                n484 = call "subHamamatsu_TurnOnOff.vi"("logic 2"=TRUE, "logic 1"=w442, "error in (no error)"=w447, "Handle in"=w449) -> ("error out"=w446:errorcluster, "Buffer"=w450:T22)  [unwired: 5 in, 1 out]
              }
            }
            n485 = control-ref of="Snap Number Counting"() -> (w394:refnum<vi>)
            n486 = control-ref of="Movie Point  Y Array"() -> (w391:refnum<vi>)
            n487 = control-ref of="Movie Point  X Array"() -> (w392:refnum<vi>)
            n488 = property on="Snap Number Counting" class="DigNum (strict)"() -> ("Value"=w393:dbl)  [unwired: 2 in, 2 out]
            n489 = control-ref of="Record Table"() -> (w390:refnum<vi>)
            n490 = property on="Stage Status" class="Clust (strict)"() -> ("Value"=w398:T7)  [unwired: 2 in, 2 out]
            n491 = call "subDAQ_GetMoviePoint.vi"("Recorde Table Refnum"=w390, "Snap Number Refnum"=w394, "Movie Point Y Arr Refnum"=w391, "Movie Point X Arr Refnum"=w392, "Snap Number Counting"=w393, "Stage Status"=w398) -> ("Snap/Movie Point cluster"=→"Movie Point cluster":cluster{"Snap Y":dbl[], "Snap X":dbl[]}, "Movie Point  Y Array"=→"Movie Point  Y Array":dbl[], "Movie Point  X Array"=→"Movie Point  X Array":dbl[])  [unwired: 3 in]
          }
          event "Stream movie": Value Change {
            n492 = event-data() -> ()  [unwired: 1 in, 1 out]
            n493 = flat-sequence {
              tunnel: w468 -> [w477]
              tunnel: [w485] -> w467
              tunnel: [w479] -> w466
              tunnel: [w478] -> w465
              tunnel: w467 -> [w505]
              tunnel: w466 -> [w495]
              tunnel: w465 -> [w501]
              tunnel: [w500] -> w464
              tunnel: [w499] -> w462
              tunnel: [w508] -> w463
              tunnel: w464 -> [w508]
              tunnel: w462 -> [w507]
              tunnel: [w507] -> w461
              frame #0 {
                n494 = property on="Handle" class="DigNum (strict)"() -> ("Value"=w470:u32)  [unwired: 2 in, 2 out]
                n495 = local read "Sub-folder"() -> (w473:string)
                n496 = local read "Base folder"() -> (w474:path)
                n497 = property on="Live" class="Bool (strict)"() -> ("Value"=w471:bool)  [unwired: 2 in, 2 out]
                n498 = call "subHamamatsu_TurnOnOff.vi"("logic 2"=FALSE, "logic 1"=w471, "error in (no error)"=w477, "Handle in"=w470) -> ("error out"=w484:errorcluster, "Handle out"=w469:u32)  [unwired: 5 in, 1 out]
                n499 = call "subSave_CreateSubfolder.vi"("Subfolder name"=w473, "Base path"=w474) -> ("Subfolder"=w475:path)  [unwired: 9 in]
                n500 = local read "Movie frame rate (Hz)"() -> (w480:dbl)
                n501 = property on="Status" class="Str"("Value"="Stream movie" ("Status")) -> ()  [unwired: 2 in, 2 out]
                n502 = Build Path(base path=w475, name or relative path="movie.dcimg" ("string")) -> (appended path=w485:path)
                n503 = local read "# frames"() -> (w483:i32)
                n504 = control-ref of="Frames Recorded"() -> (w481:refnum<vi>)
                n505 = control-ref of="Elapsed time (sec)"() -> (w482:refnum<vi>)
                n506 = call "subAcquisition_StreamMovie.vi"("Elapsed time (sec) Refnum"=w482, "Frames Recorded Refnum"=w481, "File path"=w485, "error in (no error)"=w484, "Movie frame rate (Hz)"=w480, "# frames"=w483, "Handle in"=w469) -> ("error out"=w478:errorcluster, "Handle out"=w479:u32)  [unwired: 3 in]
              }
              frame #1 {
                n507 = local read "Camera Ctrl"() -> (w488:T8)
                n508 = local read "Camera Info"() -> (w487:T19)
                n509 = local read "Image Info"() -> (w489:T2)
                n510 = local read "TI-Ctrl"() -> (w494:T9)
                n511 = local read "Confocal scanner"() -> (w493:T5)
                n512 = property on="Exposure (ms)" class="DigNum (strict)"() -> ("Value"=w498:dbl)  [unwired: 2 in, 2 out]
                n513 = local read "Light control"() -> (w492:T1)
                n514 = local read "Stage Status"() -> (w491:T7)
                n515 = call "subHamamatsu_SetExposure.vi"("Exposure (ms)"=w498, "error in (no error)"=w501, "Handle in"=w495) -> ("error out"=w504:errorcluster, "Handle out"=w503:u32)  [unwired: 7 in]
                n516 = call "subAcquisition_Info.vi"("Stage Status"=w491, "Light control"=w492, "Image Info"=w489, "Confocal scanner"=w493, "TI-Ctrl"=w494, "Camera Info"=w487, "Camera Ctrl"=w488) -> ("Text"=w490:string)  [unwired: 4 in]
                n517 = property on="Live" class="Bool (strict)"() -> ("Value"=w497:bool)  [unwired: 2 in, 2 out]
                n518 = property on="Status" class="Str"("Value"="Saving binary file" ("Status")) -> ()  [unwired: 2 in, 2 out]
                n519 = call "subSave_Dcimg2Bin.vi"("Text"=w490, ".dcimg file name"=w505) -> ()  [unwired: 9 in, 1 out]
                n520 = call "subHamamatsu_TurnOnOff.vi"("logic 2"=TRUE, "logic 1"=w497, "error in (no error)"=w504, "Handle in"=w503) -> ("error out"=w500:errorcluster, "Buffer"=w499:T22)  [unwired: 5 in, 1 out]
              }
              frame #2 {
                n521 = local write "Stream movie"(FALSE ("Acquire movie")) -> ()
                n522 = property on="Status" class="Str"("Value"="ready" ("Status")) -> ()  [unwired: 2 in, 2 out]
              }
            }
            n523 = control-ref of="Snap Number Counting"() -> (w456:refnum<vi>)
            n524 = control-ref of="Movie Point  Y Array"() -> (w459:refnum<vi>)
            n525 = control-ref of="Movie Point  X Array"() -> (w458:refnum<vi>)
            n526 = property on="Snap Number Counting" class="DigNum (strict)"() -> ("Value"=w457:dbl)  [unwired: 2 in, 2 out]
            n527 = control-ref of="Record Table"() -> (w460:refnum<vi>)
            n528 = property on="Stage Status" class="Clust (strict)"() -> ("Value"=w455:T7)  [unwired: 2 in, 2 out]
            n529 = call "subDAQ_GetMoviePoint.vi"("Recorde Table Refnum"=w460, "Snap Number Refnum"=w456, "Movie Point Y Arr Refnum"=w459, "Movie Point X Arr Refnum"=w458, "Snap Number Counting"=w457, "Stage Status"=w455) -> ("Snap/Movie Point cluster"=w452:cluster{"Snap Y":dbl[], "Snap X":dbl[]}, "Movie Point  Y Array"=w453:dbl[], "Movie Point  X Array"=w454:dbl[])  [unwired: 3 in]
            n530 = local write "Movie Point  X Array"(w454) -> ()
            n531 = local write "Movie Point  Y Array"(w453) -> ()
            n532 = local write "Movie Point cluster"(w452) -> ()
          }
          event "MD acquisition": Value Change {
            # "Timelapse Loop"
            # "Multidimensional acquisition"
            n533 = event-data() -> ()  [unwired: 1 in, 1 out]
            n534 = property on="Handle" class="DigNum (strict)"() -> ("Value"=w513:u32)  [unwired: 2 in, 2 out]
            n535 = property on="Live" class="Bool (strict)"() -> ("Value"=w514:bool)  [unwired: 2 in, 2 out]
            n536 = local read "Timelapse?"() -> (w512:bool)
            n537 = call "subHamamatsu_TurnOnOff.vi"("logic 2"=FALSE, "logic 1"=w514, "error in (no error)"=w526, "Handle in"=w513) -> ("error out"=w522:errorcluster)  [unwired: 5 in, 2 out]
            n538 = case shown="True" w512 {
              tunnel: [1 ("Timelapse Cycles") "Timelapse Cycles"] -> w511
              tunnel: [u32 0 "Period (s)"] -> w510
              frame False {
              }
              frame True {
                n539 = property on="T Acquired Progress" class="Slide (strict)"("Scale.Maximum"="Timelapse Cycles") -> ()  [unwired: 2 in, 2 out]
              }
            }
            n540 = local read "Base folder"() -> (w516:path)
            n541 = local read "Sub-folder"() -> (w518:string)
            n542 = call "subSave_CreateSubfolder.vi"("Time (F)"=TRUE, "Subfolder name"=w518, "Base path"=w516) -> ("Subfolder"=w515:path)  [unwired: 8 in]
            n543 = Tick Count (ms)() -> (millisecond timer value=w520:u32)
            n544 = for {
              N: w511 -> [_]
              tunnel: w520 -> [w567]
              tunnel: w510 -> [w545]
              shift-right: [w536] -> w521
              shift-left: w522 -> [w559]
              tunnel: "Channel settings" -> [w548]
              tunnel: w515 -> [w543]
              i -> [w566]
              # "Cycle through Colors"
              # "Wait for next time point"
              n545 = Tick Count (ms)() -> (millisecond timer value=w569:u32)
              n546 = Subtract(x=w569, y=w567) -> (x-y=w570:u32)
              n547 = local read "Timelapse Cycles"() -> (w546:i32)
              n548 = Increment(x=w566) -> (x+1=w547:i32)
              n549 = Divide(x=w570, y=1000.0) -> (x/y=w537:dbl)
              n550 = Unbundle By Name(w548) -> ("Name"=w562:string[], "Take?"=w563:bool[], "Cumulation"=w550:i32[], "Exposure time (msec)"=w551:dbl[])
              n551 = Multiply(x=u32 1000 ("y"), y=w545) -> (x*y=w549:u32)
              n552 = local read "TiE Ref"() -> (w556:T21)
              n553 = control-ref of="TI-Ctrl"() -> (w555:refnum<vi>)
              n554 = control-ref of="Light control"() -> (w553:refnum<vi>)
              n555 = control-ref of="Confocal scanner"() -> (w552:refnum<vi>)
              n556 = property on="DAQ ports" class="Clust (strict)"() -> ("Value"=w542:T25)  [unwired: 2 in, 2 out]
              n557 = property on="Confocal VISA Setting" class="VISAName"() -> ("Value"=w540:refnum<visa-resource-name>)  [unwired: 2 in, 2 out]
              n558 = property on="Channel" class="Arr (strict)"() -> ("Value"=w558:i32[])  [unwired: 2 in, 2 out]
              n559 = property on="Timelapse Time (s)" class="DigNum (strict)"("Value"=w537) -> ()  [unwired: 2 in, 2 out]
              n560 = property on="Take?" class="Arr (strict)"() -> ("Value"=w557:bool[])  [unwired: 2 in, 2 out]
              n561 = To Long Integer(number=w558) -> (32bit integer=w564:i32[])
              n562 = Bundle("TI-Ctrl"=w555, "TiE Ref"=w556) -> (w554:T35)  [unwired: 1 in]
              n563 = Array Size(array=w557) -> (size(s)=w561:i32)
              n564 = Greater?(x=w546, y=w547) -> (0:w565:bool)
              n565 = for {
                N: w561 -> [_]
                tunnel: w563 -> [w581] mode=indexing
                tunnel: w564 -> [w579] mode=indexing
                shift-right: [w583] -> w560
                shift-left: w559 -> [w584]
                tunnel: w543 -> [w582]
                tunnel: w562 -> [w580] mode=indexing
                tunnel: w554 -> [w578]
                tunnel: w551 -> [w577] mode=indexing
                tunnel: w553 -> [w576]
                tunnel: w552 -> [w575]
                tunnel: w542 -> [w574]
                tunnel: w550 -> [w573] mode=indexing
                tunnel: w547 -> [w572]
                tunnel: w540 -> [w571]
                n566 = case shown="True" w581 {
                  tunnel: w584 -> [w585 w588]
                  tunnel: [w585 w613] -> w583
                  tunnel: w582 -> [_ w616]
                  tunnel: w580 -> [_ w598]
                  tunnel: w579 -> [_ w589]
                  tunnel: w578 -> [_ w611]
                  tunnel: w577 -> [_ w594]
                  tunnel: w576 -> [_ w610]
                  tunnel: w575 -> [_ w609]
                  tunnel: w574 -> [_ w608]
                  tunnel: w573 -> [_ w599]
                  tunnel: w572 -> [_ w590]
                  tunnel: w571 -> [_ w591]
                  frame False {
                  }
                  frame True {
                    # "Filter Set cluster"
                    # "stage cluster"
                    # "zstack cluster"
                    n567 = control-ref of="Color Acquiring"() -> (w587:refnum<vi>)
                    n568 = Bundle("Filter Set"=w589, "Light control"=w610, "Confocal scanner"=w609, "Value"=w608, "Value"=w591) -> (w592:T36)  [unwired: 1 in]
                    n569 = call "subAcquisition_AcquirngColor.vi"("Bool Refnum"=w587, "Filter Set"=w589) -> ()  [unwired: 10 in]
                    n570 = Build Path(base path=w616, name or relative path=w598) -> (appended path=w603:path)
                    n571 = call "subDAQ_SetFilterSet.vi"("Ti-E cluster"=w611, "Filterset cluster"=w592, "error in"=w588) -> ("error out"=w615:errorcluster)  [unwired: 8 in]
                    n572 = property on="Handle" class="DigNum (strict)"() -> ("Value"=w593:u32)  [unwired: 2 in, 2 out]
                    n573 = local read "Timelapse?"() -> (w596:bool)
                    n574 = call "subHamamatsu_SetExposure.vi"("Exposure (ms)"=w594, "error in (no error)"=w615, "Handle in"=w593) -> ("error out"=w614:errorcluster, "Handle out"=w612:u32)  [unwired: 7 in]
                    n575 = Select(t=w590, s=w596, f=0) -> (s? t:f=w595:i32)
                    n576 = local read "Z-Stack"() -> (w607:T10)
                    n577 = control-ref of="Image Info"() -> (w605:refnum<vi>)
                    n578 = local read "Camera Ctrl"() -> (w606:T8)
                    n579 = local read "XY tiling"() -> (w602:T12)
                    n580 = control-ref of="Stage Status"() -> (w601:refnum<vi>)
                    n581 = control-ref of="Z Stack Aquired"() -> (w586:refnum<vi>)
                    n582 = Bundle("XY tiling"=w602, "Stage Status"=w601) -> (w600:T37)  [unwired: 1 in]
                    n583 = Bundle(w595, "appended path"=w603, "Z-Stack"=w607, "Arch_Dragon cumulation"=w599, "Image Info"=w605, "Camera Ctrl"=w606) -> (w604:T38)  [unwired: 1 in]
                    n584 = call "subAcquisition_3D.vi"("Z-stack cluster in"=w604, "Ti-E cluster"=w611, "Stage cluster"=w600, "error in"=w614, "Z Stack Aquired Refnum"=w586, "Handle in"=w612) -> ("error out"=w613:errorcluster)  [unwired: 5 in]
                    "Timelapse Acquired" <- w590
                    "T Acquired Progress" <- w590
                  }
                }
              }
              n585 = case shown="True" w565 {
                tunnel: w549 -> [_ w618]
                frame False {
                }
                frame True {
                  n586 = Wait Until Next ms Multiple(millisecond multiple=w618) -> (millisecond timer value=→"millisecond timer value":u32)
                }
              }
              n587 = property on="DAQ ports" class="Clust (strict)"() -> ("Value"=w541:T25)  [unwired: 2 in, 2 out]
              n588 = call "subDAQ_SetLaserDO.vi"("DAQ ports"=w541, "Error in (no error)"=w560) -> ("Error out"=w539:errorcluster)  [unwired: 9 in]
              n589 = property on="Lasers DO" class="Arr (strict)"(error in=w539, "Value"=bool[] [FALSE, FALSE, FALSE, FALSE, FALSE, FALSE]) -> (error out=w535:errorcluster)  [unwired: 1 in, 1 out]
              n590 = Bundle(u32 1985280, u32 16448250) -> (w533:cluster{u32, u32})  [unwired: 1 in]
              n591 = Build Array(w533) -> (w531:cluster{u32, u32}[])
              n592 = property on="Color Acquiring" class="Bool (strict)"(error in=w535, "Colors [4]"=w531) -> (error out=w536:errorcluster)  [unwired: 1 in, 1 out]
            }
            n593 = flat-sequence {
              tunnel: w521 -> [w623]
              tunnel: [w627] -> w525
              tunnel: [w626] -> w524
              frame #0 {
                n594 = property on="Handle" class="DigNum (strict)"() -> ("Value"=w619:u32)  [unwired: 2 in, 2 out]
                n595 = property on="Exposure (ms)" class="DigNum (strict)"() -> ("Value"=w621:dbl)  [unwired: 2 in, 2 out]
                n596 = call "subHamamatsu_SetExposure.vi"("Exposure (ms)"=w621, "error in (no error)"=w623, "Handle in"=w619) -> ("error out"=w625:errorcluster, "Handle out"=w624:u32)  [unwired: 7 in]
                n597 = local write "MD acquisition"(FALSE ("Capture")) -> ()
                n598 = property on="Live" class="Bool (strict)"() -> ("Value"=w620:bool)  [unwired: 2 in, 2 out]
                n599 = call "subHamamatsu_TurnOnOff.vi"("logic 2"=TRUE, "logic 1"=w620, "error in (no error)"=w625, "Handle in"=w624) -> ("error out"=w627:errorcluster, "Buffer"=w626:T22)  [unwired: 5 in, 1 out]
              }
            }
          }
        }
      }
      "Camera" <- w36
      n600 = while {
        shift-right: [w1027] -> _
        shift-left: errorcluster {"status"=FALSE, "code"=0, "source"=""} ("Error out") -> [w1028]
        stop <- w1026 stop-if-true
        # "Light control"
        n601 = event shown="[5] \"Light control.Filter Set\": Value Change" {
          selector: _ -> [_ _ _ _ _ _]
          dyn-events: _ -> [_ _ _ _ _ _]
          timeout: 50 -> [_ _ _ _ _ _]
          tunnel: w1028 -> [w1030 w1033 w1038 w1042 w1045 w1057]
          tunnel: [w1030 w1034 w1037 w1041 w1046 w1056] -> w1027
          event Timeout {
            n602 = event-data() -> ()  [unwired: 1 in, 1 out]
          }
          event "Light control.Lasers AO (V)": Value Change {
            n603 = event-data() -> ()  [unwired: 1 in, 1 out]
            n604 = local read "Light control"() -> (w1032:T1)
            n605 = property on="DAQ ports" class="Clust (strict)"() -> ("Value"=w1031:T25)  [unwired: 2 in, 2 out]
            n606 = call "subDAQ_SetLaserAO.vi"("DAQ ports"=w1031, "Light control (All off)"=w1032, "Error in (no error)"=w1033) -> ("Error out"=w1034:errorcluster)  [unwired: 8 in]
          }
          event "Light control.Lasers DO": Value Change {
            n607 = event-data() -> ()  [unwired: 1 in, 1 out]
            n608 = local read "Light control"() -> (w1036:T1)
            n609 = property on="DAQ ports" class="Clust (strict)"() -> ("Value"=w1035:T25)  [unwired: 2 in, 2 out]
            n610 = call "subDAQ_SetLaserDO.vi"("DAQ ports"=w1035, "Light control (All off)"=w1036, "Error in (no error)"=w1038) -> ("Error out"=w1037:errorcluster)  [unwired: 8 in]
          }
          event "Light control.LED": Value Change {
            n611 = event-data() -> ()  [unwired: 1 in, 1 out]
            n612 = property on="DAQ ports" class="Clust (strict)"() -> ("Value"=w1039:T25)  [unwired: 2 in, 2 out]
            n613 = local read "Light control"() -> (w1040:T1)
            n614 = call "subDAQ_SetLED.vi"("DAQ ports"=w1039, "Light control (All Off)"=w1040, "Error in (no error)"=w1042) -> ("Error out"=w1041:errorcluster)  [unwired: 8 in]
          }
          event "Light control.Global": Value Change {
            n615 = event-data() -> ()  [unwired: 1 in, 1 out]
            n616 = local read "Light control"() -> (w1044:T1)
            n617 = property on="DAQ ports" class="Clust (strict)"() -> ("Value"=w1043:T25)  [unwired: 2 in, 2 out]
            n618 = call "subDAQ_SetGlobal.vi"("DAQ ports"=w1043, "Light control (All off)"=w1044, "Error in (no error)"=w1045) -> ("Error out"=w1046:errorcluster)  [unwired: 8 in]
          }
          event "Light control.Filter Set": Value Change {
            n619 = event-data() -> ("NewVal"=w1052:i32)  [unwired: 1 in]
            n620 = property on="DAQ ports" class="Clust (strict)"() -> ("Value"=w1048:T25)  [unwired: 2 in, 2 out]
            n621 = control-ref of="Light control"() -> (w1051:refnum<vi>)
            n622 = control-ref of="Confocal scanner"() -> (w1050:refnum<vi>)
            n623 = property on="Confocal VISA Setting" class="VISAName"() -> ("Value"=w1047:refnum<visa-resource-name>)  [unwired: 2 in, 2 out]
            n624 = local read "TiE Ref"() -> (w1054:T21)
            n625 = control-ref of="TI-Ctrl"() -> (w1055:refnum<vi>)
            n626 = Bundle("NewVal"=w1052, "Light control"=w1051, "Confocal scanner"=w1050, "Value"=w1048, "Value"=w1047) -> (w1049:T39)  [unwired: 1 in]
            n627 = Bundle("TI-Ctrl"=w1055, "TiE Ref"=w1054) -> (w1053:T35)  [unwired: 1 in]
            n628 = call "subDAQ_SetFilterSet.vi"("Ti-E cluster"=w1053, "Filterset cluster"=w1049, "error in"=w1057) -> ("error out"=w1056:errorcluster)  [unwired: 8 in]
          }
        }
        n629 = local read "stop program"() -> (w1026:bool)
      }
      n630 = while {
        stop <- w39 stop-if-true
        # "Waveforms"
        n631 = event shown="[1] \"Load waveform\": Value Change" {
          selector: _ -> [_ _]
          dyn-events: _ -> [_ _]
          timeout: 50 -> [_ _]
          event Timeout {
            n632 = event-data() -> ()  [unwired: 1 in, 1 out]
          }
          event "Load waveform": Value Change {
            n633 = event-data() -> ()  [unwired: 1 in, 1 out]
            n634 = local read "Waveform channels"() -> (w46:T13)
            n635 = property on="DAQ ports" class="Clust (strict)"() -> ("Value"=w41:T25)  [unwired: 2 in, 2 out]
            n636 = local read "Waveform info"() -> (w47:T14)
            n637 = call "subDAQ_WaveformPorts.vi"("DAQ ports"=w41, "Waveform channels"=w46) -> ("Waveform port selection"=w45:T33)  [unwired: 9 in]
            n638 = call "subDAQ_GenWaveform.vi"("Waveform port selection"=w45, "Waveform info"=w47) -> ("error out"=w43:errorcluster, "Dev1 AO waveform"=→"Patch Ex. Command AO waveform":waveform(dbl), "Lasers AO waveform"=→"Lasers AO waveform":waveform(dbl)[], "Lasers DO waveform"=→"Lasers DO waveform":digitalwaveform[])  [unwired: 5 in, 1 out]
            n639 = property on="Load waveform" class="Bool (strict)"(error in=w43, "Value"=FALSE ("Load arbitrary waveform")) -> ()  [unwired: 1 in, 2 out]
          }
        }
        n640 = local read "stop program"() -> (w39:bool)
      }
      n641 = while {
        stop <- w929 stop-if-true
        # "Nikon control"
        n642 = event shown="[13] \"Define 2\": Value Change" {
          selector: _ -> [_ _ _ _ _ _ _ _ _ _ _ _ _ _]
          dyn-events: _ -> [_ _ _ _ _ _ _ _ _ _ _ _ _ _]
          timeout: 50 -> [_ _ _ _ _ _ _ _ _ _ _ _ _ _]
          event Timeout {
            # "This part reads the info\nfrom the microscope\n(based on what as been \ndeclared at the beginning)"
            n643 = event-data() -> ()  [unwired: 1 in, 2 out]
            n644 = local read "Ti-E initialized"() -> (w931:bool)
            n645 = case shown="True" w931 {
              frame False {
              }
              frame True {
                n646 = local read "TiE Ref"() -> (w937:T21)
                n647 = property on="Home" class="Bool (strict)"() -> ("Value"=w935:bool)  [unwired: 2 in, 2 out]
                n648 = call "subTiE_GetStatus.vi"("Ref"=w937) -> ("TI-Ctrl"=w936:T40)
                n649 = Select(t=T23."Disabled and Grayed Out" ("Disabled"), s=w935, f=T23."Enabled" ("Disabled")) -> (s? t:f=w932:T23)
                n650 = local write "TI-Ctrl"(w936) -> ()
                n651 = property on="Z-pos" class="DigNum (strict)"("DisabledEnum"=w932) -> ()  [unwired: 2 in, 2 out]
              }
            }
          }
          event "Scope on?": Value Change {
            n652 = event-data() -> ("NewVal"=w940:bool)  [unwired: 1 in]
            n653 = case shown="True" w940 {
              tunnel: [T23."Disabled and Grayed Out" ("Disabled") T23."Enabled" ("Disabled")] -> w939
              tunnel: [FALSE ("Ti-E initialized") TRUE ("Ti-E initialized")] -> w938
              frame False {
                n654 = local read "TiE Ref"() -> (w941:T21)
                n655 = call "subTiE_Deinitialize.vi"("Ref"=w941) -> ()  [unwired: 11 in]
              }
              frame True {
                n656 = flat-sequence {
                  frame #0 {
                    n657 = property on="Status" class="Str"("Value"="Initializing Nikon ..." ("Status")) -> ()  [unwired: 2 in, 2 out]
                  }
                  frame #1 {
                    n658 = local read "log path"() -> (w947:path)
                    n659 = call "subTiE_Initialize.vi"("Ti Control Lib"="Ti Control Lib") -> ("Ref"=→"TiE Ref":T21)  [unwired: 10 in]
                    n660 = call "subRegist_AddInfoIntoText.vi"("log path"=w947, "info to be added"=" Ti-E") -> ()  [unwired: 10 in]
                  }
                  frame #2 {
                    n661 = property on="Status" class="Str"("Value"="Ready" ("Status")) -> ()  [unwired: 2 in, 2 out]
                  }
                }
              }
            }
            "Ti-E initialized" <- w938
            n662 = property on="TI-Ctrl" class="Clust (strict)"("DisabledEnum"=w939) -> ()  [unwired: 2 in, 2 out]
          }
          event "TI-Ctrl.Obj": Value Change {
            n663 = event-data() -> ()  [unwired: 1 in, 1 out]
            n664 = local read "TiE Ref"() -> (w952:T21)
            n665 = local read "TI-Ctrl"() -> (w954:T9)
            n666 = call "subTiE_SetZEscape.vi"("Ref"=w952, "TI-Ctrl"=w954) -> ("error out"=w953:errorcluster)  [unwired: 9 in]
            n667 = call "subTiE_SetObjective.vi"("TiE Ref"=w952, "TI-Ctrl"=w954, "error in"=w953) -> ()  [unwired: 8 in, 1 out]
          }
          event "TI-Ctrl.Lightpath": Value Change {
            # "Change this into subVI: \nsubTiE_SetLightpath"
            n668 = event-data() -> ()  [unwired: 1 in, 1 out]
            n669 = local read "TI-Ctrl"() -> (w959:T9)
            n670 = local read "TiE Ref"() -> (w958:T21)
            n671 = Unbundle By Name(w959) -> ("Lightpath"=w956:enum32{"EYE", "L100", "R100", "L80"})
            n672 = Unbundle By Name(w958) -> ("LightPathDrive"=w957:refnum<k7>)
            n673 = Increment(x=w956) -> (x+1=w955:enum32{"EYE", "L100", "R100", "L80"})
            n674 = To Variant(anything=w955) -> (Variant=w960:variant)
            n675 = property class="ILightPathDrive"(reference=w957, "Position"=w960) -> ()  [unwired: 1 in, 2 out]
          }
          event "TI-Ctrl.Z-Ctrl.Z-pos": Value Change {
            n676 = event-data() -> ()  [unwired: 1 in, 1 out]
            n677 = local read "TiE Ref"() -> (w961:T21)
            n678 = local read "TI-Ctrl"() -> (w962:T9)
            n679 = call "subTiE_SetZPos.vi"("Ref"=w961, "TI-Ctrl"=w962) -> ()  [unwired: 9 in, 1 out]
          }
          event "TI-Ctrl.Z-Ctrl.Sensitivity": Value Change {
            # "Change this into subVI: \nsubTiE_SetZSensitivity"
            n680 = event-data() -> ()  [unwired: 1 in, 1 out]
            n681 = local read "TI-Ctrl"() -> (w970:T9)
            n682 = local read "TiE Ref"() -> (w969:T21)
            n683 = Unbundle By Name(w970) -> ("Z-Ctrl.Sensitivity"=w964:u8)
            n684 = Unbundle By Name(w969) -> ("ZDrive"=w968:refnum<k7>)
            n685 = Decrement(x=w964) -> (x-1=w966:u8)
            n686 = Multiply(x=w966, y=u8 3) -> (x*y=w967:u8)
            n687 = Increment(x=w967) -> (x+1=w963:u8)
            n688 = To Variant(anything=w963) -> (Variant=w971:variant)
            n689 = property class="IZDrive"(reference=w968, "DialSensitivity"=w971) -> ()  [unwired: 1 in, 2 out]
          }
          event "TI-Ctrl.Z-Ctrl.Home": Value Change {
            # "Home = Escape"
            n690 = event-data() -> ()  [unwired: 1 in, 1 out]
            n691 = local read "TiE Ref"() -> (w973:T21)
            n692 = local read "TI-Ctrl"() -> (w972:T9)
            n693 = call "subTiE_SetZEscape.vi"("Ref"=w973, "TI-Ctrl"=w972) -> ()  [unwired: 9 in, 1 out]
          }
          event "TI-Ctrl.PFS-Ctrl.PFS IO": Value Change {
            # "Change this into subVI: \nsubTiE_SetPFSonOff"
            # "PFS Status\n1: PFS Possible\n2: tmp\n4,5: ON (no idea the difference)\n6: DIS\n7: NOT POSSIBLE"
            n694 = event-data() -> ()  [unwired: 1 in, 1 out]
            n695 = local read "TiE Ref"() -> (w975:T21)
            n696 = Unbundle By Name(w975) -> ("PFS"=w974:refnum<k7>)
            n697 = property class="IPFS"(reference=w974) -> (reference out=w979:refnum<k7>, "Status"=w977:variant, "IsEnabled"=w981:variant)  [unwired: 1 in, 1 out]
            n698 = Variant To Data(type=0, Variant=w977) -> (data=w978:i32)  [unwired: 1 in, 1 out]
            n699 = Variant To Data(type=0, Variant=w981) -> (data=w982:i32)  [unwired: 1 in, 1 out]
            n700 = case shown="1" w978 {
              tunnel: w979 -> [w983 _ w990]
              tunnel: w982 -> [_ _ _]
              frame Default {
                n701 = local read "TI-Ctrl"() -> (w985:T9)
                n702 = Unbundle By Name(w985) -> ("PFS-Ctrl.PFS IO"=w984:bool)
                n703 = case shown="False" w984 {
                  selector: w984 -> [w987 _]
                  tunnel: w983 -> [w986 _]
                  frame False {
                    n704 = Boolean To (0,1)(Boolean=w987) -> (0, 1=w989:i16)
                    n705 = To Variant(anything=w989) -> (Variant=w988:variant)
                    n706 = property class="IPFS"(reference=w986, "IsEnabled"=w988) -> ()  [unwired: 1 in, 2 out]
                  }
                  frame True {
                  }
                }
              }
              frame 7 {
              }
              frame 1 {
                n707 = local read "TI-Ctrl"() -> (w992:T9)
                n708 = Unbundle By Name(w992) -> ("PFS-Ctrl.PFS IO"=w991:bool)
                n709 = case shown="True" w991 {
                  selector: w991 -> [_ w994]
                  tunnel: w990 -> [_ w993]
                  frame False {
                  }
                  frame True {
                    n710 = Boolean To (0,1)(Boolean=w994) -> (0, 1=w996:i16)
                    n711 = To Variant(anything=w996) -> (Variant=w995:variant)
                    n712 = property class="IPFS"(reference=w993, "IsEnabled"=w995) -> ()  [unwired: 1 in, 2 out]
                  }
                }
              }
            }
          }
          event "TI-Ctrl.PFS-Ctrl.PSF Pos": Value Change {
            # "Change this into subVI: \nsubTiE_SetPFSpos"
            # "PFS Status\n1: PFS Possible\n2: tmp\n4,5: ON (no idea the difference)\n6: DIS\n7: NOT POSSIBLE"
            n713 = event-data() -> ()  [unwired: 1 in, 1 out]
            n714 = local read "TiE Ref"() -> (w998:T21)
            n715 = Unbundle By Name(w998) -> ("PFS"=w997:refnum<k7>)
            n716 = property class="IPFS"(reference=w997) -> (reference out=w1002:refnum<k7>, "Status"=w1000:variant)  [unwired: 1 in, 1 out]
            n717 = Variant To Data(type=0, Variant=w1000) -> (data=w1001:i32)  [unwired: 1 in, 1 out]
            n718 = case shown="4, 5" w1001 {
              tunnel: w1002 -> [_ w1006]
              frame Default {
              }
              frame 4, 5 {
                n719 = local read "TI-Ctrl"() -> (w1004:T9)
                n720 = Unbundle By Name(w1004) -> ("PFS-Ctrl.PSF Pos"=w1005:u32)
                n721 = To Variant(anything=w1005) -> (Variant=w1003:variant)
                n722 = property class="IPFS"(reference=w1006, "Position"=w1003) -> ()  [unwired: 1 in, 2 out]
              }
            }
          }
          event "TI-Ctrl.Condenser": Value Change {
            # "Change this into subVI: \nsubTiE_SetCondenser"
            n723 = event-data() -> ()  [unwired: 1 in, 1 out]
            n724 = local read "TiE Ref"() -> (w1009:T21)
            n725 = local read "TI-Ctrl"() -> (w1010:T9)
            n726 = Unbundle By Name(w1009) -> ("CondenserCassette"=w1008:refnum<k7>)
            n727 = Unbundle By Name(w1010) -> ("Condenser"=w1007:u16)
            n728 = To Variant(anything=w1007) -> (Variant=w1011:variant)
            n729 = property class="ICondenserCassette"(reference=w1008, "Position"=w1011) -> ()  [unwired: 1 in, 2 out]
          }
          event "TI-Ctrl.Cube Bottom": Value Change {
            n730 = event-data() -> ()  [unwired: 1 in, 1 out]
            n731 = local read "TI-Ctrl"() -> (w1012:T9)
            n732 = local read "TiE Ref"() -> (w1013:T21)
            n733 = call "subTiE_SetCubeBottom.vi"("Ref"=w1013, "TI-Ctrl"=w1012) -> ()  [unwired: 10 in]
          }
          event "TI-Ctrl.Cube Top": Value Change {
            n734 = event-data() -> ()  [unwired: 1 in, 1 out]
            n735 = local read "TI-Ctrl"() -> (w1014:T9)
            n736 = local read "TiE Ref"() -> (w1015:T21)
            n737 = call "subTiE_SetCubeTop.vi"("Ref"=w1015, "TI-Ctrl"=w1014) -> ()  [unwired: 10 in]
          }
          event "Define 1": Value Change {
            n738 = event-data() -> ()  [unwired: 1 in, 6 out]
            n739 = local write "Define 1"(FALSE) -> ()
            n740 = local read "TI-Ctrl"() -> (w1020:T9)
            n741 = Unbundle By Name(w1020) -> ("Z-Ctrl.Z-pos"=w1018:dbl)
            n742 = local read "Z-Stack"() -> (w1016:T10)
            n743 = Bundle By Name(cluster=w1016, "Z0"=w1018) -> (w1017:T10)
            n744 = local write "Z-Stack"(w1017) -> ()
          }
          event "Define 2": Value Change {
            n745 = event-data() -> ()  [unwired: 1 in, 6 out]
            n746 = local read "TI-Ctrl"() -> (w1025:T9)
            n747 = Unbundle By Name(w1025) -> ("Z-Ctrl.Z-pos"=w1023:dbl)
            n748 = local write "Define 2"(FALSE) -> ()
            n749 = local read "Z-Stack"() -> (w1022:T10)
            n750 = Bundle By Name(cluster=w1022, "Z end"=w1023) -> (w1021:T10)
            n751 = local write "Z-Stack"(w1021) -> ()
          }
        }
        n752 = local read "stop program"() -> (w929:bool)
      }
      n753 = property on="Confocal VISA Setting" class="VISAName"() -> ("Value"=w32:refnum<visa-resource-name>)  [unwired: 2 in, 2 out]
      n754 = while {
        shift-right: [w729] -> _
        shift-left: errorcluster {"status"=FALSE, "code"=0, "source"=""} ("Confocal") -> [w733]
        tunnel: w32 -> [w732]
        stop <- w730 stop-if-true
        # "Confocal scanner"
        n755 = event shown="[0] Timeout" {
          selector: _ -> [_ _ _ _ _ _ _]
          dyn-events: _ -> [_ _ _ _ _ _ _]
          timeout: 50 -> [_ _ _ _ _ _ _]
          tunnel: w733 -> [w736 w749 w765 w769 w773 w777 w781]
          tunnel: [w734 w745 w764 w768 w772 w776 w780] -> w729
          tunnel: w732 -> [w737 w750 w766 w770 w774 w778 w782]
          event Timeout {
            n756 = event-data() -> ()  [unwired: 1 in, 1 out]
            n757 = local read "SDC initialized"() -> (w735:bool)
            n758 = case shown="True" w735 {
              tunnel: w737 -> [_ w740]
              tunnel: w736 -> [w738 w742]
              tunnel: [w738 w741] -> w734
              frame False {
              }
              frame True {
                n759 = call "SubConfocal_GetInfo.vi"("Error In"=w742, "Confocal line (VISA IN)"=w740) -> ("Error out"=w741:errorcluster, "Confocal Info"=→"Confocal Info":T20)  [unwired: 8 in]
              }
            }
          }
          event "Confocal on?": Value Change {
            n760 = event-data() -> ("NewVal"=w748:bool)  [unwired: 1 in]
            n761 = case shown="True" w748 {
              tunnel: w750 -> [w754 w761]
              tunnel: w749 -> [w753 w760]
              tunnel: [w751 w759] -> w744
              tunnel: [T23."Disabled and Grayed Out" ("Disabled") T23."Enabled" ("Disabled")] -> w747
              tunnel: [T24 {"SDC shutter"=FALSE, "FWPosition"=3, "FW speed"=3, "Disk spinning?"=FALSE, "Disk speed (rpm)"=3000.0} ("Confocal scanner") w757] -> w746
              tunnel: [FALSE ("SDC initialized") TRUE ("SDC initialized")] -> w743
              frame False {
                n762 = call "SubConfocal_StartStop.vi"("Error In"=w753, "Confocal line (VISA IN)"=w754) -> ("Error out"=w751:errorcluster)  [unwired: 9 in]
              }
              frame True {
                n763 = local read "Confocal scanner"() -> (w757:T5)
                n764 = call "SubConfocal_StartStop.vi"("Confocal scanner"=w757, "Error In"=w760, "Confocal line (VISA IN)"=w761) -> ("Error out"=w759:errorcluster)  [unwired: 8 in]
              }
            }
            n765 = property on="Confocal scanner" class="Clust (strict)"("DisabledEnum"=w747) -> ()  [unwired: 2 in, 2 out]
            n766 = property on="Confocal scanner" class="Clust (strict)"("Value"=w746) -> ()  [unwired: 2 in, 2 out]
            n767 = property on="SDC initialized" class="Bool (strict)"(error in=w744, "Value"=w743) -> (error out=w745:errorcluster)  [unwired: 1 in, 1 out]
          }
          event "Confocal scanner.SDC shutter": Value Change {
            n768 = event-data() -> ()  [unwired: 1 in, 1 out]
            n769 = local read "Confocal scanner"() -> (w763:T5)
            n770 = call "SubConfocal_SetShutterStatus.vi"("Confocal scanner"=w763, "Error In"=w765, "Confocal line (VISA IN)"=w766) -> ("Error out"=w764:errorcluster)  [unwired: 7 in, 1 out]
          }
          event "Confocal scanner.Filter wheel": Value Change {
            n771 = event-data() -> ()  [unwired: 1 in, 1 out]
            n772 = local read "Confocal scanner"() -> (w767:T5)
            n773 = call "SubConfocal_SetFWpos.vi"("Confocal scanner"=w767, "Error In"=w769, "Confocal line (VISA IN)"=w770) -> ("Error out"=w768:errorcluster)  [unwired: 7 in, 1 out]
          }
          event "Confocal scanner.FW speed": Value Change {
            n774 = event-data() -> ()  [unwired: 1 in, 1 out]
            n775 = local read "Confocal scanner"() -> (w771:T5)
            n776 = call "SubConfocal_SetFWSpeed.vi"("Confocal scanner"=w771, "Error In"=w773, "Confocal line  (VISA IN)"=w774) -> ("Error out"=w772:errorcluster)  [unwired: 7 in, 1 out]
          }
          event "Confocal scanner.Disk spinning": Value Change {
            n777 = event-data() -> ()  [unwired: 1 in, 1 out]
            n778 = local read "Confocal scanner"() -> (w775:T5)
            n779 = call "SubConfocal_DiskSpinningOnOff.vi"("Confocal scanner"=w775, "Error In"=w777, "Confocal line (VISA IN)"=w778) -> ("Error out"=w776:errorcluster)  [unwired: 7 in, 1 out]
          }
          event "Confocal scanner.Disk speed (rpm)": Value Change {
            n780 = event-data() -> ()  [unwired: 1 in, 1 out]
            n781 = local read "Confocal scanner"() -> (w779:T5)
            n782 = call "SubConfocal_SetDiskSpinningSpeed.vi"("Confocal scanner"=w779, "Error In"=w781, "Confocal line (VISA IN)"=w782) -> ("Error out"=w780:errorcluster)  [unwired: 7 in, 1 out]
          }
        }
        "Confocal" <- w729
        n783 = local read "stop program"() -> (w730:bool)
      }
    }
    frame #2 {
      # "Close camera, stage, and deinitialize"
      n784 = flat-sequence {
        frame #0 {
          n785 = local read "Camera on?"() -> (w1063:bool)
          n786 = local read "Confocal on?"() -> (w1065:bool)
          n787 = local read "Stage on?"() -> (w1064:bool)
          n788 = case shown="True" w1063 {
            tunnel: errorcluster {"status"=FALSE, "code"=0, "source"=""} ("error in (no error)") -> [w1067 w1071]
            tunnel: [w1067 w1070] -> w1062
            frame False {
            }
            frame True {
              n789 = property on="Handle" class="DigNum (strict)"() -> ("Value"=w1068:u32)  [unwired: 2 in, 2 out]
              n790 = property on="Live" class="Bool (strict)"() -> ("Value"=w1069:bool)  [unwired: 2 in, 2 out]
              n791 = call "subHamamatsu_TurnOnOff.vi"("logic 2"=FALSE, "logic 1"=w1069, "error in (no error)"=w1071, "Handle in"=w1068) -> ("error out"=w1073:errorcluster, "Handle out"=w1072:u32)  [unwired: 5 in, 1 out]
              n792 = call "subHamamatsu_Deinitialization.vi"("error in (no error)"=w1073, "Handle"=w1072) -> ("error out"=w1070:errorcluster)  [unwired: 9 in]
            }
          }
          n793 = case shown="True" w1064 {
            frame False {
            }
            frame True {
              n794 = local read "Stage Status"() -> (w1076:T7)
              n795 = call "Disconnect.vi"("Stage Info"=w1076) -> ()  [unwired: 10 in, 1 out]
              n796 = property on="Stage Status" class="Clust (strict)"("Value"=T7 {" Current Position"=[-1.0, -12.0, 0.0], "Number of Axis"=3, "ILSID"=1} ("Stage Info")) -> ()  [unwired: 2 in, 2 out]
            }
          }
          n797 = case shown="True" w1065 {
            frame False {
            }
            frame True {
              n798 = property on="Confocal VISA Setting" class="VISAName"() -> ("Value"=w1077:refnum<visa-resource-name>)  [unwired: 2 in, 2 out]
              n799 = call "SubConfocal_StartStop.vi"("Confocal line (VISA IN)"=w1077) -> ()  [unwired: 10 in, 1 out]
              n800 = property on="Confocal scanner" class="Clust (strict)"("Value"=T5 {"SDC shutter"=FALSE, "Filter wheel"=3, "FW speed"=3, "Disk spinning"=FALSE, "Disk speed (rpm)"=3000.0} ("Confocal scanner")) -> ()  [unwired: 2 in, 2 out]
            }
          }
          n801 = property on="DAQ ports" class="Clust (strict)"() -> ("Value"=w1058:T25)  [unwired: 2 in, 2 out]
          n802 = call "subDAQ_SetLaserDO.vi"("DAQ ports"=w1058) -> ("Error out"=w1059:errorcluster)  [unwired: 10 in]
          n803 = local write "Camera"(w1062) -> ()
          n804 = call "subDAQ_SetLED.vi"("DAQ ports"=w1058, "Error in (no error)"=w1059) -> ()  [unwired: 9 in, 1 out]
          n805 = local read "Scope on?"() -> (w1060:bool)
          n806 = case shown="True" w1060 {
            frame False {
            }
            frame True {
              n807 = local read "TiE Ref"() -> (w1066:T21)
              n808 = call "subTiE_Deinitialize.vi"("Ref"=w1066) -> ()  [unwired: 11 in]
            }
          }
        }
        frame #1 {
          w1079 = FALSE ("stop program")
          w1083 = "\t"
          n809 = local read "log path"() -> (w1080:path)
          n810 = local write "Camera initialized"(bool[] [FALSE, FALSE] ("Camera initialized")) -> ()
          n811 = local write "Stage on?"(w1079) -> ()
          n812 = local write "Scope on?"(w1079) -> ()
          n813 = local write "Confocal on?"(w1079) -> ()
          n814 = local write "Camera on?"(w1079) -> ()
          n815 = local write "Stage initialized"(w1079) -> ()
          n816 = local write "Ti-E initialized"(w1079) -> ()
          n817 = local write "SDC initialized"(w1079) -> ()
          n818 = local write "stop program"(w1079) -> ()
          n819 = Format Date/Time String(time format string (%c)="%X") -> (date/time string=w1082:string)  [unwired: 2 in]
          n820 = Read from Text File(file (use dialog)=w1080) -> (refnum out=w1087:refnum<file>, text=w1085:string)  [unwired: 3 in, 2 out]
          n821 = Concatenate Strings(w1085, "\r", w1083, w1083, w1083, w1083, w1082) -> (w1086:string)
          n822 = Close File(refnum=w1087) -> (path=w1088:path)  [unwired: 1 in, 1 out]
          n823 = property on="Live" class="Bool (strict)"("Value"=w1079) -> ()  [unwired: 2 in, 2 out]
          n824 = Write to Text File(file (use dialog)=w1088, text=w1086) -> ()  [unwired: 2 in, 3 out]
        }
      }
    }
  }
